vi "Lab Panel V3.2.vi"() -> ()   [LabVIEW 2013]
uses:
  <vilib>/Platform/TimedLoop/XDataNode/timing_clust.ctl
  <vilib>/Platform/TimedLoop/XDataNode/nitl_modes.ctl
  <vilib>/Platform/TimedLoop/XDataNode/wakeup.ctl
  Global 1.vi
  <vilib>/platform/TimedLoop/XDataNode/XDataNode.xnode
  <vilib>/Platform/TimedLoop/XDataNode/XDNodeRunTimeDep.lvlib
panel:
  out "TEMP update":bool
  out "AI update":bool
  in  "stop":bool
  in  "Tab Control 2":T1(tab)
  out "SIG LAB05-2":T2 {"PF" format="%.2f"; "AMPS" format="%.1f"}
  out "SIG LAB05-1":T2 {"PF" format="%.2f"; "AMPS" format="%.1f"}
  out "SIG LAB04-2":T2 {"PF" format="%.2f"; "AMPS" format="%.1f"}
  out "SIG LAB04-1":T2 {"PF" format="%.2f"; "AMPS" format="%.1f"}
  out "SIG LAB03-2":T2 {"PF" format="%.2f"; "AMPS" format="%.1f"}
  out "SIG LAB03-1":T2 {"PF" format="%.2f"; "AMPS" format="%.1f"}
  out "SIG LAB02-2":T2 {"PF" format="%.2f"; "AMPS" format="%.1f"}
  in  "RUN LAB01-1":bool
  in  "O/I  LAB05-1":bool
  in  "O/I  LAB05-2":bool
  in  "O/I  LAB04-1":bool
  in  "O/I  LAB04-2":bool
  in  "O/I  LAB02-1":bool
  in  "O/1  LAB02-2":bool
  in  "O/I  LAB01-2":bool
  in  "O/I  LAB01-1":bool
  in  "O/I  LAB03-1":bool
  in  "RUN LAB05-2":bool
  in  "RUN LAB05-1":bool
  in  "RUN LAB04-2":bool
  in  "RUN LAB04-1":bool
  in  "RUN LAB03-2":bool
  in  "RUN LAB03-1":bool
  in  "RUN LAB02-2":bool
  in  "RUN LAB02-1":bool
  in  "RUN LAB01-2":bool
  in  "SELECT LAB05-2":T3(radio)
  in  "SELECT LAB05-1":T3(radio)
  in  "SELECT LAB04-2":T3(radio)
  in  "SELECT LAB04-1":T3(radio)
  in  "SELECT LAB03-2":T3(radio)
  in  "SELECT LAB03-1":T3(radio)
  in  "SELECT LAB02-2":T3(radio)
  in  "SELECT LAB02-1":T3(radio)
  in  "SELECT LAB01-2":T3(radio)
  in  "SELECT LAB01-1":T3(radio)
  in  "O/I  LAB03-2":bool
  out "SIG LAB01-1":T2 {"PF" format="%.2f"; "AMPS" format="%.1f"}
  out "SIG LAB01-2":T2 {"PF" format="%.2f"; "AMPS" format="%.1f"}
  out "SIG LAB02-1":T2 {"PF" format="%.2f"; "AMPS" format="%.1f"}
  out "DISP LAB05-2":T4 {"MINS" format="%.2g"}
  out "DISP LAB05-1":T4 {"MINS" format="%.2g"}
  out "DISP LAB04-2":T4 {"MINS" format="%.2g"}
  out "DISP LAB04-1":T4 {"MINS" format="%.2g"}
  out "DISP LAB03-2":T4 {"MINS" format="%.2g"}
  out "DISP LAB03-1":T4 {"MINS" format="%.2g"}
  in  "SET LAB05-2":T5={"NAME"="", "DESCRIPTION"="", "CYCLES"=5.0, "T-RISE mins"=0.0, "T-RISE deg C"=0.0} {"CYCLES" min=5.0 step=1.0}
  in  "SET LAB05-1":T5={"NAME"="", "DESCRIPTION"="", "CYCLES"=5.0, "T-RISE mins"=0.0, "T-RISE deg C"=0.0} {"CYCLES" min=5.0 step=1.0}
  in  "SET LAB04-2":T5={"NAME"="", "DESCRIPTION"="", "CYCLES"=5.0, "T-RISE mins"=0.0, "T-RISE deg C"=0.0} {"CYCLES" min=5.0 step=1.0}
  in  "SET LAB04-1":T5={"NAME"="", "DESCRIPTION"="", "CYCLES"=5.0, "T-RISE mins"=0.0, "T-RISE deg C"=0.0} {"CYCLES" min=5.0 step=1.0}
  in  "SET LAB03-2":T5={"NAME"="", "DESCRIPTION"="", "CYCLES"=5.0, "T-RISE mins"=0.0, "T-RISE deg C"=0.0} {"CYCLES" min=5.0 step=1.0}
  in  "SET LAB03-1":T5={"NAME"="", "DESCRIPTION"="", "CYCLES"=5.0, "T-RISE mins"=0.0, "T-RISE deg C"=0.0} {"CYCLES" min=5.0 step=1.0}
  out "DISP LAB02-2":T4 {"MINS" format="%.2g"}
  out "DISP LAB02-1":T4 {"MINS" format="%.2g"}
  in  "SET LAB02-2":T5={"NAME"="", "DESCRIPTION"="", "CYCLES"=5.0, "T-RISE mins"=0.0, "T-RISE deg C"=0.0} {"CYCLES" min=5.0 step=1.0}
  in  "SET LAB02-1":T5={"NAME"="", "DESCRIPTION"="", "CYCLES"=5.0, "T-RISE mins"=0.0, "T-RISE deg C"=0.0} {"CYCLES" min=5.0 step=1.0}
  out "RESULT LAB05-2":bool
  out "RESULT LAB05-1":bool
  out "RESULT LAB04-2":bool
  out "RESULT LAB04-1":bool
  out "RESULT LAB03-2":bool
  out "RESULT LAB03-1":bool
  out "RESULT LAB02-2":bool
  out "RESULT LAB02-1":bool
  out "RESULT LAB01-2":bool
  out "RESULT LAB01-1":bool
  in  "SET LAB01-1":T5={"NAME"="", "DESCRIPTION"="", "CYCLES"=5.0, "T-RISE mins"=0.0, "T-RISE deg C"=0.0} {"CYCLES" min=5.0 step=1.0}
  in  "SET LAB01-2":T5={"NAME"="", "DESCRIPTION"="", "CYCLES"=5.0, "T-RISE mins"=0.0, "T-RISE deg C"=0.0} {"CYCLES" min=5.0 step=1.0}
  out "DISP LAB01-1":T4 {"MINS" format="%.2g"}
  out "DISP LAB01-2":T4 {"MINS" format="%.2f"}
  in  "Mail Report Error":errorcluster
  in  "MAIL SELECT":cluster{"Mail Notification":bool, "TO:":string}
  in  "Network Directory":path
  in  "JIG OFF TIME (S)":dbl=2.0 min=2.0 max=10.0 step=0.5 format="%.1g"
  in  "JIG ON TIME (S)":dbl=1.0 min=1.0 max=10.0 step=0.5 format="%.1g"
  out "FAIL LAB05-2":cluster{"LO":dbl, "HI":dbl}
  out "FAIL LAB05-1":cluster{"LO":dbl, "HI":dbl}
  out "FAIL LAB04-2":cluster{"LO":dbl, "HI":dbl}
  out "FAIL LAB04-1":cluster{"LO":dbl, "HI":dbl}
  out "FAIL LAB03-2":cluster{"LO":dbl, "HI":dbl}
  out "FAIL LAB03-1":cluster{"LO":dbl, "HI":dbl}
  out "FAIL LAB02-2":cluster{"LO":dbl, "HI":dbl}
  out "FAIL LAB02-1":cluster{"LO":dbl, "HI":dbl}
  out "FAIL LAB01-2":cluster{"LO":dbl, "HI":dbl}
  out "FAIL LAB01-1":cluster{"LO":dbl, "HI":dbl}
  out "TEMP START LAB05-2":cluster{"TL":dbl, "TN":dbl}
  out "TEMP START LAB04-2":cluster{"TL":dbl, "TN":dbl}
  out "TEMP START LAB03-2":cluster{"TL":dbl, "TN":dbl}
  out "TEMP START LAB02-2":cluster{"TL":dbl, "TN":dbl}
  out "TEMP START LAB01-2":cluster{"TL":dbl, "TN":dbl}
  out "TEMP START LAB05-1":cluster{"TL":dbl, "TN":dbl}
  out "TEMP START LAB04-1":cluster{"TL":dbl, "TN":dbl}
  out "TEMP START LAB03-1":cluster{"TL":dbl, "TN":dbl}
  out "TEMP START LAB02-1":cluster{"TL":dbl, "TN":dbl}
  out "TEMP START LAB01-1":cluster{"TL":dbl, "TN":dbl}
  out "JIG LAB01-1":bool
  out "JIG LAB01-2":bool
  out "JIG LAB02-1":bool
  out "JIG LAB02-2":bool
  out "JIG LAB03-1":bool
  out "JIG LAB03-2":bool
  out "JIG LAB04-1":bool
  out "JIG LAB04-2":bool
  out "JIG LAB05-1":bool
  out "JIG LAB05-2":bool
  out "CAL LAB01":T6 {"2 (TN) cal" min=0.0 step=0.01 format="%.2f"; "2 (TL) cal" min=0.0 step=0.01 format="%.2f"; "2 (PF) cal" min=0.0 step=0.01 format="%.2f"; "2 (V) cal" min=0.0 step=0.01 format="%.2f"; "2 (A) cal" min=0.0 step=0.01 format="%.2f"; "1 (TN) cal" min=0.0 step=0.01 format="%.2f"; "1 (TL) cal" min=0.0 step=0.01 format="%.2f"; "1 (PF) cal" min=0.0 step=0.01 format="%.2f"; "1 (V) cal" min=0.0 step=0.01 format="%.2f"; "1  (A) cal" min=0.0 step=0.01 format="%.2f"}
  out "CAL LAB03":T6 {"2 (TN) cal" min=0.0 step=0.01 format="%.2f"; "2 (TL) cal" min=0.0 step=0.01 format="%.2f"; "2 (PF) cal" min=0.0 step=0.01 format="%.2f"; "2 (V) cal" min=0.0 step=0.01 format="%.2f"; "2 (A) cal" min=0.0 step=0.01 format="%.2f"; "1 (TN) cal" min=0.0 step=0.01 format="%.2f"; "1 (TL) cal" min=0.0 step=0.01 format="%.2f"; "1 (PF) cal" min=0.0 step=0.01 format="%.2f"; "1 (V) cal" min=0.0 step=0.01 format="%.2f"; "1  (A) cal" min=0.0 step=0.01 format="%.2f"}
  out "CAL LAB02":T7 {"2 (TN) cal" min=0.0 step=0.01 format="%.2f"; "2 (TL) cal" min=0.0 step=0.01 format="%.2f"; "2 (PF) cal" min=0.0 step=0.01 format="%.2f"; "2 (V) cal" min=0.0 step=0.01 format="%.2f"; "2 (A) cal" min=0.0 step=0.01 format="%.2f"; "1 (TN) cal" min=0.0 step=0.01 format="%.2f"; "1 (TL) cal" min=0.0 step=0.01 format="%.2f"; "1 (PF) cal" min=0.0 step=0.01 format="%.2f"; "1 (V) cal" min=0.0 step=0.01 format="%.2f"; "1 (A) cal" min=0.0 step=0.01 format="%.2f"}
  out "CAL LAB05":T6 {"2 (TN) cal" min=0.0 step=0.01 format="%.2f"; "2 (TL) cal" min=0.0 step=0.01 format="%.2f"; "2 (PF) cal" min=0.0 step=0.01 format="%.2f"; "2 (V) cal" min=0.0 step=0.01 format="%.2f"; "2 (A) cal" min=0.0 step=0.01 format="%.2f"; "1 (TN) cal" min=0.0 step=0.01 format="%.2f"; "1 (TL) cal" min=0.0 step=0.01 format="%.2f"; "1 (PF) cal" min=0.0 step=0.01 format="%.2f"; "1 (V) cal" min=0.0 step=0.01 format="%.2f"; "1  (A) cal" min=0.0 step=0.01 format="%.2f"}
  out "CAL LAB04":T6 {"2 (TN) cal" min=0.0 step=0.01 format="%.2f"; "2 (TL) cal" min=0.0 step=0.01 format="%.2f"; "2 (PF) cal" min=0.0 step=0.01 format="%.2f"; "2 (V) cal" min=0.0 step=0.01 format="%.2f"; "2 (A) cal" min=0.0 step=0.01 format="%.2f"; "1 (TN) cal" min=0.0 step=0.01 format="%.2f"; "1 (TL) cal" min=0.0 step=0.01 format="%.2f"; "1 (PF) cal" min=0.0 step=0.01 format="%.2f"; "1 (V) cal" min=0.0 step=0.01 format="%.2f"; "1  (A) cal" min=0.0 step=0.01 format="%.2f"}
  out "calibration file error out":errorcluster
  in  "CALIBRATE":bool
  in  "MAIL SETTINGS":T8
  out "mail control":string
  out "MAIL REPORT":string
  out "stop2":bool
  in  "Tab Control":T9(tab)
  out "LAB01-2 (GRAPH)":dynamicdata(graph)
  out "LAB01-1 (GRAPH)":dynamicdata(graph)
  out "LAB02-2 (GRAPH)":dynamicdata(graph)
  out "LAB02-1 (GRAPH)":dynamicdata(graph)
  out "LAB03-2 (GRAPH)":dynamicdata(graph)
  out "LAB03-1 (GRAPH)":dynamicdata(graph)
  out "LAB04-2 (GRAPH)":dynamicdata(graph)
  out "LAB04-1 (GRAPH)":dynamicdata(graph)
  out "LAB05-2 (GRAPH)":dynamicdata(graph)
  out "LAB05-1 (GRAPH)":dynamicdata(graph)
  out "LAB05 TEMP":T10
  out "LAB04 TEMP":T10
  out "LAB02 TEMP":T10
  out "LAB01 TEMP":T10
  out "LAB03 TEMP":T10
  out "Analog Error Array":errorcluster[](array[cluster])
  out "AI loop time":dbl format="%.6g"
  out "loops":dbl
  in  "loop  delay(mS)":dbl
  out "on loops":dbl
  out "off loops":dbl
  out "jig cycle":dbl
  out "TDMS LAB01-1":refnum<k34>
  out "data file error":errorcluster
  out "TDMS LAB02-1":refnum<k34>
  out "TDMS LAB01-2":refnum<k34>
  out "TDMS LAB02-2":refnum<k34>
  out "TDMS LAB03-1":refnum<k34>
  out "TDMS LAB03-2":refnum<k34>
  out "TDMS LAB04-1":refnum<k34>
  out "TDMS LAB04-2":refnum<k34>
  out "TDMS LAB05-1":refnum<k34>
  out "TDMS LAB05-2":refnum<k34>
  # "LAB01"
  # "LAB02"
  # "LAB05"
  # "LAB03"
  # "LAB04"
  # "LAB01"
  # "LAB02"
  # "LAB03"
  # "LAB04"
  # "LAB05"
  # "JIG SET"
  # "Enter receipients address seperated by comma."
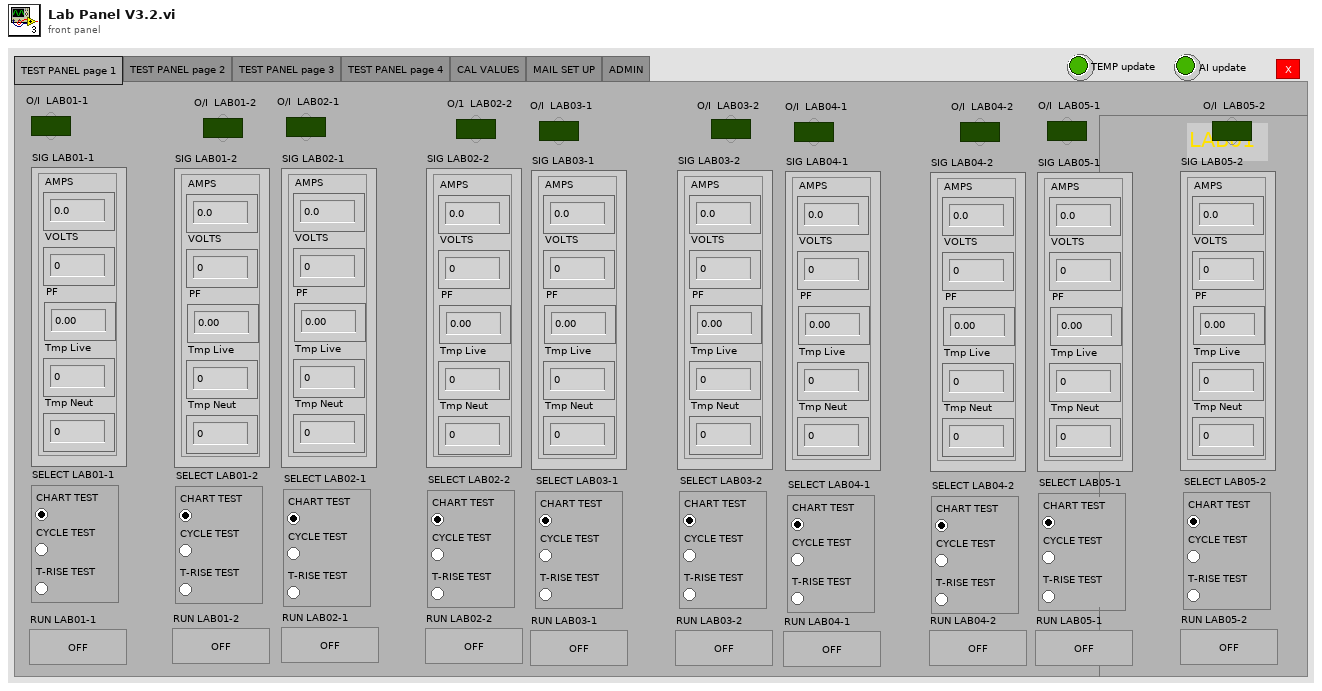
[diagram p1: front panel]
types:
  T1 = enum32{"TEST PANEL page 1", "TEST PANEL page 2", "TEST PANEL page 3", "TEST PANEL page 4", "CAL VALUES", "MAIL SET UP", "ADMIN"}
  T2 = cluster{"AMPS":dbl, "VOLTS":dbl, "PF":dbl, "Tmp Live":dbl, "Tmp Neut":dbl}
  T3 = enum32{"CHART TEST", "CYCLE TEST", "T-RISE TEST"}
  T4 = cluster{"CYCLE":dbl, "MINS":dbl, "STATUS":string}
  T5 = cluster{"NAME":string, "DESCRIPTION":string, "CYCLES":dbl, "T-RISE mins":dbl, "T-RISE deg C":dbl}
  T6 = cluster{"1  (A) cal":dbl, "1 (V) cal":dbl, "1 (PF) cal":dbl, "1 (TL) cal":dbl, "1 (TN) cal":dbl, "2 (A) cal":dbl, "2 (V) cal":dbl, "2 (PF) cal":dbl, "2 (TL) cal":dbl, "2 (TN) cal":dbl}
  T7 = cluster{"1 (A) cal":dbl, "1 (V) cal":dbl, "1 (PF) cal":dbl, "1 (TL) cal":dbl, "1 (TN) cal":dbl, "2 (A) cal":dbl, "2 (V) cal":dbl, "2 (PF) cal":dbl, "2 (TL) cal":dbl, "2 (TN) cal":dbl}
  T8 = cluster{"OUT SERVER ADDRESS":string, "FROM ACCOUNT":string, "USER NAME":string, "PASSWORD":string, "TEST MAIL":bool, "TEST MAIL STATUS":string, "mail error":errorcluster}
  T9 = enum32{"LAB01", "LAB02", "LAB03", "LAB04", "LAB05", "TEMPERATURE", "ERROR"}
  T10 = cluster{"T1 Live":dbl, "T1 Neut":dbl, "T2 Live":dbl, "T2 Neut":dbl, "ID":dbl, "ER":dbl}
  T11 = enum8{"Enabled", "Disabled", "Disabled and Grayed Out"}
  T12 = typedef "XDNodeRunTimeDep.lvlib/timing_clust.ctl" = cluster{"Expected End [f-1]":u64, "Actual End [f-1]":u64, "Finished Late? [f-1]":bool, "Expected End [i-1]":u64, "Actual End [i-1]":u64, "Finished Late? [i-1]":bool, "Expected Start [i]":u64, "Actual Start [i]":u64, "Expected Start [f]":u64, "Actual Start [f]":u64, "Source Name":string, "Structure Name":string, "Period":i64, "Deadline":i64, "Offset":i64, "Start":i64, "Priority":i32, "Timeout":i32, "Mode":T13, "Wakeup Reason":T14, "Error":errorcluster, "Source Type":string, "Secondary Source Type":string, "Global End Time":u64, "Global Start Time":u64, "Frame Duration":u64, "Iteration Duration":u64, "Assigned CPU":i32, "I/O Scan Engine Mode":u32}
  T13 = typedef "XDNodeRunTimeDep.lvlib/nitl_modes.ctl" = enum32{"No Change", "Process missed periods, maintain original phase", "Discard missed periods, maintain original phase", "Process missed periods, ignore original phase", "Discard missed periods, ignore original phase"}
  T14 = typedef "XDNodeRunTimeDep.lvlib/wakeup.ctl" = enum32{"Normal", "Aborted", "Asynchronous wakeup", "Timing source error", "Timed loop error", "Timeout"}
  T15 = enum16{"open", "open or create", "create or replace", "create", "open (read-only)"}
  T16 = enum16{"open", "replace", "create", "open or create", "replace or create", "replace or create with confirmation"}
  T17 = cluster{"SET LAB01-1":cluster{"NAME":string, "DESCRIPTION":string, "CYCLES":dbl, "T-RISE mins":dbl, "T-RISE deg C":dbl}, "SET LAB01-2":cluster{"NAME":string, "DESCRIPTION":string, "CYCLES":dbl, "T-RISE mins":dbl, "T-RISE deg C":dbl}, "SET LAB02-1":cluster{"NAME":string, "DESCRIPTION":string, "CYCLES":dbl, "T-RISE mins":dbl, "T-RISE deg C":dbl}, "SET LAB02-2":cluster{"NAME":string, "DESCRIPTION":string, "CYCLES":dbl, "T-RISE mins":dbl, "T-RISE deg C":dbl}, "SET LAB03-1":cluster{"NAME":string, "DESCRIPTION":string, "CYCLES":dbl, "T-RISE mins":dbl, "T-RISE deg C":dbl}, "SET LAB03-2":cluster{"NAME":string, "DESCRIPTION":string, "CYCLES":dbl, "T-RISE mins":dbl, "T-RISE deg C":dbl}, "SET LAB04-1":cluster{"NAME":string, "DESCRIPTION":string, "CYCLES":dbl, "T-RISE mins":dbl, "T-RISE deg C":dbl}, "SET LAB04-2":cluster{"NAME":string, "DESCRIPTION":string, "CYCLES":dbl, "T-RISE mins":dbl, "T-RISE deg C":dbl}, "SET LAB05-1":cluster{"NAME":string, "DESCRIPTION":string, "CYCLES":dbl, "T-RISE mins":dbl, "T-RISE deg C":dbl}, "SET LAB05-2":cluster{"NAME":string, "DESCRIPTION":string, "CYCLES":dbl, "T-RISE mins":dbl, "T-RISE deg C":dbl}, "Network Directory":path}
  T18 = cluster{"MAIL SETTINGS":cluster{"OUT SERVER ADDRESS":string, "FROM ACCOUNT":string, "USER NAME":string, "PASSWORD":string, "TEST MAIL":bool, "TEST MAIL STATUS":string, "mail error":errorcluster}, "MAIL SELECT":cluster{"Mail Notification":bool, "TO:":string}}
  T19 = cluster{"T1":dbl, "T2":dbl, "T3":dbl, "T4":dbl, "ID":dbl, "ER":dbl}
  T20 = cluster{"LAB01-1 (A)":dbl, "LAB01-1 (V)":dbl, "LAB01-1 (PF)":dbl, "LAB01-2 (A)":dbl, "LAB01-2 (V)":dbl, "LAB01-2 (PF)":dbl}
  T21 = cluster{"LAB02-1 (A)":dbl, "LAB02-1 (V)":dbl, "LAB02-1 (PF)":dbl, "LAB02-2 (A)":dbl, "LAB02-2 (V)":dbl, "LAB02-2 (PF)":dbl}
  T22 = cluster{"LAB03-1 (A)":dbl, "LAB03-1 (V)":dbl, "LAB03-1 (PF)":dbl, "LAB03-2 (A)":dbl, "LAB03-2 (V)":dbl, "LAB03-2 (PF)":dbl}
  T23 = cluster{"LAB04-1 (A)":dbl, "LAB04-1 (V)":dbl, "LAB04-1 (PF)":dbl, "LAB04-2 (A)":dbl, "LAB04-2 (V)":dbl, "LAB04-2 (PF)":dbl}
  T24 = cluster{"LAB05-1 (A)":dbl, "LAB05-1 (V)":dbl, "LAB05-1 (PF)":dbl, "LAB05-2 (A)":dbl, "LAB05-2 (V)":dbl, "LAB05-2 (PF)":dbl}
  T25 = cluster{"FAIL LAB01-1":cluster{"LO":dbl, "HI":dbl}, "SIG LAB01-1":cluster{"AMPS":dbl, "VOLTS":dbl, "PF":dbl, "Tmp Live":dbl, "Tmp Neut":dbl}, "TEMP START LAB01-1":cluster{"TL":dbl, "TN":dbl}, "DISP LAB01-1":cluster{"CYCLE":dbl, "MINS":dbl, "STATUS":string}, "SET LAB01-1":cluster{"NAME":string, "DESCRIPTION":string, "CYCLES":dbl, "T-RISE mins":dbl, "T-RISE deg C":dbl}, "TDMS LAB01-1":refnum<k34>}
  T26 = cluster{"FAIL LAB01-2":cluster{"LO":dbl, "HI":dbl}, "SIG LAB01-2":cluster{"AMPS":dbl, "VOLTS":dbl, "PF":dbl, "Tmp Live":dbl, "Tmp Neut":dbl}, "TEMP START LAB01-2":cluster{"TL":dbl, "TN":dbl}, "DISP LAB01-2":cluster{"CYCLE":dbl, "MINS":dbl, "STATUS":string}, "SET LAB01-2":cluster{"NAME":string, "DESCRIPTION":string, "CYCLES":dbl, "T-RISE mins":dbl, "T-RISE deg C":dbl}, "TDMS LAB01-2":refnum<k34>}
  T27 = cluster{"FAIL LAB02-1":cluster{"LO":dbl, "HI":dbl}, "SIG LAB02-1":cluster{"AMPS":dbl, "VOLTS":dbl, "PF":dbl, "Tmp Live":dbl, "Tmp Neut":dbl}, "TEMP START LAB02-1":cluster{"TL":dbl, "TN":dbl}, "DISP LAB02-1":cluster{"CYCLE":dbl, "MINS":dbl, "STATUS":string}, "SET LAB02-1":cluster{"NAME":string, "DESCRIPTION":string, "CYCLES":dbl, "T-RISE mins":dbl, "T-RISE deg C":dbl}, "TDMS LAB02-1":refnum<k34>}
  T28 = cluster{"FAIL LAB02-2":cluster{"LO":dbl, "HI":dbl}, "SIG LAB02-2":cluster{"AMPS":dbl, "VOLTS":dbl, "PF":dbl, "Tmp Live":dbl, "Tmp Neut":dbl}, "TEMP START LAB02-2":cluster{"TL":dbl, "TN":dbl}, "DISP LAB02-2":cluster{"CYCLE":dbl, "MINS":dbl, "STATUS":string}, "SET LAB02-2":cluster{"NAME":string, "DESCRIPTION":string, "CYCLES":dbl, "T-RISE mins":dbl, "T-RISE deg C":dbl}, "TDMS LAB02-2":refnum<k34>}
  T29 = cluster{"FAIL LAB03-1":cluster{"LO":dbl, "HI":dbl}, "SIG LAB03-1":cluster{"AMPS":dbl, "VOLTS":dbl, "PF":dbl, "Tmp Live":dbl, "Tmp Neut":dbl}, "TEMP START LAB03-1":cluster{"TL":dbl, "TN":dbl}, "DISP LAB03-1":cluster{"CYCLE":dbl, "MINS":dbl, "STATUS":string}, "SET LAB03-1":cluster{"NAME":string, "DESCRIPTION":string, "CYCLES":dbl, "T-RISE mins":dbl, "T-RISE deg C":dbl}, "TDMS LAB03-1":refnum<k34>}
  T30 = cluster{"FAIL LAB03-2":cluster{"LO":dbl, "HI":dbl}, "SIG LAB03-2":cluster{"AMPS":dbl, "VOLTS":dbl, "PF":dbl, "Tmp Live":dbl, "Tmp Neut":dbl}, "TEMP START LAB03-2":cluster{"TL":dbl, "TN":dbl}, "DISP LAB03-2":cluster{"CYCLE":dbl, "MINS":dbl, "STATUS":string}, "SET LAB03-2":cluster{"NAME":string, "DESCRIPTION":string, "CYCLES":dbl, "T-RISE mins":dbl, "T-RISE deg C":dbl}, "TDMS LAB03-2":refnum<k34>}
  T31 = cluster{"FAIL LAB04-1":cluster{"LO":dbl, "HI":dbl}, "SIG LAB04-1":cluster{"AMPS":dbl, "VOLTS":dbl, "PF":dbl, "Tmp Live":dbl, "Tmp Neut":dbl}, "TEMP START LAB04-1":cluster{"TL":dbl, "TN":dbl}, "DISP LAB04-1":cluster{"CYCLE":dbl, "MINS":dbl, "STATUS":string}, "SET LAB04-1":cluster{"NAME":string, "DESCRIPTION":string, "CYCLES":dbl, "T-RISE mins":dbl, "T-RISE deg C":dbl}, "TDMS LAB04-1":refnum<k34>}
  T32 = cluster{"FAIL LAB04-2":cluster{"LO":dbl, "HI":dbl}, "SIG LAB04-2":cluster{"AMPS":dbl, "VOLTS":dbl, "PF":dbl, "Tmp Live":dbl, "Tmp Neut":dbl}, "TEMP START LAB04-2":cluster{"TL":dbl, "TN":dbl}, "DISP LAB04-2":cluster{"CYCLE":dbl, "MINS":dbl, "STATUS":string}, "SET LAB04-2":cluster{"NAME":string, "DESCRIPTION":string, "CYCLES":dbl, "T-RISE mins":dbl, "T-RISE deg C":dbl}, "TDMS LAB04-2":refnum<k34>}
  T33 = cluster{"FAIL LAB05-1":cluster{"LO":dbl, "HI":dbl}, "SIG LAB05-1":cluster{"AMPS":dbl, "VOLTS":dbl, "PF":dbl, "Tmp Live":dbl, "Tmp Neut":dbl}, "TEMP START LAB05-1":cluster{"TL":dbl, "TN":dbl}, "DISP LAB05-1":cluster{"CYCLE":dbl, "MINS":dbl, "STATUS":string}, "SET LAB05-1":cluster{"NAME":string, "DESCRIPTION":string, "CYCLES":dbl, "T-RISE mins":dbl, "T-RISE deg C":dbl}, "TDMS LAB05-1":refnum<k34>}
  T34 = cluster{"FAIL LAB05-2":cluster{"LO":dbl, "HI":dbl}, "SIG LAB05-2":cluster{"AMPS":dbl, "VOLTS":dbl, "PF":dbl, "Tmp Live":dbl, "Tmp Neut":dbl}, "TEMP START LAB05-2":cluster{"TL":dbl, "TN":dbl}, "DISP LAB05-2":cluster{"CYCLE":dbl, "MINS":dbl, "STATUS":string}, "SET LAB05-2":cluster{"NAME":string, "DESCRIPTION":string, "CYCLES":dbl, "T-RISE mins":dbl, "T-RISE deg C":dbl}, "TDMS LAB05-2":refnum<k34>}
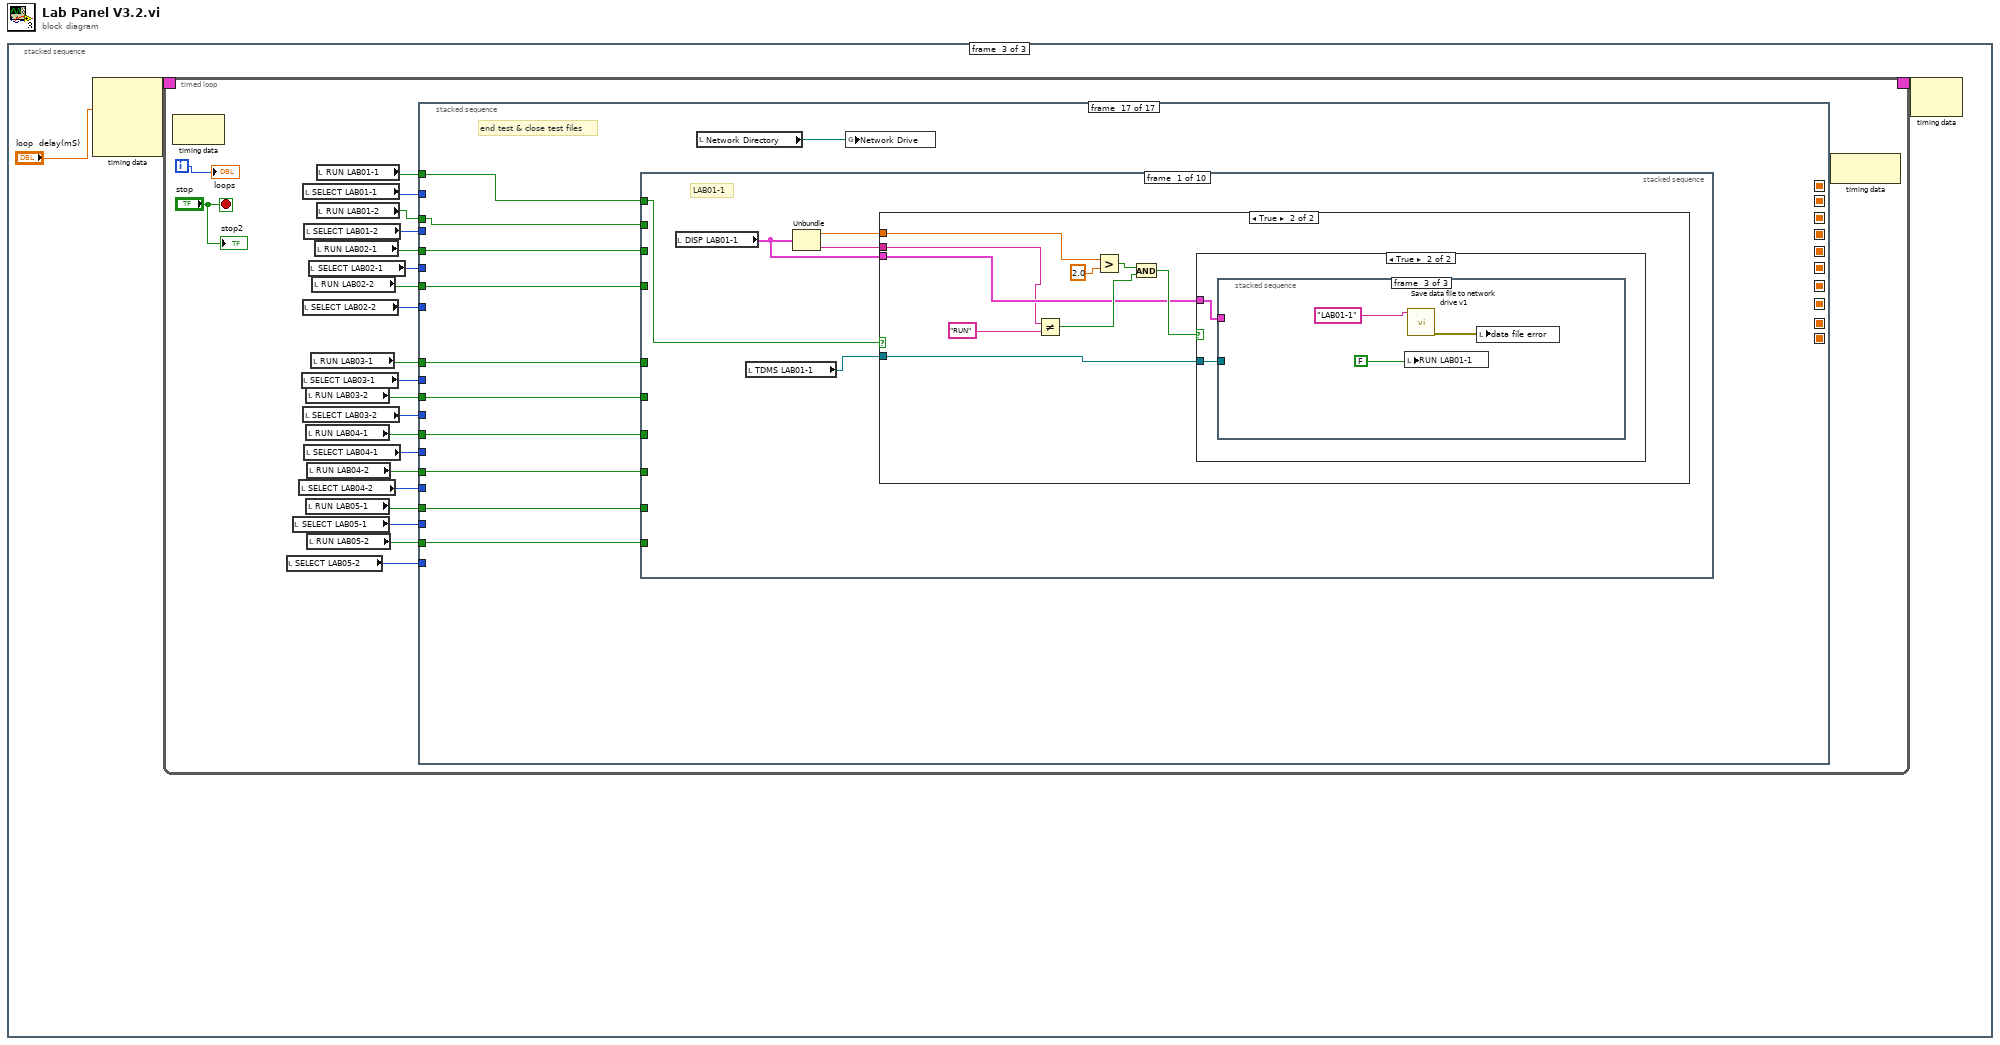
[diagram p0: block diagram]
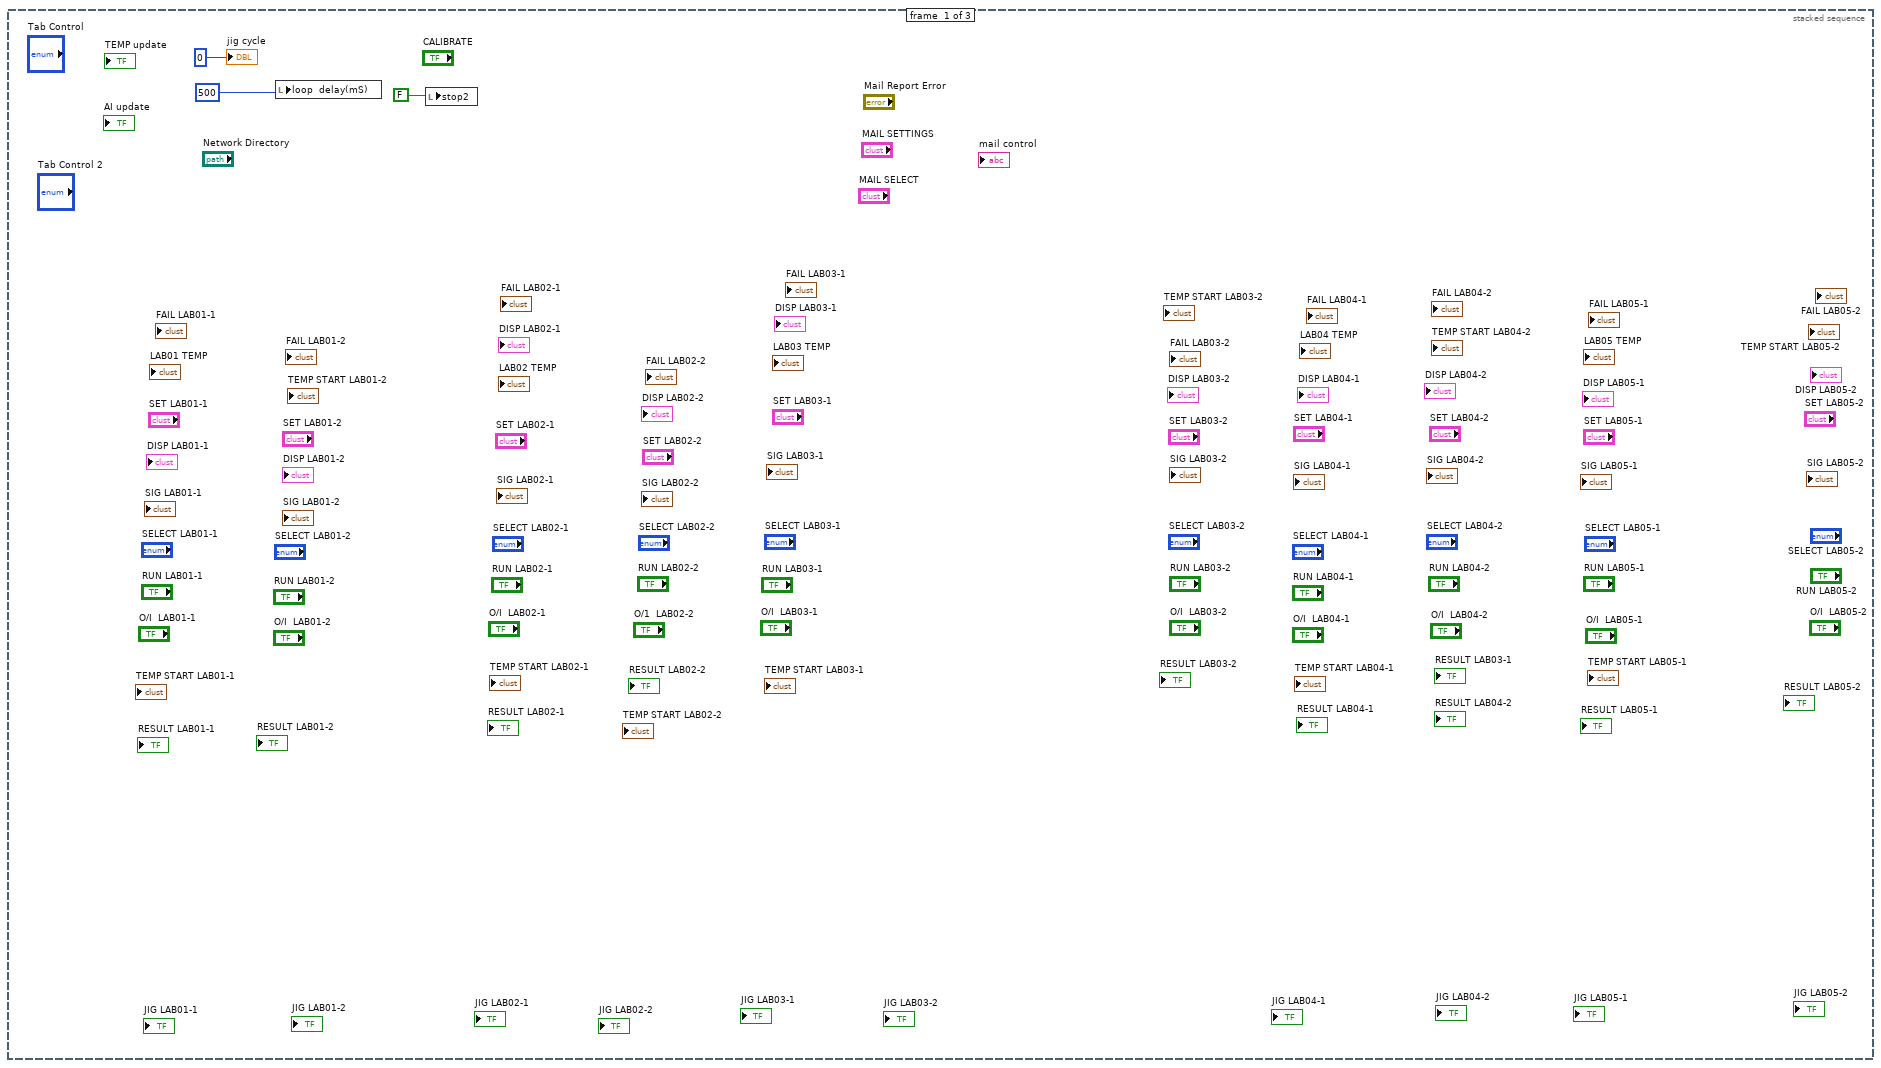
[diagram p2: hidden frame]
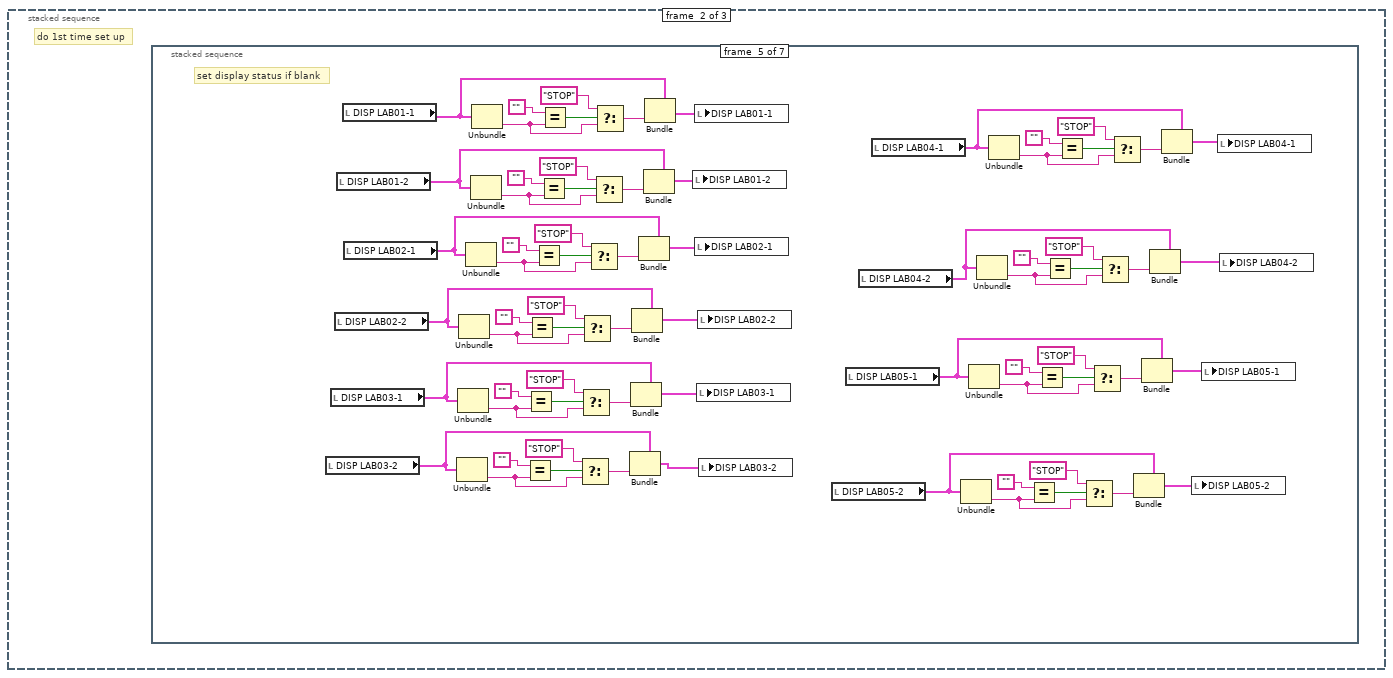
[diagram p3: hidden frame]
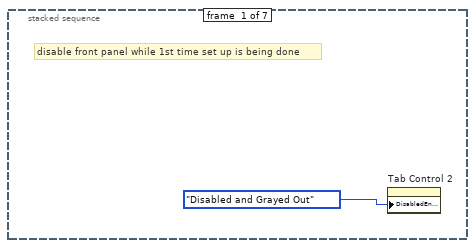
[diagram p4: hidden frame]
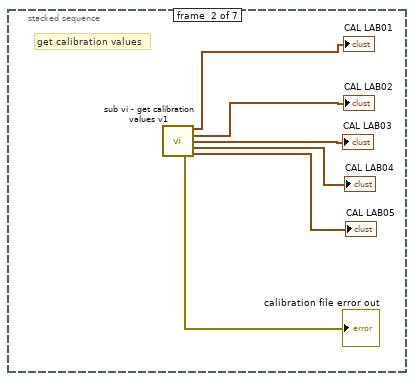
[diagram p5: hidden frame]
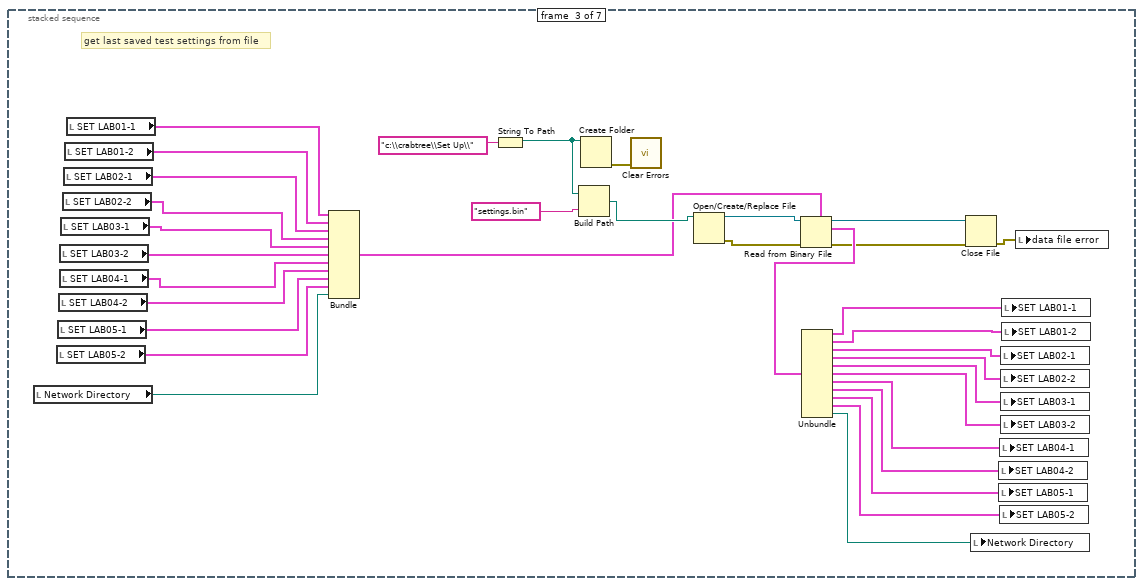
[diagram p6: hidden frame]
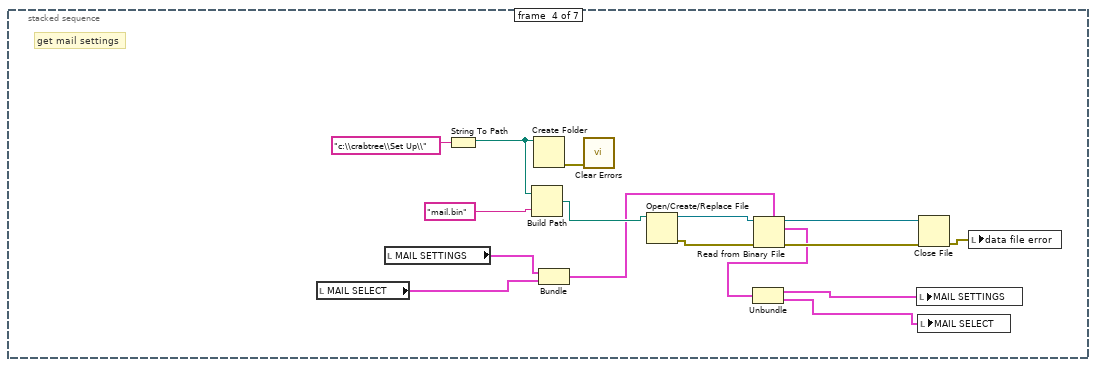
[diagram p7: hidden frame]
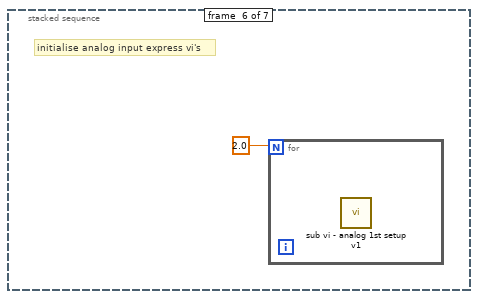
[diagram p8: hidden frame]
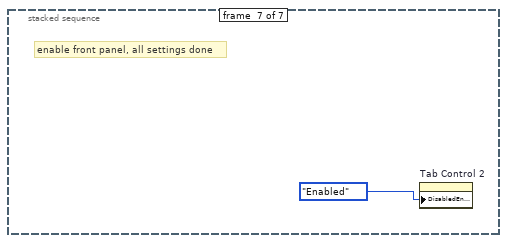
[diagram p9: hidden frame]
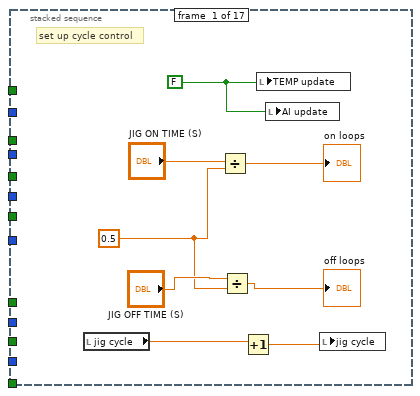
[diagram p10: hidden frame]
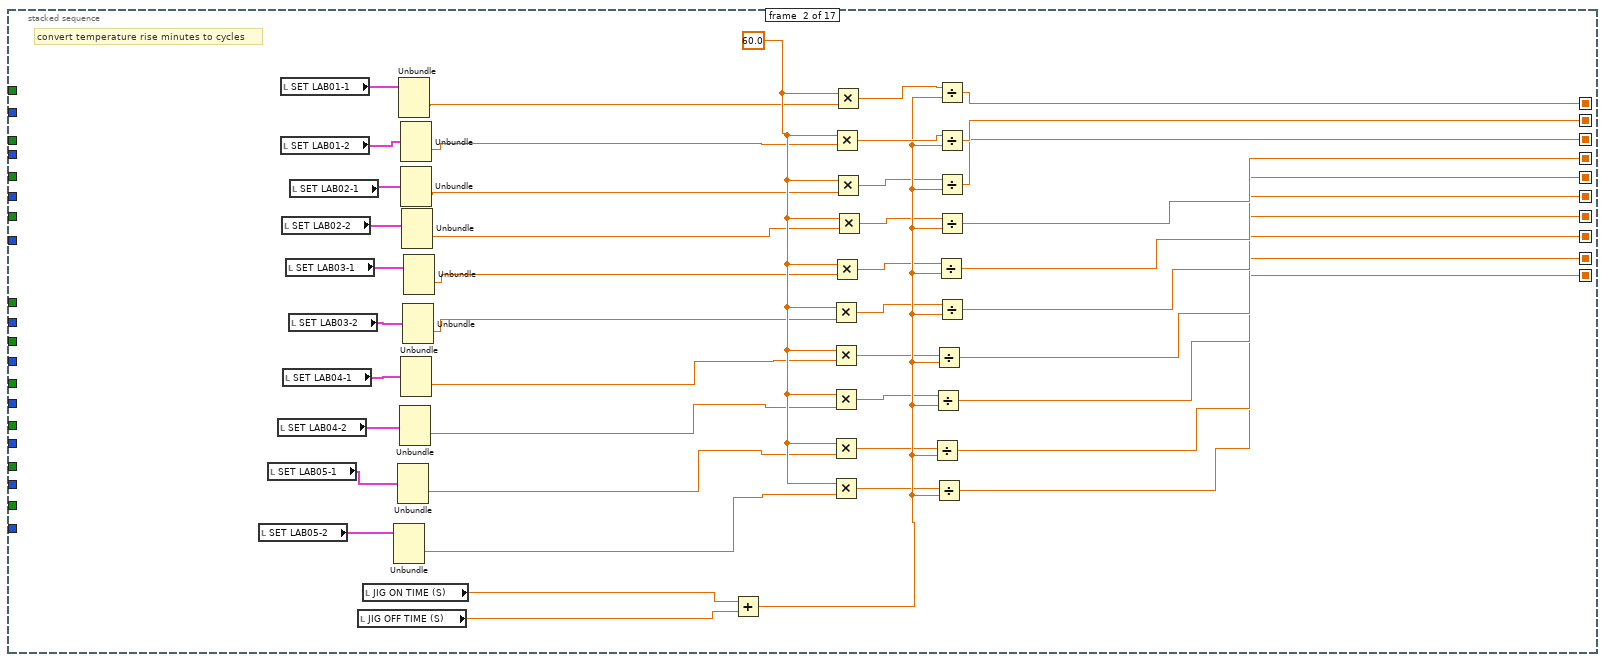
[diagram p11: hidden frame]
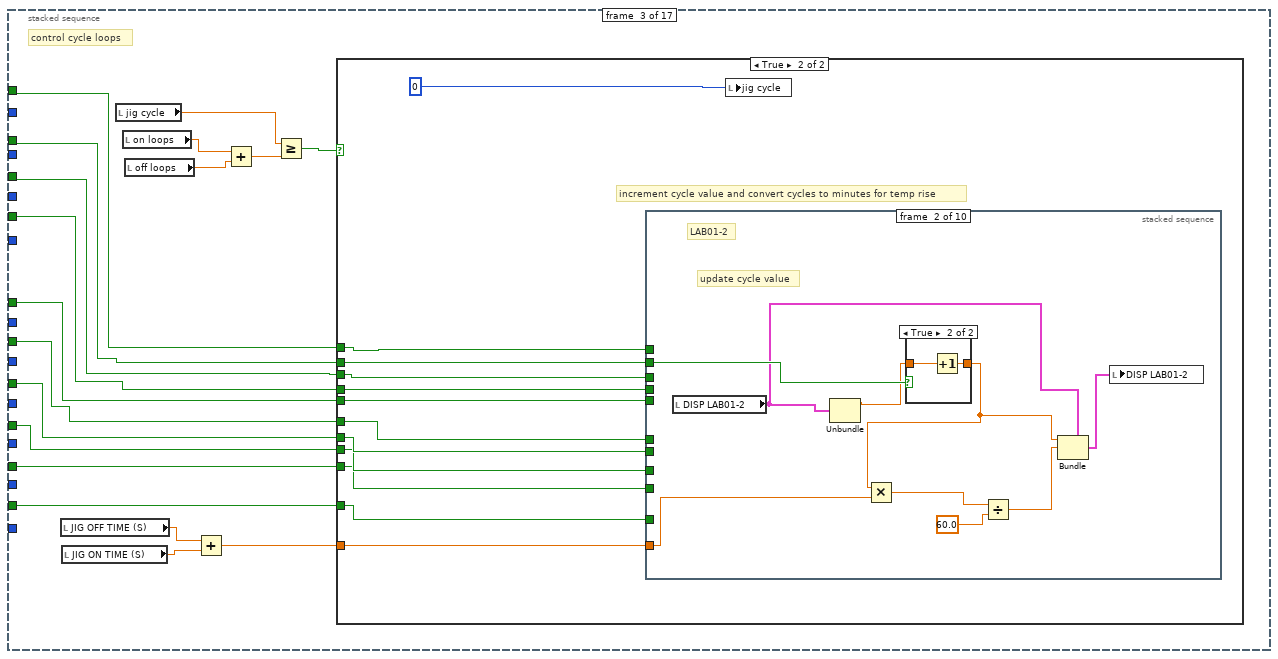
[diagram p12: hidden frame]
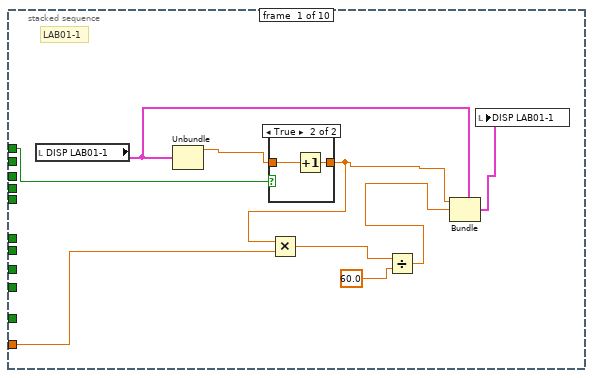
[diagram p14: hidden frame]
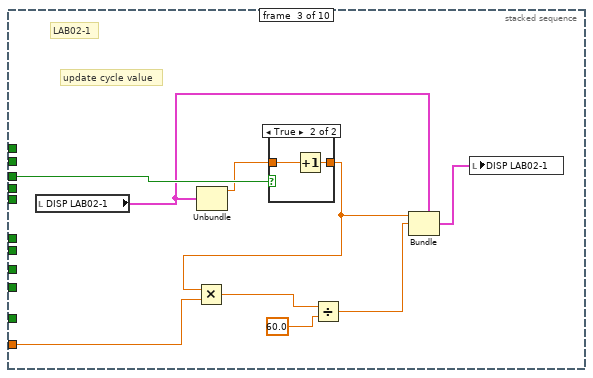
[diagram p17: hidden frame]
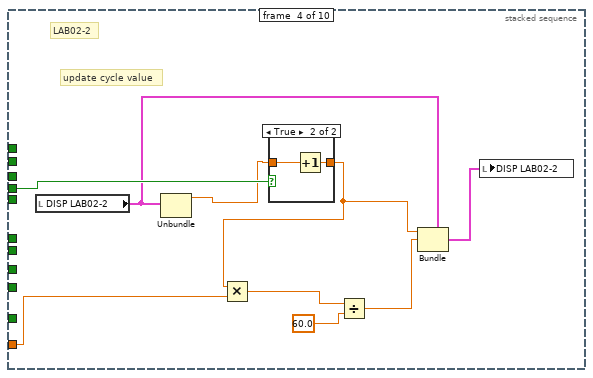
[diagram p19: hidden frame]
diagram:
  n1 = stacked-sequence {
    frame #0 {
      n2 = local write "loop  delay(mS)"(500) -> ()
      n3 = local write "stop2"(FALSE) -> ()
      "jig cycle" <- 0
    }
    frame #1 {
      # "do 1st time set up"
      n4 = stacked-sequence {
        frame #0 {
          # "disable front panel while 1st time set up is being done"
          n5 = property on="Tab Control 2" class="TabCtl (strict)"("DisabledEnum"=T11."Disabled and Grayed Out" ("Disabled")) -> ()  [unwired: 2 in, 2 out]
        }
        frame #1 {
          # "get calibration values"
          n6 = call "sub vi - get calibration values v1.vi"() -> ("LAB01 (CAL)"=→"CAL LAB01":T6, "LAB02 (CAL)"=→"CAL LAB02":T7, "LAB03 (CAL)"=→"CAL LAB03":T6, "LAB04 (CAL)"=→"CAL LAB04":T6, "calibration file error out"=→"calibration file error out":errorcluster, "LAB05 (CAL)"=→"CAL LAB05":T6)  [unwired: 10 in]
        }
        frame #2 {
          # "get last saved test settings from file"
          n7 = local read "Network Directory"() -> (w40:path)
          n8 = local read "SET LAB05-2"() -> (w41:T5)
          n9 = local read "SET LAB05-1"() -> (w42:T5)
          n10 = local read "SET LAB04-2"() -> (w43:T5)
          n11 = local read "SET LAB03-2"() -> (w39:T5)
          n12 = local read "SET LAB04-1"() -> (w44:T5)
          n13 = local read "SET LAB03-1"() -> (w38:T5)
          n14 = local read "SET LAB02-2"() -> (w37:T5)
          n15 = local read "SET LAB02-1"() -> (w36:T5)
          n16 = local read "SET LAB01-2"() -> (w35:T5)
          n17 = local read "SET LAB01-1"() -> (w34:T5)
          n18 = Bundle("SET LAB01-1"=w34, "SET LAB01-2"=w35, "SET LAB02-1"=w36, "SET LAB02-2"=w37, "SET LAB03-1"=w38, "SET LAB03-2"=w39, "SET LAB04-1"=w44, "SET LAB04-2"=w43, "SET LAB05-1"=w42, "SET LAB05-2"=w41, "Network Directory"=w40) -> (w27:T17)  [unwired: 1 in]
          n19 = String To Path(string="c:\\crabtree\\Set Up\\") -> (path=w31:path)
          n20 = Build Path(base path=w31, name or relative path="settings.bin") -> (appended path=w29:path)
          n21 = Create Folder(path (use dialog)=w31) -> (error out=w33:errorcluster)  [unwired: 2 in, 2 out]
          n22 = call <vilib>:"Clear Errors.vi"("error in (no error)"=w33) -> ()  [unwired: 6 in, 1 out]
          n23 = Open/Create/Replace File(file path (use dialog)=w29) -> (refnum out=w26:refnum<file>, error out=w28:errorcluster)  [unwired: 5 in, 1 out]
          n24 = Read from Binary File(5:w27, 8:w28, 11:w26) -> (0:w23:errorcluster, 2:w25:T17, 3:w24:refnum<file>)  [unwired: 3 in, 1 out]
          n25 = Unbundle(w25) -> ("SET LAB01-1"=w21:T5, "SET LAB01-2"=w20:T5, "SET LAB02-1"=w19:T5, "SET LAB02-2"=w18:T5, "SET LAB03-1"=w17:T5, "SET LAB03-2"=w16:T5, "SET LAB04-1"=w15:T5, "SET LAB04-2"=w14:T5, "SET LAB05-1"=w13:T5, "SET LAB05-2"=w12:T5, "Network Directory"=w11:path)
          n26 = Close File(refnum=w24, error in=w23) -> (error out=w22:errorcluster)  [unwired: 1 out]
          n27 = local write "Network Directory"(w11) -> ()
          n28 = local write "SET LAB04-2"(w14) -> ()
          n29 = local write "SET LAB05-1"(w13) -> ()
          n30 = local write "SET LAB04-1"(w15) -> ()
          n31 = local write "SET LAB05-2"(w12) -> ()
          n32 = local write "SET LAB02-1"(w19) -> ()
          n33 = local write "SET LAB02-2"(w18) -> ()
          n34 = local write "SET LAB03-1"(w17) -> ()
          n35 = local write "SET LAB03-2"(w16) -> ()
          n36 = local write "SET LAB01-1"(w21) -> ()
          n37 = local write "SET LAB01-2"(w20) -> ()
          n38 = local write "data file error"(w22) -> ()
        }
        frame #3 {
          # "get mail settings"
          n39 = local read "MAIL SELECT"() -> (w46:cluster{"Mail Notification":bool, "TO:":string})
          n40 = local read "MAIL SETTINGS"() -> (w50:T8)
          n41 = String To Path(string="c:\\crabtree\\Set Up\\") -> (path=w58:path)
          n42 = Build Path(base path=w58, name or relative path="mail.bin") -> (appended path=w56:path)
          n43 = Create Folder(path (use dialog)=w58) -> (error out=w60:errorcluster)  [unwired: 2 in, 2 out]
          n44 = Bundle("MAIL SETTINGS"=w50, "MAIL SELECT"=w46) -> (w49:T18)  [unwired: 1 in]
          n45 = call <vilib>:"Clear Errors.vi"("error in (no error)"=w60) -> ()  [unwired: 6 in, 1 out]
          n46 = Open/Create/Replace File(file path (use dialog)=w56) -> (refnum out=w54:refnum<file>, error out=w55:errorcluster)  [unwired: 5 in, 1 out]
          n47 = Read from Binary File(5:w49, 8:w55, 11:w54) -> (0:w52:errorcluster, 2:w48:T18, 3:w53:refnum<file>)  [unwired: 3 in, 1 out]
          n48 = Unbundle(w48) -> ("MAIL SETTINGS"=w47:T8, "MAIL SELECT"=w45:cluster{"Mail Notification":bool, "TO:":string})
          n49 = local write "MAIL SETTINGS"(w47) -> ()
          n50 = local write "MAIL SELECT"(w45) -> ()
          n51 = Close File(refnum=w53, error in=w52) -> (error out=w51:errorcluster)  [unwired: 1 out]
          n52 = local write "data file error"(w51) -> ()
        }
        frame #4 {
          # "set display status if blank"
          n53 = local read "DISP LAB03-2"() -> (w90:T4)
          n54 = local read "DISP LAB03-1"() -> (w97:T4)
          n55 = local read "DISP LAB02-2"() -> (w104:T4)
          n56 = local read "DISP LAB01-2"() -> (w117:T4)
          n57 = local read "DISP LAB01-1"() -> (w126:T4)
          n58 = local read "DISP LAB02-1"() -> (w111:T4)
          n59 = Unbundle(w90) -> ("STATUS"=w92:string)  [unwired: 2 out]
          n60 = Unbundle(w97) -> ("STATUS"=w99:string)  [unwired: 2 out]
          n61 = Unbundle(w104) -> ("STATUS"=w106:string)  [unwired: 2 out]
          n62 = Unbundle(w111) -> ("STATUS"=w113:string)  [unwired: 2 out]
          n63 = Unbundle(w117) -> ("STATUS"=w120:string)  [unwired: 2 out]
          n64 = Unbundle(w126) -> ("STATUS"=w127:string)  [unwired: 2 out]
          n65 = Equal?(x="", y=w92) -> (x = y?=w94:bool)
          n66 = Equal?(x="", y=w99) -> (x = y?=w101:bool)
          n67 = Equal?(x="", y=w106) -> (x = y?=w108:bool)
          n68 = Equal?(x="", y=w113) -> (x = y?=w115:bool)
          n69 = Equal?(x="", y=w120) -> (x = y?=w122:bool)
          n70 = Equal?(x="", y=w127) -> (x = y?=w129:bool)
          n71 = Select(t="STOP", s=w94, f=w92) -> (s? t:f=w91:string)
          n72 = Select(t="STOP", s=w101, f=w99) -> (s? t:f=w98:string)
          n73 = Select(t="STOP", s=w108, f=w106) -> (s? t:f=w105:string)
          n74 = Select(t="STOP", s=w115, f=w113) -> (s? t:f=w112:string)
          n75 = Select(t="STOP", s=w122, f=w120) -> (s? t:f=w119:string)
          n76 = Select(t="STOP", s=w129, f=w127) -> (s? t:f=w125:string)
          n77 = Bundle(cluster=w90, "STATUS"=w91) -> (w89:T4)  [unwired: 2 in]
          n78 = Bundle(cluster=w97, "STATUS"=w98) -> (w96:T4)  [unwired: 2 in]
          n79 = Bundle(cluster=w104, "STATUS"=w105) -> (w103:T4)  [unwired: 2 in]
          n80 = Bundle(cluster=w111, "STATUS"=w112) -> (w110:T4)  [unwired: 2 in]
          n81 = Bundle(cluster=w117, "STATUS"=w119) -> (w118:T4)  [unwired: 2 in]
          n82 = Bundle(cluster=w126, "STATUS"=w125) -> (w124:T4)  [unwired: 2 in]
          n83 = local write "DISP LAB01-2"(w118) -> ()
          n84 = local write "DISP LAB01-1"(w124) -> ()
          n85 = local write "DISP LAB02-1"(w110) -> ()
          n86 = local write "DISP LAB03-1"(w96) -> ()
          n87 = local write "DISP LAB02-2"(w103) -> ()
          n88 = local write "DISP LAB03-2"(w89) -> ()
          n89 = local read "DISP LAB05-2"() -> (w62:T4)
          n90 = local read "DISP LAB05-1"() -> (w69:T4)
          n91 = local read "DISP LAB04-2"() -> (w71:T4)
          n92 = local read "DISP LAB04-1"() -> (w73:T4)
          n93 = Unbundle(w62) -> ("STATUS"=w64:string)  [unwired: 2 out]
          n94 = Unbundle(w69) -> ("STATUS"=w75:string)  [unwired: 2 out]
          n95 = Unbundle(w71) -> ("STATUS"=w80:string)  [unwired: 2 out]
          n96 = Unbundle(w73) -> ("STATUS"=w85:string)  [unwired: 2 out]
          n97 = Equal?(x="", y=w64) -> (x = y?=w66:bool)
          n98 = Equal?(x="", y=w75) -> (x = y?=w77:bool)
          n99 = Equal?(x="", y=w80) -> (x = y?=w82:bool)
          n100 = Equal?(x="", y=w85) -> (x = y?=w87:bool)
          n101 = Select(t="STOP", s=w66, f=w64) -> (s? t:f=w63:string)
          n102 = Select(t="STOP", s=w77, f=w75) -> (s? t:f=w74:string)
          n103 = Select(t="STOP", s=w82, f=w80) -> (s? t:f=w79:string)
          n104 = Select(t="STOP", s=w87, f=w85) -> (s? t:f=w84:string)
          n105 = Bundle(cluster=w62, "STATUS"=w63) -> (w61:T4)  [unwired: 2 in]
          n106 = Bundle(cluster=w69, "STATUS"=w74) -> (w68:T4)  [unwired: 2 in]
          n107 = Bundle(cluster=w71, "STATUS"=w79) -> (w70:T4)  [unwired: 2 in]
          n108 = Bundle(cluster=w73, "STATUS"=w84) -> (w72:T4)  [unwired: 2 in]
          n109 = local write "DISP LAB05-2"(w61) -> ()
          n110 = local write "DISP LAB05-1"(w68) -> ()
          n111 = local write "DISP LAB04-1"(w72) -> ()
          n112 = local write "DISP LAB04-2"(w70) -> ()
        }
        frame #5 {
          # "initialise analog input express vi's"
          n113 = for {
            N: 2.0 -> [_]
            n114 = call "sub vi - analog 1st setup v1.vi"() -> ()  [unwired: 11 in, 5 out]
          }
        }
        frame #6 {
          # "enable front panel, all settings done"
          n115 = property on="Tab Control 2" class="TabCtl (strict)"("DisabledEnum"=T11."Enabled" ("Disabled")) -> ()  [unwired: 2 in, 2 out]
        }
      }
    }
    frame #2 {
      n116 = node-c288("loop  delay(mS)") -> (w135:T12)  [unwired: 3 in]
      n117 = timed-loop {
        timing: w135 -> [_]
        timing-out: [_] -> w134
        i -> [w157]
        stop <- "stop" stop-if-true
        n118 = node-c288() -> ()  [unwired: 1 in, 1 out]
        n119 = local read "SELECT LAB05-2"() -> (w137:T3)
        n120 = local read "SELECT LAB05-1"() -> (w138:T3)
        n121 = local read "SELECT LAB04-2"() -> (w139:T3)
        n122 = local read "SELECT LAB03-1"() -> (w142:T3)
        n123 = local read "SELECT LAB02-2"() -> (w143:T3)
        n124 = local read "SELECT LAB01-1"() -> (w146:T3)
        n125 = local read "SELECT LAB03-2"() -> (w141:T3)
        n126 = local read "SELECT LAB01-2"() -> (w145:T3)
        n127 = local read "SELECT LAB04-1"() -> (w140:T3)
        n128 = local read "RUN LAB03-2"() -> (w151:bool)
        n129 = local read "RUN LAB04-1"() -> (w150:bool)
        n130 = local read "RUN LAB05-1"() -> (w148:bool)
        n131 = local read "RUN LAB04-2"() -> (w149:bool)
        n132 = local read "RUN LAB05-2"() -> (w147:bool)
        n133 = local read "SELECT LAB02-1"() -> (w144:T3)
        n134 = local read "RUN LAB03-1"() -> (w152:bool)
        n135 = local read "RUN LAB02-2"() -> (w153:bool)
        n136 = local read "RUN LAB02-1"() -> (w154:bool)
        n137 = local read "RUN LAB01-1"() -> (w156:bool)
        n138 = local read "RUN LAB01-2"() -> (w155:bool)
        n139 = stacked-sequence {
          seq-local: [_ w209 _ _ _ _ _ _ _ _ _ _ _ _ _ _ _] -> [_ _ _ _ _ w1701 _ _ _ _ _ _ _ _ _ _ _]
          seq-local: [_ w208 _ _ _ _ _ _ _ _ _ _ _ _ _ _ _] -> [_ _ _ _ _ w1700 _ _ _ _ _ _ _ _ _ _ _]
          seq-local: [_ w195 _ _ _ _ _ _ _ _ _ _ _ _ _ _ _] -> [_ _ _ _ _ w1699 _ _ _ _ _ _ _ _ _ _ _]
          seq-local: [_ w194 _ _ _ _ _ _ _ _ _ _ _ _ _ _ _] -> [_ _ _ _ _ w1698 _ _ _ _ _ _ _ _ _ _ _]
          seq-local: [_ w193 _ _ _ _ _ _ _ _ _ _ _ _ _ _ _] -> [_ _ _ _ _ w1697 _ _ _ _ _ _ _ _ _ _ _]
          seq-local: [_ w192 _ _ _ _ _ _ _ _ _ _ _ _ _ _ _] -> [_ _ _ _ _ w1696 _ _ _ _ _ _ _ _ _ _ _]
          seq-local: [_ w191 _ _ _ _ _ _ _ _ _ _ _ _ _ _ _] -> [_ _ _ _ _ w1695 _ _ _ _ _ _ _ _ _ _ _]
          seq-local: [_ w190 _ _ _ _ _ _ _ _ _ _ _ _ _ _ _] -> [_ _ _ _ _ w1694 _ _ _ _ _ _ _ _ _ _ _]
          seq-local: [_ w189 _ _ _ _ _ _ _ _ _ _ _ _ _ _ _] -> [_ _ _ _ _ w1693 _ _ _ _ _ _ _ _ _ _ _]
          seq-local: [_ w188 _ _ _ _ _ _ _ _ _ _ _ _ _ _ _] -> [_ _ _ _ _ w1692 _ _ _ _ _ _ _ _ _ _ _]
          tunnel: w156 -> [_ _ w225 w386 w1301 w1721 w2031 _ _ _ _ w2476 w2964 _ _ w3225 w3486]
          tunnel: w155 -> [_ _ w224 w384 w1300 w1720 w2030 _ _ _ _ w2475 w2962 _ _ w3224 w3487]
          tunnel: w154 -> [_ _ w223 w382 w1299 w1719 w2029 _ _ _ _ w2474 w2960 _ _ w3223 w3485]
          tunnel: w153 -> [_ _ w222 w380 w1298 w1718 w2028 _ _ _ _ w2473 w2958 _ _ w3222 w3484]
          tunnel: w152 -> [_ _ w221 w378 w1297 w1717 w2027 _ _ _ _ w2472 w2956 _ _ w3221 w3483]
          tunnel: w151 -> [_ _ w220 w376 w1296 w1716 w2026 _ _ _ _ w2471 w2954 _ _ w3220 w3482]
          tunnel: w150 -> [_ _ w219 w374 w1295 w1715 w2025 _ _ _ _ w2470 w2952 _ _ w3219 w3481]
          tunnel: w149 -> [_ _ w218 w372 w1294 w1714 w2024 _ _ _ _ w2469 w2950 _ _ w3218 w3480]
          tunnel: w148 -> [_ _ w217 w370 w1293 w1713 w2023 _ _ _ _ w2468 w2948 _ _ w3217 w3479]
          tunnel: w147 -> [_ _ w216 w368 w1292 w1712 w2022 _ _ _ _ w2467 w2946 _ _ w3216 w3478]
          tunnel: w146 -> [_ _ _ w385 w1291 w1711 _ _ _ _ _ _ w2966 _ _ _ _]
          tunnel: w145 -> [_ _ _ w383 w1290 w1710 _ _ _ _ _ _ w2961 _ _ _ _]
          tunnel: w144 -> [_ _ _ w381 w1289 w1709 _ _ _ _ _ _ w2959 _ _ _ _]
          tunnel: w143 -> [_ _ _ w379 w1288 w1708 _ _ _ _ _ _ w2957 _ _ _ _]
          tunnel: w142 -> [_ _ _ w377 w1287 w1707 _ _ _ _ _ _ w2955 _ _ _ _]
          tunnel: w141 -> [_ _ _ w375 w1286 w1706 _ _ _ _ _ _ w2953 _ _ _ _]
          tunnel: w140 -> [_ _ _ w373 w1285 w1705 _ _ _ _ _ _ w2951 _ _ _ _]
          tunnel: w139 -> [_ _ _ w371 w1284 w1704 _ _ _ _ _ _ w2949 _ _ _ _]
          tunnel: w138 -> [_ _ _ w369 w1283 w1703 _ _ _ _ _ _ w2947 _ _ _ _]
          tunnel: w137 -> [_ _ _ w367 w1282 w1702 _ _ _ _ _ _ w2945 _ _ _ _]
          frame #0 {
            w160 = FALSE
            w165 = 0.5
            # "set up cycle control"
            n140 = local read "jig cycle"() -> (w164:dbl)
            n141 = Divide(x="JIG ON TIME (S)", y=w165) -> (x/y=→"on loops":dbl)
            n142 = Divide(x="JIG OFF TIME (S)", y=w165) -> (x/y=→"off loops":dbl)
            n143 = Increment(x=w164) -> (x+1=w163:dbl)
            n144 = local write "TEMP update"(w160) -> ()
            n145 = local write "AI update"(w160) -> ()
            n146 = local write "jig cycle"(w163) -> ()
          }
          frame #1 {
            w205 = 60.0
            # "convert temperature rise minutes to cycles"
            n147 = local read "SET LAB05-2"() -> (w169:T5)
            n148 = local read "SET LAB05-1"() -> (w171:T5)
            n149 = local read "SET LAB04-2"() -> (w173:T5)
            n150 = local read "SET LAB01-1"() -> (w187:T5)
            n151 = local read "SET LAB01-2"() -> (w185:T5)
            n152 = local read "SET LAB02-2"() -> (w181:T5)
            n153 = local read "SET LAB04-1"() -> (w175:T5)
            n154 = local read "SET LAB03-1"() -> (w179:T5)
            n155 = local read "SET LAB03-2"() -> (w177:T5)
            n156 = local read "SET LAB02-1"() -> (w183:T5)
            n157 = local read "JIG OFF TIME (S)"() -> (w210:dbl)
            n158 = local read "JIG ON TIME (S)"() -> (w211:dbl)
            n159 = Unbundle(w169) -> ("T-RISE mins"=w168:dbl)  [unwired: 4 out]
            n160 = Unbundle(w171) -> ("T-RISE mins"=w170:dbl)  [unwired: 4 out]
            n161 = Unbundle(w187) -> ("T-RISE mins"=w186:dbl)  [unwired: 4 out]
            n162 = Unbundle(w173) -> ("T-RISE mins"=w172:dbl)  [unwired: 4 out]
            n163 = Unbundle(w185) -> ("T-RISE mins"=w184:dbl)  [unwired: 4 out]
            n164 = Unbundle(w183) -> ("T-RISE mins"=w182:dbl)  [unwired: 4 out]
            n165 = Unbundle(w175) -> ("T-RISE mins"=w174:dbl)  [unwired: 4 out]
            n166 = Unbundle(w181) -> ("T-RISE mins"=w180:dbl)  [unwired: 4 out]
            n167 = Unbundle(w177) -> ("T-RISE mins"=w176:dbl)  [unwired: 4 out]
            n168 = Unbundle(w179) -> ("T-RISE mins"=w178:dbl)  [unwired: 4 out]
            n169 = Add(x=w211, y=w210) -> (x+y=w204:dbl)
            n170 = Multiply(x=w205, y=w176) -> (x*y=w200:dbl)
            n171 = Multiply(x=w205, y=w174) -> (x*y=w199:dbl)
            n172 = Multiply(x=w205, y=w172) -> (x*y=w198:dbl)
            n173 = Multiply(x=w205, y=w170) -> (x*y=w197:dbl)
            n174 = Multiply(x=w205, y=w168) -> (x*y=w196:dbl)
            n175 = Multiply(x=w205, y=w184) -> (x*y=w206:dbl)
            n176 = Multiply(x=w205, y=w178) -> (x*y=w201:dbl)
            n177 = Multiply(x=w205, y=w186) -> (x*y=w207:dbl)
            n178 = Multiply(x=w205, y=w182) -> (x*y=w203:dbl)
            n179 = Multiply(x=w205, y=w180) -> (x*y=w202:dbl)
            n180 = Divide(x=w197, y=w204) -> (x/y=w189:dbl)
            n181 = Divide(x=w198, y=w204) -> (x/y=w190:dbl)
            n182 = Divide(x=w199, y=w204) -> (x/y=w191:dbl)
            n183 = Divide(x=w196, y=w204) -> (x/y=w188:dbl)
            n184 = Divide(x=w201, y=w204) -> (x/y=w193:dbl)
            n185 = Divide(x=w207, y=w204) -> (x/y=w209:dbl)
            n186 = Divide(x=w206, y=w204) -> (x/y=w208:dbl)
            n187 = Divide(x=w203, y=w204) -> (x/y=w195:dbl)
            n188 = Divide(x=w202, y=w204) -> (x/y=w194:dbl)
            n189 = Divide(x=w200, y=w204) -> (x/y=w192:dbl)
          }
          frame #2 {
            # "control cycle loops"
            n190 = local read "JIG OFF TIME (S)"() -> (w214:dbl)
            n191 = local read "JIG ON TIME (S)"() -> (w213:dbl)
            n192 = local read "jig cycle"() -> (w227:dbl)
            n193 = local read "on loops"() -> (w229:dbl)
            n194 = local read "off loops"() -> (w228:dbl)
            n195 = Add(x=w214, y=w213) -> (x+y=w212:dbl)
            n196 = Add(x=w229, y=w228) -> (x+y=w215:dbl)
            n197 = Greater Or Equal?(x=w227, y=w215) -> (x >= y?=w226:bool)
            n198 = case shown="True" w226 {
              tunnel: w225 -> [_ w240]
              tunnel: w224 -> [_ w239]
              tunnel: w223 -> [_ w238]
              tunnel: w222 -> [_ w237]
              tunnel: w221 -> [_ w236]
              tunnel: w220 -> [_ w235]
              tunnel: w219 -> [_ w234]
              tunnel: w218 -> [_ w233]
              tunnel: w217 -> [_ w232]
              tunnel: w216 -> [_ w231]
              tunnel: w212 -> [_ w230]
              frame False {
              }
              frame True {
                # "increment cycle value and convert cycles to minutes for temp rise"
                n199 = stacked-sequence {
                  tunnel: w240 -> [w250 _ _ _ _ _ _ _ _ _]
                  tunnel: w239 -> [_ w262 _ _ _ _ _ _ _ _]
                  tunnel: w238 -> [_ _ w274 _ _ _ _ _ _ _]
                  tunnel: w237 -> [_ _ _ w286 _ _ _ _ _ _]
                  tunnel: w236 -> [_ _ _ _ w298 _ _ _ _ _]
                  tunnel: w235 -> [_ _ _ _ _ w310 _ _ _ _]
                  tunnel: w234 -> [_ _ _ _ _ _ w322 _ _ _]
                  tunnel: w233 -> [_ _ _ _ _ _ _ w334 _ _]
                  tunnel: w232 -> [_ _ _ _ _ _ _ _ w346 _]
                  tunnel: w231 -> [_ _ _ _ _ _ _ _ _ w358]
                  tunnel: w230 -> [w247 w259 w271 w283 w295 w307 w319 w331 w343 w355]
                  frame #0 {
                    # "LAB01-1"
                    n200 = local read "DISP LAB01-1"() -> (w245:T4)
                    n201 = Unbundle(w245) -> ("CYCLE"=w246:dbl)  [unwired: 2 out]
                    n202 = case shown="True" w250 {
                      tunnel: w246 -> [w251 w253]
                      tunnel: [w251 w252] -> w244
                      frame False {
                      }
                      frame True {
                        n203 = Increment(x=w253) -> (x+1=w252:dbl)
                      }
                    }
                    n204 = Multiply(x=w244, y=w247) -> (x*y=w248:dbl)
                    n205 = Divide(x=w248, y=60.0) -> (x/y=w243:dbl)
                    n206 = Bundle(cluster=w245, "CYCLE"=w244, "MINS"=w243) -> (w242:T4)  [unwired: 1 in]
                    n207 = local write "DISP LAB01-1"(w242) -> ()
                  }
                  frame #1 {
                    # "update cycle value"
                    # "LAB01-2"
                    n208 = local read "DISP LAB01-2"() -> (w257:T4)
                    n209 = Unbundle(w257) -> ("CYCLE"=w258:dbl)  [unwired: 2 out]
                    n210 = case shown="True" w262 {
                      tunnel: w258 -> [w263 w265]
                      tunnel: [w263 w264] -> w255
                      frame False {
                      }
                      frame True {
                        n211 = Increment(x=w265) -> (x+1=w264:dbl)
                      }
                    }
                    n212 = Multiply(x=w255, y=w259) -> (x*y=w260:dbl)
                    n213 = Divide(x=w260, y=60.0) -> (x/y=w254:dbl)
                    n214 = Bundle(cluster=w257, "CYCLE"=w255, "MINS"=w254) -> (w256:T4)  [unwired: 1 in]
                    n215 = local write "DISP LAB01-2"(w256) -> ()
                  }
                  frame #2 {
                    # "update cycle value"
                    # "LAB02-1"
                    n216 = local read "DISP LAB02-1"() -> (w269:T4)
                    n217 = Unbundle(w269) -> ("CYCLE"=w270:dbl)  [unwired: 2 out]
                    n218 = case shown="True" w274 {
                      tunnel: [w275 w277] -> w267
                      tunnel: w270 -> [w275 w276]
                      frame False {
                      }
                      frame True {
                        n219 = Increment(x=w276) -> (x+1=w277:dbl)
                      }
                    }
                    n220 = Multiply(x=w267, y=w271) -> (x*y=w272:dbl)
                    n221 = Divide(x=w272, y=60.0) -> (x/y=w266:dbl)
                    n222 = Bundle(cluster=w269, "CYCLE"=w267, "MINS"=w266) -> (w268:T4)  [unwired: 1 in]
                    n223 = local write "DISP LAB02-1"(w268) -> ()
                  }
                  frame #3 {
                    # "update cycle value"
                    # "LAB02-2"
                    n224 = local read "DISP LAB02-2"() -> (w281:T4)
                    n225 = Unbundle(w281) -> ("CYCLE"=w282:dbl)  [unwired: 2 out]
                    n226 = case shown="True" w286 {
                      tunnel: [w287 w289] -> w280
                      tunnel: w282 -> [w287 w288]
                      frame False {
                      }
                      frame True {
                        n227 = Increment(x=w288) -> (x+1=w289:dbl)
                      }
                    }
                    n228 = Multiply(x=w280, y=w283) -> (x*y=w284:dbl)
                    n229 = Divide(x=w284, y=60.0) -> (x/y=w279:dbl)
                    n230 = Bundle(cluster=w281, "CYCLE"=w280, "MINS"=w279) -> (w278:T4)  [unwired: 1 in]
                    n231 = local write "DISP LAB02-2"(w278) -> ()
                  }
                  frame #4 {
                    # "update cycle value"
                    # "LAB03-1"
                    n232 = local read "DISP LAB03-1"() -> (w293:T4)
                    n233 = Unbundle(w293) -> ("CYCLE"=w294:dbl)  [unwired: 2 out]
                    n234 = case shown="True" w298 {
                      tunnel: [w299 w301] -> w290
                      tunnel: w294 -> [w299 w300]
                      frame False {
                      }
                      frame True {
                        n235 = Increment(x=w300) -> (x+1=w301:dbl)
                      }
                    }
                    n236 = Multiply(x=w290, y=w295) -> (x*y=w296:dbl)
                    n237 = Divide(x=w296, y=60.0) -> (x/y=w291:dbl)
                    n238 = Bundle(cluster=w293, "CYCLE"=w290, "MINS"=w291) -> (w292:T4)  [unwired: 1 in]
                    n239 = local write "DISP LAB03-1"(w292) -> ()
                  }
                  frame #5 {
                    # "update cycle value"
                    # "LAB03-2"
                    n240 = local read "DISP LAB03-2"() -> (w305:T4)
                    n241 = Unbundle(w305) -> ("CYCLE"=w306:dbl)  [unwired: 2 out]
                    n242 = case shown="False" w310 {
                      tunnel: [w311 w313] -> w304
                      tunnel: w306 -> [w311 w312]
                      frame False {
                      }
                      frame True {
                        n243 = Increment(x=w312) -> (x+1=w313:dbl)
                      }
                    }
                    n244 = Multiply(x=w304, y=w307) -> (x*y=w308:dbl)
                    n245 = Divide(x=w308, y=60.0) -> (x/y=w303:dbl)
                    n246 = Bundle(cluster=w305, "CYCLE"=w304, "MINS"=w303) -> (w302:T4)  [unwired: 1 in]
                    n247 = local write "DISP LAB03-2"(w302) -> ()
                  }
                  frame #6 {
                    # "update cycle value"
                    # "LAB04-1"
                    n248 = local read "DISP LAB04-1"() -> (w317:T4)
                    n249 = Unbundle(w317) -> ("CYCLE"=w318:dbl)  [unwired: 2 out]
                    n250 = case shown="True" w322 {
                      tunnel: [w323 w325] -> w315
                      tunnel: w318 -> [w323 w324]
                      frame False {
                      }
                      frame True {
                        n251 = Increment(x=w324) -> (x+1=w325:dbl)
                      }
                    }
                    n252 = Multiply(x=w315, y=w319) -> (x*y=w320:dbl)
                    n253 = Divide(x=w320, y=60.0) -> (x/y=w314:dbl)
                    n254 = Bundle(cluster=w317, "CYCLE"=w315, "MINS"=w314) -> (w316:T4)  [unwired: 1 in]
                    n255 = local write "DISP LAB04-1"(w316) -> ()
                  }
                  frame #7 {
                    # "update cycle value"
                    # "LAB04-2"
                    n256 = local read "DISP LAB04-2"() -> (w329:T4)
                    n257 = Unbundle(w329) -> ("CYCLE"=w330:dbl)  [unwired: 2 out]
                    n258 = case shown="True" w334 {
                      tunnel: [w335 w337] -> w327
                      tunnel: w330 -> [w335 w336]
                      frame False {
                      }
                      frame True {
                        n259 = Increment(x=w336) -> (x+1=w337:dbl)
                      }
                    }
                    n260 = Multiply(x=w327, y=w331) -> (x*y=w333:dbl)
                    n261 = Divide(x=w333, y=60.0) -> (x/y=w326:dbl)
                    n262 = Bundle(cluster=w329, "CYCLE"=w327, "MINS"=w326) -> (w328:T4)  [unwired: 1 in]
                    n263 = local write "DISP LAB04-2"(w328) -> ()
                  }
                  frame #8 {
                    # "update cycle value"
                    # "LAB05-1"
                    n264 = local read "DISP LAB05-1"() -> (w341:T4)
                    n265 = Unbundle(w341) -> ("CYCLE"=w342:dbl)  [unwired: 2 out]
                    n266 = case shown="True" w346 {
                      tunnel: [w347 w349] -> w339
                      tunnel: w342 -> [w347 w348]
                      frame False {
                      }
                      frame True {
                        n267 = Increment(x=w348) -> (x+1=w349:dbl)
                      }
                    }
                    n268 = Multiply(x=w339, y=w343) -> (x*y=w344:dbl)
                    n269 = Divide(x=w344, y=60.0) -> (x/y=w338:dbl)
                    n270 = Bundle(cluster=w341, "CYCLE"=w339, "MINS"=w338) -> (w340:T4)  [unwired: 1 in]
                    n271 = local write "DISP LAB05-1"(w340) -> ()
                  }
                  frame #9 {
                    # "update cycle value"
                    # "LAB05-2"
                    n272 = local read "DISP LAB05-2"() -> (w354:T4)
                    n273 = Unbundle(w354) -> ("CYCLE"=w353:dbl)  [unwired: 2 out]
                    n274 = case shown="True" w358 {
                      tunnel: [w359 w361] -> w352
                      tunnel: w353 -> [w359 w360]
                      frame False {
                      }
                      frame True {
                        n275 = Increment(x=w360) -> (x+1=w361:dbl)
                      }
                    }
                    n276 = Multiply(x=w352, y=w355) -> (x*y=w356:dbl)
                    n277 = Divide(x=w356, y=60.0) -> (x/y=w351:dbl)
                    n278 = Bundle(cluster=w354, "CYCLE"=w352, "MINS"=w351) -> (w350:T4)  [unwired: 1 in]
                    n279 = local write "DISP LAB05-2"(w350) -> ()
                  }
                }
                n280 = local write "jig cycle"(0) -> ()
              }
            }
          }
          frame #3 {
            # "START & STOP test RUN switch change, start test if true and stop test if false"
            n281 = Get Date/Time In Seconds() -> (seconds since 1Jan1904=w365:timestamp)
            n282 = Format Date/Time String(time format string (%c)="%b%d", seconds (now)=w365) -> (date/time string=w389:string)  [unwired: 1 in]
            n283 = Format Date/Time String(time format string (%c)="%H%M", seconds (now)=w365) -> (date/time string=w387:string)  [unwired: 1 in]
            n284 = Format Date/Time String(time format string (%c)="%Y", seconds (now)=w365) -> (date/time string=w364:string)  [unwired: 1 in]
            n285 = event shown="[1] \"RUN LAB01-1\": Value Change" {
              selector: _ -> [_ _ _ _ _ _ _ _ _ _ _]
              dyn-events: _ -> [_ _ _ _ _ _ _ _ _ _ _]
              timeout: 10 -> [_ _ _ _ _ _ _ _ _ _ _]
              tunnel: "c:\\crabtree\\Test Data\\" -> [_ w398 w487 w576 w665 w754 w843 w932 w1021 w1110 w1199]
              tunnel: w389 -> [_ w397 w486 w575 w664 w753 w842 w931 w1020 w1109 w1198]
              tunnel: w387 -> [_ w395 w485 w574 w663 w752 w841 w930 w1019 w1108 w1197]
              tunnel: w385 -> [_ w396 _ _ _ _ _ _ _ _ _]
              tunnel: w386 -> [_ _ _ _ _ _ _ _ _ _ _]
              tunnel: w384 -> [_ _ _ _ _ _ _ _ _ _ _]
              tunnel: w383 -> [_ _ w484 _ _ _ _ _ _ _ _]
              tunnel: w382 -> [_ _ _ _ _ _ _ _ _ _ _]
              tunnel: w381 -> [_ _ _ w573 _ _ _ _ _ _ _]
              tunnel: w380 -> [_ _ _ _ _ _ _ _ _ _ _]
              tunnel: w379 -> [_ _ _ _ w662 _ _ _ _ _ _]
              tunnel: w378 -> [_ _ _ _ _ _ _ _ _ _ _]
              tunnel: w377 -> [_ _ _ _ _ w751 _ _ _ _ _]
              tunnel: w376 -> [_ _ _ _ _ _ _ _ _ _ _]
              tunnel: w375 -> [_ _ _ _ _ _ w840 _ _ _ _]
              tunnel: w374 -> [_ _ _ _ _ _ _ _ _ _ _]
              tunnel: w373 -> [_ _ _ _ _ _ _ w929 _ _ _]
              tunnel: w372 -> [_ _ _ _ _ _ _ _ _ _ _]
              tunnel: w371 -> [_ _ _ _ _ _ _ _ w1018 _ _]
              tunnel: w370 -> [_ _ _ _ _ _ _ _ _ _ _]
              tunnel: w369 -> [_ _ _ _ _ _ _ _ _ w1107 _]
              tunnel: w368 -> [_ _ _ _ _ _ _ _ _ _ _]
              tunnel: w367 -> [_ _ _ _ _ _ _ _ _ _ w1196]
              tunnel: w364 -> [_ w393 w482 w571 w660 w749 w838 w927 w1016 w1105 w1194]
              tunnel: [_ w392 w481 w570 w659 w748 w837 w926 w1015 w1104 w1193] -> w362
              event Timeout {
                n286 = event-data() -> ()  [unwired: 1 in, 3 out]
              }
              event "RUN LAB01-1": Value Change {
                n287 = event-data() -> ("NewVal"=w394:bool)  [unwired: 1 in, 5 out]
                n288 = case shown="True" w394 {
                  tunnel: w398 -> [_ w428]
                  tunnel: w397 -> [_ w427]
                  tunnel: w396 -> [w400 w426]
                  tunnel: w395 -> [_ w425]
                  tunnel: w393 -> [_ w424]
                  tunnel: [w399 w423] -> w392
                  frame False {
                    # "stop test"
                    n289 = stacked-sequence {
                      tunnel: w400 -> [w409 _]
                      tunnel: [w401 _] -> w399
                      frame #0 {
                        n290 = local read "DISP LAB01-1"() -> (w408:T4)
                        n291 = Unbundle(w408) -> ("CYCLE"=w406:dbl, "MINS"=w407:dbl)  [unwired: 1 out]
                        n292 = case shown="\"CYCLE TEST\"" w409 {
                          tunnel: w407 -> [_ _ w416]
                          tunnel: w406 -> [w414 w415 _]
                          tunnel: [w414 w415 w416] -> w405
                          frame "CHART TEST", Default {
                          }
                          frame "CYCLE TEST" {
                          }
                          frame "T-RISE TEST" {
                          }
                        }
                        n293 = local read "TDMS LAB01-1"() -> (w413:refnum<k34>)
                        n294 = Build Array("STOPPED") -> (w410:string[])
                        n295 = Build Array(w405) -> (w404:dbl[])
                        n296 = TDMS Write(0:w413, 5:"TEST RESULT", 7:w410, 9:w404) -> (4:w402:refnum<k34>, 15:w403:errorcluster)  [unwired: 2 in, 2 out]
                        n297 = TDMS Close(8:w403, 11:w402) -> (0:w401:errorcluster)  [unwired: 1 out]
                      }
                      frame #1 {
                        n298 = local read "DISP LAB01-1"() -> (w422:T4)
                        n299 = Bundle(cluster=w422, "STATUS"="STOP") -> (w420:T4)  [unwired: 2 in]
                        n300 = call "Save data file to network drive v1.vi"("panel id"="LAB01-1") -> ("network file save error"=w417:errorcluster)  [unwired: 9 in, 1 out]
                        n301 = local write "RESULT LAB01-1"(FALSE) -> ()
                        n302 = local write "DISP LAB01-1"(w420) -> ()
                        n303 = local write "data file error"(w417) -> ()
                      }
                    }
                  }
                  frame True {
                    # "start new test and create test file"
                    n304 = stacked-sequence {
                      seq-local: [w429 _ _ _ _] -> [_ w454 _ _ _]
                      tunnel: w428 -> [w434 _ _ _ _]
                      tunnel: w427 -> [w430 _ _ _ _]
                      tunnel: w426 -> [w444 _ _ _ _]
                      tunnel: w425 -> [w437 _ _ _ _]
                      tunnel: w424 -> [w432 _ _ _ _]
                      tunnel: [_ w448 _ _ _] -> w423
                      frame #0 {
                        w431 = "\\"
                        n305 = local read "SET LAB01-1"() -> (w439:T5)
                        n306 = case shown="\"CHART TEST\", Default" w444 {
                          tunnel: ["CHART TEST-" "CYCLE TEST-" "T-RISE TEST-"] -> w440
                          frame "CHART TEST", Default {
                          }
                          frame "CYCLE TEST" {
                          }
                          frame "T-RISE TEST" {
                          }
                        }
                        n307 = Unbundle(w439) -> ("DESCRIPTION"=w438:string)  [unwired: 4 out]
                        n308 = Concatenate Strings(w434, "LAB01-1\\", w432, w431, w430, w431) -> (w441:string)
                        n309 = String To Path(string=w441) -> (path=w443:path)
                        n310 = Concatenate Strings(w441, w440, w438, "-", w437, ".tdms") -> (w429:string)
                        n311 = Create Folder(path (use dialog)=w443) -> (error out=w442:errorcluster)  [unwired: 2 in, 2 out]
                        n312 = call <vilib>:"Clear Errors.vi"("error in (no error)"=w442) -> ()  [unwired: 6 in, 1 out]
                        n313 = global write "Global 1.vi" "LAB01-1 FILE"(w429) -> ()
                      }
                      frame #1 {
                        n314 = String To Path(string=w454) -> (path=w449:path)
                        n315 = TDMS Open(5:FALSE, 6:FALSE, 10:T15."create or replace" ("operation (0:open)"), 11:w449) -> (0:w448:errorcluster, 3:→"TDMS LAB01-1":refnum<k34>)  [unwired: 3 in]
                      }
                      frame #2 {
                        n316 = local read "SET LAB01-1"() -> (w460:T5)
                        n317 = local read "TDMS LAB01-1"() -> (w471:refnum<k34>)
                        n318 = Build Array("Testers Name", "Description", "Set Test Cycles", "T-Rise minutes", "T-Rise Deg C") -> (w461:string[])
                        n319 = Unbundle(w460) -> ("NAME"=w459:string, "DESCRIPTION"=w458:string, "CYCLES"=w457:dbl, "T-RISE mins"=w456:dbl, "T-RISE deg C"=w455:dbl)
                        n320 = Number To Decimal String(number=w457) -> (decimal integer string=w470:string)  [unwired: 1 in]
                        n321 = Number To Decimal String(number=w456) -> (decimal integer string=w469:string)  [unwired: 1 in]
                        n322 = Number To Decimal String(number=w455) -> (decimal integer string=w468:string)  [unwired: 1 in]
                        n323 = Build Array(w459, w458, w470, w469, w468) -> (w467:string[])
                        n324 = TDMS Set Properties(5:w467, 7:w461, 11:w471) -> ()  [unwired: 3 in, 4 out]
                      }
                      frame #3 {
                        w472 = 0.0
                        n325 = local read "DISP LAB01-1"() -> (w475:T4)
                        n326 = Bundle(cluster=w475, "CYCLE"=w472, "MINS"=w472, "STATUS"="RUN") -> (w474:T4)
                        n327 = local write "DISP LAB01-1"(w474) -> ()
                      }
                      frame #4 {
                        n328 = local read "SIG LAB01-1"() -> (w478:T2)
                        n329 = local read "TEMP START LAB01-1"() -> (w480:cluster{"TL":dbl, "TN":dbl})
                        n330 = Unbundle(w478) -> ("Tmp Live"=w477:dbl, "Tmp Neut"=w476:dbl)  [unwired: 3 out]
                        n331 = Bundle(cluster=w480, "TL"=w477, "TN"=w476) -> (w479:cluster{"TL":dbl, "TN":dbl})
                        n332 = local write "TEMP START LAB01-1"(w479) -> ()
                      }
                    }
                  }
                }
              }
              event "RUN LAB01-2": Value Change {
                n333 = event-data() -> ("NewVal"=w483:bool)  [unwired: 1 in, 5 out]
                n334 = case shown="False" w483 {
                  tunnel: w487 -> [_ w517]
                  tunnel: w486 -> [_ w516]
                  tunnel: w484 -> [w489 w515]
                  tunnel: w485 -> [_ w514]
                  tunnel: w482 -> [_ w513]
                  tunnel: [w488 w512] -> w481
                  frame False {
                    # "stop test"
                    n335 = stacked-sequence {
                      tunnel: w489 -> [w498 _]
                      tunnel: [w490 _] -> w488
                      frame #0 {
                        n336 = local read "DISP LAB01-2"() -> (w497:T4)
                        n337 = Unbundle(w497) -> ("CYCLE"=w495:dbl, "MINS"=w496:dbl)  [unwired: 1 out]
                        n338 = case shown="\"CHART TEST\", Default" w498 {
                          tunnel: w496 -> [_ _ w505]
                          tunnel: w495 -> [w503 w504 _]
                          tunnel: [w503 w504 w505] -> w494
                          frame "CHART TEST", Default {
                          }
                          frame "CYCLE TEST" {
                          }
                          frame "T-RISE TEST" {
                          }
                        }
                        n339 = local read "TDMS LAB01-2"() -> (w502:refnum<k34>)
                        n340 = Build Array("STOPPED") -> (w499:string[])
                        n341 = Build Array(w494) -> (w493:dbl[])
                        n342 = TDMS Write(0:w502, 5:"TEST RESULT", 7:w499, 9:w493) -> (4:w491:refnum<k34>, 15:w492:errorcluster)  [unwired: 2 in, 2 out]
                        n343 = TDMS Close(8:w492, 11:w491) -> (0:w490:errorcluster)  [unwired: 1 out]
                      }
                      frame #1 {
                        n344 = local read "DISP LAB01-2"() -> (w511:T4)
                        n345 = Bundle(cluster=w511, "STATUS"="STOP") -> (w509:T4)  [unwired: 2 in]
                        n346 = call "Save data file to network drive v1.vi"("panel id"="LAB01-2") -> ("network file save error"=w506:errorcluster)  [unwired: 9 in, 1 out]
                        n347 = local write "RESULT LAB01-2"(FALSE) -> ()
                        n348 = local write "DISP LAB01-2"(w509) -> ()
                        n349 = local write "data file error"(w506) -> ()
                      }
                    }
                  }
                  frame True {
                    # "start new test and create test file"
                    n350 = stacked-sequence {
                      seq-local: [w518 _ _ _ _] -> [_ w543 _ _ _]
                      tunnel: w517 -> [w523 _ _ _ _]
                      tunnel: w516 -> [w520 _ _ _ _]
                      tunnel: w515 -> [w533 _ _ _ _]
                      tunnel: w514 -> [w526 _ _ _ _]
                      tunnel: w513 -> [w521 _ _ _ _]
                      tunnel: [_ w537 _ _ _] -> w512
                      frame #0 {
                        w519 = "\\"
                        n351 = local read "SET LAB01-2"() -> (w528:T5)
                        n352 = case shown="\"CHART TEST\", Default" w533 {
                          tunnel: ["CHART TEST-" "CYCLE TEST-" "T-RISE TEST-"] -> w529
                          frame "CHART TEST", Default {
                          }
                          frame "CYCLE TEST" {
                          }
                          frame "T-RISE TEST" {
                          }
                        }
                        n353 = Unbundle(w528) -> ("DESCRIPTION"=w527:string)  [unwired: 4 out]
                        n354 = Concatenate Strings(w523, "LAB01-2\\", w521, w519, w520, w519) -> (w530:string)
                        n355 = String To Path(string=w530) -> (path=w532:path)
                        n356 = Concatenate Strings(w530, w529, w527, "-", w526, ".tdms") -> (w518:string)
                        n357 = Create Folder(path (use dialog)=w532) -> (error out=w531:errorcluster)  [unwired: 2 in, 2 out]
                        n358 = global write "Global 1.vi" "LAB01-2 FILE"(w518) -> ()
                        n359 = call <vilib>:"Clear Errors.vi"("error in (no error)"=w531) -> ()  [unwired: 6 in, 1 out]
                      }
                      frame #1 {
                        n360 = String To Path(string=w543) -> (path=w538:path)
                        n361 = TDMS Open(5:FALSE, 6:FALSE, 10:T15."create or replace" ("operation (0:open)"), 11:w538) -> (0:w537:errorcluster, 3:→"TDMS LAB01-2":refnum<k34>)  [unwired: 3 in]
                      }
                      frame #2 {
                        n362 = local read "SET LAB01-2"() -> (w549:T5)
                        n363 = local read "TDMS LAB01-2"() -> (w560:refnum<k34>)
                        n364 = Build Array("Testers Name", "Description", "Set Test Cycles", "T-Rise minutes", "T-Rise Deg C") -> (w550:string[])
                        n365 = Unbundle(w549) -> ("NAME"=w548:string, "DESCRIPTION"=w547:string, "CYCLES"=w546:dbl, "T-RISE mins"=w545:dbl, "T-RISE deg C"=w544:dbl)
                        n366 = Number To Decimal String(number=w546) -> (decimal integer string=w559:string)  [unwired: 1 in]
                        n367 = Number To Decimal String(number=w545) -> (decimal integer string=w558:string)  [unwired: 1 in]
                        n368 = Number To Decimal String(number=w544) -> (decimal integer string=w557:string)  [unwired: 1 in]
                        n369 = Build Array(w548, w547, w559, w558, w557) -> (w556:string[])
                        n370 = TDMS Set Properties(5:w556, 7:w550, 11:w560) -> ()  [unwired: 3 in, 4 out]
                      }
                      frame #3 {
                        w562 = 0.0
                        n371 = local read "DISP LAB01-2"() -> (w564:T4)
                        n372 = Bundle(cluster=w564, "CYCLE"=w562, "MINS"=w562, "STATUS"="RUN") -> (w563:T4)
                        n373 = local write "DISP LAB01-2"(w563) -> ()
                      }
                      frame #4 {
                        n374 = local read "SIG LAB01-2"() -> (w567:T2)
                        n375 = local read "TEMP START LAB01-2"() -> (w569:cluster{"TL":dbl, "TN":dbl})
                        n376 = Unbundle(w567) -> ("Tmp Live"=w566:dbl, "Tmp Neut"=w565:dbl)  [unwired: 3 out]
                        n377 = Bundle(cluster=w569, "TL"=w566, "TN"=w565) -> (w568:cluster{"TL":dbl, "TN":dbl})
                        n378 = local write "TEMP START LAB01-2"(w568) -> ()
                      }
                    }
                  }
                }
              }
              event "RUN LAB02-1": Value Change {
                n379 = event-data() -> ("NewVal"=w572:bool)  [unwired: 1 in, 5 out]
                n380 = case shown="False" w572 {
                  tunnel: w576 -> [_ w606]
                  tunnel: w575 -> [_ w605]
                  tunnel: w573 -> [w578 w604]
                  tunnel: w574 -> [_ w603]
                  tunnel: w571 -> [_ w602]
                  tunnel: [w577 w601] -> w570
                  frame False {
                    # "stop test"
                    n381 = stacked-sequence {
                      tunnel: w578 -> [w587 _]
                      tunnel: [w579 _] -> w577
                      frame #0 {
                        n382 = local read "DISP LAB02-1"() -> (w586:T4)
                        n383 = Unbundle(w586) -> ("CYCLE"=w584:dbl, "MINS"=w585:dbl)  [unwired: 1 out]
                        n384 = case shown="\"CYCLE TEST\"" w587 {
                          tunnel: w585 -> [_ _ w594]
                          tunnel: w584 -> [w592 w593 _]
                          tunnel: [w592 w593 w594] -> w583
                          frame "CHART TEST", Default {
                          }
                          frame "CYCLE TEST" {
                          }
                          frame "T-RISE TEST" {
                          }
                        }
                        n385 = local read "TDMS LAB02-1"() -> (w591:refnum<k34>)
                        n386 = Build Array("STOPPED") -> (w588:string[])
                        n387 = Build Array(w583) -> (w582:dbl[])
                        n388 = TDMS Write(0:w591, 5:"TEST RESULT", 7:w588, 9:w582) -> (4:w580:refnum<k34>, 15:w581:errorcluster)  [unwired: 2 in, 2 out]
                        n389 = TDMS Close(8:w581, 11:w580) -> (0:w579:errorcluster)  [unwired: 1 out]
                      }
                      frame #1 {
                        n390 = local read "DISP LAB02-1"() -> (w600:T4)
                        n391 = Bundle(cluster=w600, "STATUS"="STOP") -> (w598:T4)  [unwired: 2 in]
                        n392 = local write "RESULT LAB02-1"(FALSE) -> ()
                        n393 = local write "DISP LAB02-1"(w598) -> ()
                        n394 = call "Save data file to network drive v1.vi"("panel id"="LAB02-1") -> ("network file save error"=w595:errorcluster)  [unwired: 9 in, 1 out]
                        n395 = local write "data file error"(w595) -> ()
                      }
                    }
                  }
                  frame True {
                    # "start new test and create test file"
                    n396 = stacked-sequence {
                      seq-local: [w607 _ _ _ _] -> [_ w632 _ _ _]
                      tunnel: w606 -> [w612 _ _ _ _]
                      tunnel: w605 -> [w609 _ _ _ _]
                      tunnel: w604 -> [w622 _ _ _ _]
                      tunnel: w603 -> [w615 _ _ _ _]
                      tunnel: w602 -> [w610 _ _ _ _]
                      tunnel: [_ w626 _ _ _] -> w601
                      frame #0 {
                        w608 = "\\"
                        n397 = local read "SET LAB02-1"() -> (w617:T5)
                        n398 = case shown="\"CHART TEST\", Default" w622 {
                          tunnel: ["CHART TEST-" "CYCLE TEST-" "T-RISE TEST-"] -> w618
                          frame "CHART TEST", Default {
                          }
                          frame "CYCLE TEST" {
                          }
                          frame "T-RISE TEST" {
                          }
                        }
                        n399 = Unbundle(w617) -> ("DESCRIPTION"=w616:string)  [unwired: 4 out]
                        n400 = Concatenate Strings(w612, "LAB02-1\\", w610, w608, w609, w608) -> (w619:string)
                        n401 = String To Path(string=w619) -> (path=w621:path)
                        n402 = Concatenate Strings(w619, w618, w616, "-", w615, ".tdms") -> (w607:string)
                        n403 = Create Folder(path (use dialog)=w621) -> (error out=w620:errorcluster)  [unwired: 2 in, 2 out]
                        n404 = global write "Global 1.vi" "LAB02-1 FILE"(w607) -> ()
                        n405 = call <vilib>:"Clear Errors.vi"("error in (no error)"=w620) -> ()  [unwired: 6 in, 1 out]
                      }
                      frame #1 {
                        n406 = String To Path(string=w632) -> (path=w627:path)
                        n407 = TDMS Open(5:FALSE, 6:FALSE, 10:T15."create or replace" ("operation (0:open)"), 11:w627) -> (0:w626:errorcluster, 3:→"TDMS LAB02-1":refnum<k34>)  [unwired: 3 in]
                      }
                      frame #2 {
                        n408 = local read "SET LAB02-1"() -> (w638:T5)
                        n409 = local read "TDMS LAB02-1"() -> (w649:refnum<k34>)
                        n410 = Build Array("Testers Name", "Description", "Set Test Cycles", "T-Rise minutes", "T-Rise Deg C") -> (w639:string[])
                        n411 = Unbundle(w638) -> ("NAME"=w637:string, "DESCRIPTION"=w636:string, "CYCLES"=w635:dbl, "T-RISE mins"=w634:dbl, "T-RISE deg C"=w633:dbl)
                        n412 = Number To Decimal String(number=w635) -> (decimal integer string=w648:string)  [unwired: 1 in]
                        n413 = Number To Decimal String(number=w634) -> (decimal integer string=w647:string)  [unwired: 1 in]
                        n414 = Number To Decimal String(number=w633) -> (decimal integer string=w646:string)  [unwired: 1 in]
                        n415 = Build Array(w637, w636, w648, w647, w646) -> (w645:string[])
                        n416 = TDMS Set Properties(5:w645, 7:w639, 11:w649) -> ()  [unwired: 3 in, 4 out]
                      }
                      frame #3 {
                        w651 = 0.0
                        n417 = local read "DISP LAB02-1"() -> (w653:T4)
                        n418 = Bundle(cluster=w653, "CYCLE"=w651, "MINS"=w651, "STATUS"="RUN") -> (w652:T4)
                        n419 = local write "DISP LAB02-1"(w652) -> ()
                      }
                      frame #4 {
                        n420 = local read "SIG LAB02-1"() -> (w656:T2)
                        n421 = local read "TEMP START LAB02-1"() -> (w658:cluster{"TL":dbl, "TN":dbl})
                        n422 = Unbundle(w656) -> ("Tmp Live"=w655:dbl, "Tmp Neut"=w654:dbl)  [unwired: 3 out]
                        n423 = Bundle(cluster=w658, "TL"=w655, "TN"=w654) -> (w657:cluster{"TL":dbl, "TN":dbl})
                        n424 = local write "TEMP START LAB02-1"(w657) -> ()
                      }
                    }
                  }
                }
              }
              event "RUN LAB02-2": Value Change {
                n425 = event-data() -> ("NewVal"=w661:bool)  [unwired: 1 in, 5 out]
                n426 = case shown="False" w661 {
                  tunnel: w665 -> [_ w695]
                  tunnel: w664 -> [_ w694]
                  tunnel: w662 -> [w667 w693]
                  tunnel: w663 -> [_ w692]
                  tunnel: w660 -> [_ w691]
                  tunnel: [w666 w690] -> w659
                  frame False {
                    # "stop test"
                    n427 = stacked-sequence {
                      tunnel: w667 -> [w676 _]
                      tunnel: [w668 _] -> w666
                      frame #0 {
                        n428 = local read "DISP LAB02-2"() -> (w675:T4)
                        n429 = Unbundle(w675) -> ("CYCLE"=w673:dbl, "MINS"=w674:dbl)  [unwired: 1 out]
                        n430 = case shown="\"CYCLE TEST\"" w676 {
                          tunnel: w674 -> [_ _ w683]
                          tunnel: w673 -> [w681 w682 _]
                          tunnel: [w681 w682 w683] -> w672
                          frame "CHART TEST", Default {
                          }
                          frame "CYCLE TEST" {
                          }
                          frame "T-RISE TEST" {
                          }
                        }
                        n431 = local read "TDMS LAB02-2"() -> (w680:refnum<k34>)
                        n432 = Build Array("STOPPED") -> (w677:string[])
                        n433 = Build Array(w672) -> (w671:dbl[])
                        n434 = TDMS Write(0:w680, 5:"TEST RESULT", 7:w677, 9:w671) -> (4:w669:refnum<k34>, 15:w670:errorcluster)  [unwired: 2 in, 2 out]
                        n435 = TDMS Close(8:w670, 11:w669) -> (0:w668:errorcluster)  [unwired: 1 out]
                      }
                      frame #1 {
                        n436 = local read "DISP LAB02-2"() -> (w689:T4)
                        n437 = Bundle(cluster=w689, "STATUS"="STOP") -> (w687:T4)  [unwired: 2 in]
                        n438 = call "Save data file to network drive v1.vi"("panel id"="LAB02-2") -> ("network file save error"=w684:errorcluster)  [unwired: 9 in, 1 out]
                        n439 = local write "RESULT LAB02-2"(FALSE) -> ()
                        n440 = local write "DISP LAB02-2"(w687) -> ()
                        n441 = local write "data file error"(w684) -> ()
                      }
                    }
                  }
                  frame True {
                    # "start new test and create test file"
                    n442 = stacked-sequence {
                      seq-local: [w696 _ _ _ _] -> [_ w721 _ _ _]
                      tunnel: w695 -> [w701 _ _ _ _]
                      tunnel: w694 -> [w698 _ _ _ _]
                      tunnel: w693 -> [w711 _ _ _ _]
                      tunnel: w692 -> [w704 _ _ _ _]
                      tunnel: w691 -> [w699 _ _ _ _]
                      tunnel: [_ w715 _ _ _] -> w690
                      frame #0 {
                        w697 = "\\"
                        n443 = local read "SET LAB02-2"() -> (w706:T5)
                        n444 = case shown="\"CHART TEST\", Default" w711 {
                          tunnel: ["CHART TEST-" "CYCLE TEST-" "T-RISE TEST-"] -> w707
                          frame "CHART TEST", Default {
                          }
                          frame "CYCLE TEST" {
                          }
                          frame "T-RISE TEST" {
                          }
                        }
                        n445 = Unbundle(w706) -> ("DESCRIPTION"=w705:string)  [unwired: 4 out]
                        n446 = Concatenate Strings(w701, "LAB02-2\\", w699, w697, w698, w697) -> (w708:string)
                        n447 = String To Path(string=w708) -> (path=w710:path)
                        n448 = Concatenate Strings(w708, w707, w705, "-", w704, ".tdms") -> (w696:string)
                        n449 = Create Folder(path (use dialog)=w710) -> (error out=w709:errorcluster)  [unwired: 2 in, 2 out]
                        n450 = global write "Global 1.vi" "LAB02-2 FILE"(w696) -> ()
                        n451 = call <vilib>:"Clear Errors.vi"("error in (no error)"=w709) -> ()  [unwired: 6 in, 1 out]
                      }
                      frame #1 {
                        n452 = String To Path(string=w721) -> (path=w716:path)
                        n453 = TDMS Open(5:FALSE, 6:FALSE, 10:T15."create or replace" ("operation (0:open)"), 11:w716) -> (0:w715:errorcluster, 3:→"TDMS LAB02-2":refnum<k34>)  [unwired: 3 in]
                      }
                      frame #2 {
                        n454 = local read "SET LAB02-2"() -> (w727:T5)
                        n455 = local read "TDMS LAB02-2"() -> (w738:refnum<k34>)
                        n456 = Build Array("Testers Name", "Description", "Set Test Cycles", "T-Rise minutes", "T-Rise Deg C") -> (w728:string[])
                        n457 = Unbundle(w727) -> ("NAME"=w726:string, "DESCRIPTION"=w725:string, "CYCLES"=w724:dbl, "T-RISE mins"=w723:dbl, "T-RISE deg C"=w722:dbl)
                        n458 = Number To Decimal String(number=w724) -> (decimal integer string=w737:string)  [unwired: 1 in]
                        n459 = Number To Decimal String(number=w723) -> (decimal integer string=w736:string)  [unwired: 1 in]
                        n460 = Number To Decimal String(number=w722) -> (decimal integer string=w735:string)  [unwired: 1 in]
                        n461 = Build Array(w726, w725, w737, w736, w735) -> (w734:string[])
                        n462 = TDMS Set Properties(5:w734, 7:w728, 11:w738) -> ()  [unwired: 3 in, 4 out]
                      }
                      frame #3 {
                        w740 = 0.0
                        n463 = local read "DISP LAB02-2"() -> (w742:T4)
                        n464 = Bundle(cluster=w742, "CYCLE"=w740, "MINS"=w740, "STATUS"="RUN") -> (w741:T4)
                        n465 = local write "DISP LAB02-2"(w741) -> ()
                      }
                      frame #4 {
                        n466 = local read "SIG LAB02-2"() -> (w745:T2)
                        n467 = local read "TEMP START LAB02-2"() -> (w747:cluster{"TL":dbl, "TN":dbl})
                        n468 = Unbundle(w745) -> ("Tmp Live"=w744:dbl, "Tmp Neut"=w743:dbl)  [unwired: 3 out]
                        n469 = Bundle(cluster=w747, "TL"=w744, "TN"=w743) -> (w746:cluster{"TL":dbl, "TN":dbl})
                        n470 = local write "TEMP START LAB02-2"(w746) -> ()
                      }
                    }
                  }
                }
              }
              event "RUN LAB03-1": Value Change {
                n471 = event-data() -> ("NewVal"=w750:bool)  [unwired: 1 in, 5 out]
                n472 = case shown="False" w750 {
                  tunnel: w754 -> [_ w784]
                  tunnel: w753 -> [_ w783]
                  tunnel: w751 -> [w756 w782]
                  tunnel: w752 -> [_ w781]
                  tunnel: w749 -> [_ w780]
                  tunnel: [w755 w779] -> w748
                  frame False {
                    # "stop test"
                    n473 = stacked-sequence {
                      tunnel: w756 -> [w765 _]
                      tunnel: [w757 _] -> w755
                      frame #0 {
                        n474 = local read "DISP LAB03-1"() -> (w764:T4)
                        n475 = Unbundle(w764) -> ("CYCLE"=w762:dbl, "MINS"=w763:dbl)  [unwired: 1 out]
                        n476 = case shown="\"CYCLE TEST\"" w765 {
                          tunnel: w763 -> [_ _ w772]
                          tunnel: w762 -> [w770 w771 _]
                          tunnel: [w770 w771 w772] -> w761
                          frame "CHART TEST", Default {
                          }
                          frame "CYCLE TEST" {
                          }
                          frame "T-RISE TEST" {
                          }
                        }
                        n477 = local read "TDMS LAB03-1"() -> (w769:refnum<k34>)
                        n478 = Build Array("STOPPED") -> (w766:string[])
                        n479 = Build Array(w761) -> (w760:dbl[])
                        n480 = TDMS Write(0:w769, 5:"TEST RESULT", 7:w766, 9:w760) -> (4:w758:refnum<k34>, 15:w759:errorcluster)  [unwired: 2 in, 2 out]
                        n481 = TDMS Close(8:w759, 11:w758) -> (0:w757:errorcluster)  [unwired: 1 out]
                      }
                      frame #1 {
                        n482 = local read "DISP LAB03-1"() -> (w778:T4)
                        n483 = Bundle(cluster=w778, "STATUS"="STOP") -> (w776:T4)  [unwired: 2 in]
                        n484 = call "Save data file to network drive v1.vi"("panel id"="LAB03-1") -> ("network file save error"=w773:errorcluster)  [unwired: 9 in, 1 out]
                        n485 = local write "RESULT LAB03-1"(FALSE) -> ()
                        n486 = local write "data file error"(w773) -> ()
                        n487 = local write "DISP LAB03-1"(w776) -> ()
                      }
                    }
                  }
                  frame True {
                    # "start new test and create test file"
                    n488 = stacked-sequence {
                      seq-local: [w785 _ _ _ _] -> [_ w810 _ _ _]
                      tunnel: w784 -> [w790 _ _ _ _]
                      tunnel: w783 -> [w787 _ _ _ _]
                      tunnel: w782 -> [w800 _ _ _ _]
                      tunnel: w781 -> [w793 _ _ _ _]
                      tunnel: w780 -> [w788 _ _ _ _]
                      tunnel: [_ w804 _ _ _] -> w779
                      frame #0 {
                        w786 = "\\"
                        n489 = local read "SET LAB03-1"() -> (w795:T5)
                        n490 = case shown="\"CHART TEST\", Default" w800 {
                          tunnel: ["CHART TEST-" "CYCLE TEST-" "T-RISE TEST-"] -> w796
                          frame "CHART TEST", Default {
                          }
                          frame "CYCLE TEST" {
                          }
                          frame "T-RISE TEST" {
                          }
                        }
                        n491 = Unbundle(w795) -> ("DESCRIPTION"=w794:string)  [unwired: 4 out]
                        n492 = Concatenate Strings(w790, "LAB03-1\\", w788, w786, w787, w786) -> (w797:string)
                        n493 = String To Path(string=w797) -> (path=w799:path)
                        n494 = Concatenate Strings(w797, w796, w794, "-", w793, ".tdms") -> (w785:string)
                        n495 = Create Folder(path (use dialog)=w799) -> (error out=w798:errorcluster)  [unwired: 2 in, 2 out]
                        n496 = global write "Global 1.vi" "LAB03-1 FILE"(w785) -> ()
                        n497 = call <vilib>:"Clear Errors.vi"("error in (no error)"=w798) -> ()  [unwired: 6 in, 1 out]
                      }
                      frame #1 {
                        n498 = String To Path(string=w810) -> (path=w805:path)
                        n499 = TDMS Open(5:FALSE, 6:FALSE, 10:T15."create or replace" ("operation (0:open)"), 11:w805) -> (0:w804:errorcluster, 3:→"TDMS LAB03-1":refnum<k34>)  [unwired: 3 in]
                      }
                      frame #2 {
                        n500 = local read "SET LAB03-1"() -> (w816:T5)
                        n501 = local read "TDMS LAB03-1"() -> (w827:refnum<k34>)
                        n502 = Build Array("Testers Name", "Description", "Set Test Cycles", "T-Rise minutes", "T-Rise Deg C") -> (w817:string[])
                        n503 = Unbundle(w816) -> ("NAME"=w815:string, "DESCRIPTION"=w814:string, "CYCLES"=w813:dbl, "T-RISE mins"=w812:dbl, "T-RISE deg C"=w811:dbl)
                        n504 = Number To Decimal String(number=w813) -> (decimal integer string=w826:string)  [unwired: 1 in]
                        n505 = Number To Decimal String(number=w812) -> (decimal integer string=w825:string)  [unwired: 1 in]
                        n506 = Number To Decimal String(number=w811) -> (decimal integer string=w824:string)  [unwired: 1 in]
                        n507 = Build Array(w815, w814, w826, w825, w824) -> (w823:string[])
                        n508 = TDMS Set Properties(5:w823, 7:w817, 11:w827) -> ()  [unwired: 3 in, 4 out]
                      }
                      frame #3 {
                        w829 = 0.0
                        n509 = local read "DISP LAB03-1"() -> (w831:T4)
                        n510 = Bundle(cluster=w831, "CYCLE"=w829, "MINS"=w829, "STATUS"="RUN") -> (w830:T4)
                        n511 = local write "DISP LAB03-1"(w830) -> ()
                      }
                      frame #4 {
                        n512 = local read "SIG LAB03-1"() -> (w834:T2)
                        n513 = local read "TEMP START LAB03-1"() -> (w836:cluster{"TL":dbl, "TN":dbl})
                        n514 = Unbundle(w834) -> ("Tmp Live"=w833:dbl, "Tmp Neut"=w832:dbl)  [unwired: 3 out]
                        n515 = Bundle(cluster=w836, "TL"=w833, "TN"=w832) -> (w835:cluster{"TL":dbl, "TN":dbl})
                        n516 = local write "TEMP START LAB03-1"(w835) -> ()
                      }
                    }
                  }
                }
              }
              event "RUN LAB03-2": Value Change {
                n517 = event-data() -> ("NewVal"=w839:bool)  [unwired: 1 in, 5 out]
                n518 = case shown="False" w839 {
                  tunnel: w843 -> [_ w873]
                  tunnel: w842 -> [_ w872]
                  tunnel: w840 -> [w845 w871]
                  tunnel: w841 -> [_ w870]
                  tunnel: w838 -> [_ w869]
                  tunnel: [w844 w868] -> w837
                  frame False {
                    # "stop test"
                    n519 = stacked-sequence {
                      tunnel: w845 -> [w854 _]
                      tunnel: [w846 _] -> w844
                      frame #0 {
                        n520 = local read "DISP LAB03-2"() -> (w853:T4)
                        n521 = Unbundle(w853) -> ("CYCLE"=w851:dbl, "MINS"=w852:dbl)  [unwired: 1 out]
                        n522 = case shown="\"CYCLE TEST\"" w854 {
                          tunnel: w852 -> [_ _ w861]
                          tunnel: w851 -> [w859 w860 _]
                          tunnel: [w859 w860 w861] -> w850
                          frame "CHART TEST", Default {
                          }
                          frame "CYCLE TEST" {
                          }
                          frame "T-RISE TEST" {
                          }
                        }
                        n523 = local read "TDMS LAB03-2"() -> (w858:refnum<k34>)
                        n524 = Build Array("STOPPED") -> (w855:string[])
                        n525 = Build Array(w850) -> (w849:dbl[])
                        n526 = TDMS Write(0:w858, 5:"TEST RESULT", 7:w855, 9:w849) -> (4:w847:refnum<k34>, 15:w848:errorcluster)  [unwired: 2 in, 2 out]
                        n527 = TDMS Close(8:w848, 11:w847) -> (0:w846:errorcluster)  [unwired: 1 out]
                      }
                      frame #1 {
                        n528 = local read "DISP LAB03-2"() -> (w867:T4)
                        n529 = Bundle(cluster=w867, "STATUS"="STOP") -> (w865:T4)  [unwired: 2 in]
                        n530 = call "Save data file to network drive v1.vi"("panel id"="LAB03-2") -> ("network file save error"=w862:errorcluster)  [unwired: 9 in, 1 out]
                        n531 = local write "RESULT LAB03-2"(FALSE) -> ()
                        n532 = local write "DISP LAB03-2"(w865) -> ()
                        n533 = local write "data file error"(w862) -> ()
                      }
                    }
                  }
                  frame True {
                    # "start new test and create test file"
                    n534 = stacked-sequence {
                      seq-local: [w874 _ _ _ _] -> [_ w899 _ _ _]
                      tunnel: w873 -> [w879 _ _ _ _]
                      tunnel: w872 -> [w876 _ _ _ _]
                      tunnel: w871 -> [w889 _ _ _ _]
                      tunnel: w870 -> [w882 _ _ _ _]
                      tunnel: w869 -> [w877 _ _ _ _]
                      tunnel: [_ w893 _ _ _] -> w868
                      frame #0 {
                        w875 = "\\"
                        n535 = local read "SET LAB03-2"() -> (w884:T5)
                        n536 = case shown="\"CHART TEST\", Default" w889 {
                          tunnel: ["CHART TEST-" "CYCLE TEST-" "T-RISE TEST-"] -> w885
                          frame "CHART TEST", Default {
                          }
                          frame "CYCLE TEST" {
                          }
                          frame "T-RISE TEST" {
                          }
                        }
                        n537 = Unbundle(w884) -> ("DESCRIPTION"=w883:string)  [unwired: 4 out]
                        n538 = Concatenate Strings(w879, "LAB03-2\\", w877, w875, w876, w875) -> (w886:string)
                        n539 = String To Path(string=w886) -> (path=w888:path)
                        n540 = Concatenate Strings(w886, w885, w883, "-", w882, ".tdms") -> (w874:string)
                        n541 = Create Folder(path (use dialog)=w888) -> (error out=w887:errorcluster)  [unwired: 2 in, 2 out]
                        n542 = global write "Global 1.vi" "LAB03-2 FILE"(w874) -> ()
                        n543 = call <vilib>:"Clear Errors.vi"("error in (no error)"=w887) -> ()  [unwired: 6 in, 1 out]
                      }
                      frame #1 {
                        n544 = String To Path(string=w899) -> (path=w894:path)
                        n545 = TDMS Open(5:FALSE, 6:FALSE, 10:T15."create or replace" ("operation (0:open)"), 11:w894) -> (0:w893:errorcluster, 3:→"TDMS LAB03-2":refnum<k34>)  [unwired: 3 in]
                      }
                      frame #2 {
                        n546 = local read "SET LAB03-2"() -> (w905:T5)
                        n547 = local read "TDMS LAB03-2"() -> (w916:refnum<k34>)
                        n548 = Build Array("Testers Name", "Description", "Set Test Cycles", "T-Rise minutes", "T-Rise Deg C") -> (w906:string[])
                        n549 = Unbundle(w905) -> ("NAME"=w904:string, "DESCRIPTION"=w903:string, "CYCLES"=w902:dbl, "T-RISE mins"=w901:dbl, "T-RISE deg C"=w900:dbl)
                        n550 = Number To Decimal String(number=w902) -> (decimal integer string=w915:string)  [unwired: 1 in]
                        n551 = Number To Decimal String(number=w901) -> (decimal integer string=w914:string)  [unwired: 1 in]
                        n552 = Number To Decimal String(number=w900) -> (decimal integer string=w913:string)  [unwired: 1 in]
                        n553 = Build Array(w904, w903, w915, w914, w913) -> (w912:string[])
                        n554 = TDMS Set Properties(5:w912, 7:w906, 11:w916) -> ()  [unwired: 3 in, 4 out]
                      }
                      frame #3 {
                        w918 = 0.0
                        n555 = local read "DISP LAB03-2"() -> (w920:T4)
                        n556 = Bundle(cluster=w920, "CYCLE"=w918, "MINS"=w918, "STATUS"="RUN") -> (w919:T4)
                        n557 = local write "DISP LAB03-2"(w919) -> ()
                      }
                      frame #4 {
                        n558 = local read "SIG LAB03-2"() -> (w923:T2)
                        n559 = local read "TEMP START LAB03-2"() -> (w925:cluster{"TL":dbl, "TN":dbl})
                        n560 = Unbundle(w923) -> ("Tmp Live"=w922:dbl, "Tmp Neut"=w921:dbl)  [unwired: 3 out]
                        n561 = Bundle(cluster=w925, "TL"=w922, "TN"=w921) -> (w924:cluster{"TL":dbl, "TN":dbl})
                        n562 = local write "TEMP START LAB03-2"(w924) -> ()
                      }
                    }
                  }
                }
              }
              event "RUN LAB04-1": Value Change {
                n563 = event-data() -> ("NewVal"=w928:bool)  [unwired: 1 in, 5 out]
                n564 = case shown="False" w928 {
                  tunnel: w932 -> [_ w962]
                  tunnel: w931 -> [_ w961]
                  tunnel: w929 -> [w934 w960]
                  tunnel: w930 -> [_ w959]
                  tunnel: w927 -> [_ w958]
                  tunnel: [w933 w957] -> w926
                  frame False {
                    # "stop test"
                    n565 = stacked-sequence {
                      tunnel: w934 -> [w943 _]
                      tunnel: [w935 _] -> w933
                      frame #0 {
                        n566 = local read "DISP LAB04-1"() -> (w942:T4)
                        n567 = Unbundle(w942) -> ("CYCLE"=w940:dbl, "MINS"=w941:dbl)  [unwired: 1 out]
                        n568 = case shown="\"CYCLE TEST\"" w943 {
                          tunnel: w941 -> [_ _ w950]
                          tunnel: w940 -> [w948 w949 _]
                          tunnel: [w948 w949 w950] -> w939
                          frame "CHART TEST", Default {
                          }
                          frame "CYCLE TEST" {
                          }
                          frame "T-RISE TEST" {
                          }
                        }
                        n569 = local read "TDMS LAB04-1"() -> (w947:refnum<k34>)
                        n570 = Build Array("STOPPED") -> (w944:string[])
                        n571 = Build Array(w939) -> (w938:dbl[])
                        n572 = TDMS Write(0:w947, 5:"TEST RESULT", 7:w944, 9:w938) -> (4:w936:refnum<k34>, 15:w937:errorcluster)  [unwired: 2 in, 2 out]
                        n573 = TDMS Close(8:w937, 11:w936) -> (0:w935:errorcluster)  [unwired: 1 out]
                      }
                      frame #1 {
                        n574 = local read "DISP LAB04-1"() -> (w956:T4)
                        n575 = Bundle(cluster=w956, "STATUS"="STOP") -> (w954:T4)  [unwired: 2 in]
                        n576 = call "Save data file to network drive v1.vi"("panel id"="LAB04-1") -> ("network file save error"=w951:errorcluster)  [unwired: 9 in, 1 out]
                        n577 = local write "RESULT LAB04-1"(FALSE) -> ()
                        n578 = local write "DISP LAB04-1"(w954) -> ()
                        n579 = local write "data file error"(w951) -> ()
                      }
                    }
                  }
                  frame True {
                    # "start new test and create test file"
                    n580 = stacked-sequence {
                      seq-local: [w963 _ _ _ _] -> [_ w988 _ _ _]
                      tunnel: w962 -> [w968 _ _ _ _]
                      tunnel: w961 -> [w964 _ _ _ _]
                      tunnel: w960 -> [w978 _ _ _ _]
                      tunnel: w959 -> [w971 _ _ _ _]
                      tunnel: w958 -> [w966 _ _ _ _]
                      tunnel: [_ w982 _ _ _] -> w957
                      frame #0 {
                        w965 = "\\"
                        n581 = local read "SET LAB04-1"() -> (w973:T5)
                        n582 = case shown="\"CHART TEST\", Default" w978 {
                          tunnel: ["CHART TEST-" "CYCLE TEST-" "T-RISE TEST-"] -> w974
                          frame "CHART TEST", Default {
                          }
                          frame "CYCLE TEST" {
                          }
                          frame "T-RISE TEST" {
                          }
                        }
                        n583 = Unbundle(w973) -> ("DESCRIPTION"=w972:string)  [unwired: 4 out]
                        n584 = Concatenate Strings(w968, "LAB04-1\\", w966, w965, w964, w965) -> (w975:string)
                        n585 = String To Path(string=w975) -> (path=w977:path)
                        n586 = Concatenate Strings(w975, w974, w972, "-", w971, ".tdms") -> (w963:string)
                        n587 = Create Folder(path (use dialog)=w977) -> (error out=w976:errorcluster)  [unwired: 2 in, 2 out]
                        n588 = global write "Global 1.vi" "LAB04-1 FILE"(w963) -> ()
                        n589 = call <vilib>:"Clear Errors.vi"("error in (no error)"=w976) -> ()  [unwired: 6 in, 1 out]
                      }
                      frame #1 {
                        n590 = String To Path(string=w988) -> (path=w983:path)
                        n591 = TDMS Open(5:FALSE, 6:FALSE, 10:T15."create or replace" ("operation (0:open)"), 11:w983) -> (0:w982:errorcluster, 3:→"TDMS LAB04-1":refnum<k34>)  [unwired: 3 in]
                      }
                      frame #2 {
                        n592 = local read "SET LAB04-1"() -> (w994:T5)
                        n593 = local read "TDMS LAB04-1"() -> (w1005:refnum<k34>)
                        n594 = Build Array("Testers Name", "Description", "Set Test Cycles", "T-Rise minutes", "T-Rise Deg C") -> (w995:string[])
                        n595 = Unbundle(w994) -> ("NAME"=w993:string, "DESCRIPTION"=w992:string, "CYCLES"=w991:dbl, "T-RISE mins"=w990:dbl, "T-RISE deg C"=w989:dbl)
                        n596 = Number To Decimal String(number=w991) -> (decimal integer string=w1004:string)  [unwired: 1 in]
                        n597 = Number To Decimal String(number=w990) -> (decimal integer string=w1003:string)  [unwired: 1 in]
                        n598 = Number To Decimal String(number=w989) -> (decimal integer string=w1002:string)  [unwired: 1 in]
                        n599 = Build Array(w993, w992, w1004, w1003, w1002) -> (w1001:string[])
                        n600 = TDMS Set Properties(5:w1001, 7:w995, 11:w1005) -> ()  [unwired: 3 in, 4 out]
                      }
                      frame #3 {
                        w1007 = 0.0
                        n601 = local read "DISP LAB04-1"() -> (w1009:T4)
                        n602 = Bundle(cluster=w1009, "CYCLE"=w1007, "MINS"=w1007, "STATUS"="RUN") -> (w1008:T4)
                        n603 = local write "DISP LAB04-1"(w1008) -> ()
                      }
                      frame #4 {
                        n604 = local read "SIG LAB04-1"() -> (w1012:T2)
                        n605 = local read "TEMP START LAB04-1"() -> (w1014:cluster{"TL":dbl, "TN":dbl})
                        n606 = Unbundle(w1012) -> ("Tmp Live"=w1011:dbl, "Tmp Neut"=w1010:dbl)  [unwired: 3 out]
                        n607 = Bundle(cluster=w1014, "TL"=w1011, "TN"=w1010) -> (w1013:cluster{"TL":dbl, "TN":dbl})
                        n608 = local write "TEMP START LAB04-1"(w1013) -> ()
                      }
                    }
                  }
                }
              }
              event "RUN LAB04-2": Value Change {
                n609 = event-data() -> ("NewVal"=w1017:bool)  [unwired: 1 in, 5 out]
                n610 = case shown="False" w1017 {
                  tunnel: w1021 -> [_ w1051]
                  tunnel: w1020 -> [_ w1050]
                  tunnel: w1018 -> [w1023 w1049]
                  tunnel: w1019 -> [_ w1048]
                  tunnel: w1016 -> [_ w1047]
                  tunnel: [w1022 w1046] -> w1015
                  frame False {
                    # "stop test"
                    n611 = stacked-sequence {
                      tunnel: w1023 -> [w1032 _]
                      tunnel: [w1024 _] -> w1022
                      frame #0 {
                        n612 = local read "DISP LAB04-2"() -> (w1031:T4)
                        n613 = Unbundle(w1031) -> ("CYCLE"=w1029:dbl, "MINS"=w1030:dbl)  [unwired: 1 out]
                        n614 = case shown="\"CYCLE TEST\"" w1032 {
                          tunnel: w1030 -> [_ _ w1039]
                          tunnel: w1029 -> [w1037 w1038 _]
                          tunnel: [w1037 w1038 w1039] -> w1028
                          frame "CHART TEST", Default {
                          }
                          frame "CYCLE TEST" {
                          }
                          frame "T-RISE TEST" {
                          }
                        }
                        n615 = local read "TDMS LAB04-2"() -> (w1036:refnum<k34>)
                        n616 = Build Array("STOPPED") -> (w1033:string[])
                        n617 = Build Array(w1028) -> (w1027:dbl[])
                        n618 = TDMS Write(0:w1036, 5:"TEST RESULT", 7:w1033, 9:w1027) -> (4:w1025:refnum<k34>, 15:w1026:errorcluster)  [unwired: 2 in, 2 out]
                        n619 = TDMS Close(8:w1026, 11:w1025) -> (0:w1024:errorcluster)  [unwired: 1 out]
                      }
                      frame #1 {
                        n620 = local read "DISP LAB04-2"() -> (w1045:T4)
                        n621 = Bundle(cluster=w1045, "STATUS"="STOP") -> (w1043:T4)  [unwired: 2 in]
                        n622 = call "Save data file to network drive v1.vi"("panel id"="LAB04-2") -> ("network file save error"=w1040:errorcluster)  [unwired: 9 in, 1 out]
                        n623 = local write "RESULT LAB04-2"(FALSE) -> ()
                        n624 = local write "DISP LAB04-2"(w1043) -> ()
                        n625 = local write "data file error"(w1040) -> ()
                      }
                    }
                  }
                  frame True {
                    # "start new test and create test file"
                    n626 = stacked-sequence {
                      seq-local: [w1052 _ _ _ _] -> [_ w1077 _ _ _]
                      tunnel: w1051 -> [w1057 _ _ _ _]
                      tunnel: w1050 -> [w1053 _ _ _ _]
                      tunnel: w1049 -> [w1067 _ _ _ _]
                      tunnel: w1048 -> [w1060 _ _ _ _]
                      tunnel: w1047 -> [w1055 _ _ _ _]
                      tunnel: [_ w1071 _ _ _] -> w1046
                      frame #0 {
                        w1054 = "\\"
                        n627 = local read "SET LAB04-2"() -> (w1062:T5)
                        n628 = case shown="\"CHART TEST\", Default" w1067 {
                          tunnel: ["CHART TEST-" "CYCLE TEST-" "T-RISE TEST-"] -> w1063
                          frame "CHART TEST", Default {
                          }
                          frame "CYCLE TEST" {
                          }
                          frame "T-RISE TEST" {
                          }
                        }
                        n629 = Unbundle(w1062) -> ("DESCRIPTION"=w1061:string)  [unwired: 4 out]
                        n630 = Concatenate Strings(w1057, "LAB04-2\\", w1055, w1054, w1053, w1054) -> (w1064:string)
                        n631 = String To Path(string=w1064) -> (path=w1066:path)
                        n632 = Concatenate Strings(w1064, w1063, w1061, "-", w1060, ".tdms") -> (w1052:string)
                        n633 = Create Folder(path (use dialog)=w1066) -> (error out=w1065:errorcluster)  [unwired: 2 in, 2 out]
                        n634 = global write "Global 1.vi" "LAB04-2 FILE"(w1052) -> ()
                        n635 = call <vilib>:"Clear Errors.vi"("error in (no error)"=w1065) -> ()  [unwired: 6 in, 1 out]
                      }
                      frame #1 {
                        n636 = String To Path(string=w1077) -> (path=w1072:path)
                        n637 = TDMS Open(5:FALSE, 6:FALSE, 10:T15."create or replace" ("operation (0:open)"), 11:w1072) -> (0:w1071:errorcluster, 3:→"TDMS LAB04-2":refnum<k34>)  [unwired: 3 in]
                      }
                      frame #2 {
                        n638 = local read "SET LAB04-2"() -> (w1083:T5)
                        n639 = local read "TDMS LAB04-2"() -> (w1094:refnum<k34>)
                        n640 = Build Array("Testers Name", "Description", "Set Test Cycles", "T-Rise minutes", "T-Rise Deg C") -> (w1084:string[])
                        n641 = Unbundle(w1083) -> ("NAME"=w1082:string, "DESCRIPTION"=w1081:string, "CYCLES"=w1080:dbl, "T-RISE mins"=w1079:dbl, "T-RISE deg C"=w1078:dbl)
                        n642 = Number To Decimal String(number=w1080) -> (decimal integer string=w1093:string)  [unwired: 1 in]
                        n643 = Number To Decimal String(number=w1079) -> (decimal integer string=w1092:string)  [unwired: 1 in]
                        n644 = Number To Decimal String(number=w1078) -> (decimal integer string=w1091:string)  [unwired: 1 in]
                        n645 = Build Array(w1082, w1081, w1093, w1092, w1091) -> (w1090:string[])
                        n646 = TDMS Set Properties(5:w1090, 7:w1084, 11:w1094) -> ()  [unwired: 3 in, 4 out]
                      }
                      frame #3 {
                        w1096 = 0.0
                        n647 = local read "DISP LAB04-2"() -> (w1098:T4)
                        n648 = Bundle(cluster=w1098, "CYCLE"=w1096, "MINS"=w1096, "STATUS"="RUN") -> (w1097:T4)
                        n649 = local write "DISP LAB04-2"(w1097) -> ()
                      }
                      frame #4 {
                        n650 = local read "SIG LAB04-2"() -> (w1101:T2)
                        n651 = local read "TEMP START LAB04-2"() -> (w1103:cluster{"TL":dbl, "TN":dbl})
                        n652 = Unbundle(w1101) -> ("Tmp Live"=w1100:dbl, "Tmp Neut"=w1099:dbl)  [unwired: 3 out]
                        n653 = Bundle(cluster=w1103, "TL"=w1100, "TN"=w1099) -> (w1102:cluster{"TL":dbl, "TN":dbl})
                        n654 = local write "TEMP START LAB04-2"(w1102) -> ()
                      }
                    }
                  }
                }
              }
              event "RUN LAB05-1": Value Change {
                n655 = event-data() -> ("NewVal"=w1106:bool)  [unwired: 1 in, 5 out]
                n656 = case shown="False" w1106 {
                  tunnel: w1110 -> [_ w1140]
                  tunnel: w1109 -> [_ w1139]
                  tunnel: w1107 -> [w1112 w1138]
                  tunnel: w1108 -> [_ w1137]
                  tunnel: w1105 -> [_ w1136]
                  tunnel: [w1111 w1135] -> w1104
                  frame False {
                    # "stop test"
                    n657 = stacked-sequence {
                      tunnel: w1112 -> [w1121 _]
                      tunnel: [w1113 _] -> w1111
                      frame #0 {
                        n658 = local read "DISP LAB05-1"() -> (w1120:T4)
                        n659 = Unbundle(w1120) -> ("CYCLE"=w1118:dbl, "MINS"=w1119:dbl)  [unwired: 1 out]
                        n660 = case shown="\"CYCLE TEST\"" w1121 {
                          tunnel: w1119 -> [_ _ w1128]
                          tunnel: w1118 -> [w1126 w1127 _]
                          tunnel: [w1126 w1127 w1128] -> w1117
                          frame "CHART TEST", Default {
                          }
                          frame "CYCLE TEST" {
                          }
                          frame "T-RISE TEST" {
                          }
                        }
                        n661 = local read "TDMS LAB05-1"() -> (w1125:refnum<k34>)
                        n662 = Build Array("STOPPED") -> (w1122:string[])
                        n663 = Build Array(w1117) -> (w1116:dbl[])
                        n664 = TDMS Write(0:w1125, 5:"TEST RESULT", 7:w1122, 9:w1116) -> (4:w1114:refnum<k34>, 15:w1115:errorcluster)  [unwired: 2 in, 2 out]
                        n665 = TDMS Close(8:w1115, 11:w1114) -> (0:w1113:errorcluster)  [unwired: 1 out]
                      }
                      frame #1 {
                        n666 = local read "DISP LAB05-1"() -> (w1134:T4)
                        n667 = Bundle(cluster=w1134, "STATUS"="STOP") -> (w1132:T4)  [unwired: 2 in]
                        n668 = call "Save data file to network drive v1.vi"("panel id"="LAB05-1") -> ("network file save error"=w1129:errorcluster)  [unwired: 9 in, 1 out]
                        n669 = local write "RESULT LAB05-1"(FALSE) -> ()
                        n670 = local write "DISP LAB05-1"(w1132) -> ()
                        n671 = local write "data file error"(w1129) -> ()
                      }
                    }
                  }
                  frame True {
                    # "start new test and create test file"
                    n672 = stacked-sequence {
                      seq-local: [w1141 _ _ _ _] -> [_ w1166 _ _ _]
                      tunnel: w1140 -> [w1146 _ _ _ _]
                      tunnel: w1139 -> [w1142 _ _ _ _]
                      tunnel: w1138 -> [w1156 _ _ _ _]
                      tunnel: w1137 -> [w1149 _ _ _ _]
                      tunnel: w1136 -> [w1144 _ _ _ _]
                      tunnel: [_ w1160 _ _ _] -> w1135
                      frame #0 {
                        w1143 = "\\"
                        n673 = local read "SET LAB05-1"() -> (w1151:T5)
                        n674 = case shown="\"CHART TEST\", Default" w1156 {
                          tunnel: ["CHART TEST-" "CYCLE TEST-" "T-RISE TEST-"] -> w1152
                          frame "CHART TEST", Default {
                          }
                          frame "CYCLE TEST" {
                          }
                          frame "T-RISE TEST" {
                          }
                        }
                        n675 = Unbundle(w1151) -> ("DESCRIPTION"=w1150:string)  [unwired: 4 out]
                        n676 = Concatenate Strings(w1146, "LAB05-1\\", w1144, w1143, w1142, w1143) -> (w1153:string)
                        n677 = String To Path(string=w1153) -> (path=w1155:path)
                        n678 = Concatenate Strings(w1153, w1152, w1150, "-", w1149, ".tdms") -> (w1141:string)
                        n679 = Create Folder(path (use dialog)=w1155) -> (error out=w1154:errorcluster)  [unwired: 2 in, 2 out]
                        n680 = global write "Global 1.vi" "LAB05-1 FILE"(w1141) -> ()
                        n681 = call <vilib>:"Clear Errors.vi"("error in (no error)"=w1154) -> ()  [unwired: 6 in, 1 out]
                      }
                      frame #1 {
                        n682 = String To Path(string=w1166) -> (path=w1161:path)
                        n683 = TDMS Open(5:FALSE, 6:FALSE, 10:T15."create or replace" ("operation (0:open)"), 11:w1161) -> (0:w1160:errorcluster, 3:→"TDMS LAB05-1":refnum<k34>)  [unwired: 3 in]
                      }
                      frame #2 {
                        n684 = local read "SET LAB05-1"() -> (w1172:T5)
                        n685 = local read "TDMS LAB05-1"() -> (w1183:refnum<k34>)
                        n686 = Build Array("Testers Name", "Description", "Set Test Cycles", "T-Rise minutes", "T-Rise Deg C") -> (w1173:string[])
                        n687 = Unbundle(w1172) -> ("NAME"=w1171:string, "DESCRIPTION"=w1170:string, "CYCLES"=w1169:dbl, "T-RISE mins"=w1168:dbl, "T-RISE deg C"=w1167:dbl)
                        n688 = Number To Decimal String(number=w1169) -> (decimal integer string=w1182:string)  [unwired: 1 in]
                        n689 = Number To Decimal String(number=w1168) -> (decimal integer string=w1181:string)  [unwired: 1 in]
                        n690 = Number To Decimal String(number=w1167) -> (decimal integer string=w1180:string)  [unwired: 1 in]
                        n691 = Build Array(w1171, w1170, w1182, w1181, w1180) -> (w1179:string[])
                        n692 = TDMS Set Properties(5:w1179, 7:w1173, 11:w1183) -> ()  [unwired: 3 in, 4 out]
                      }
                      frame #3 {
                        w1185 = 0.0
                        n693 = local read "DISP LAB05-1"() -> (w1187:T4)
                        n694 = Bundle(cluster=w1187, "CYCLE"=w1185, "MINS"=w1185, "STATUS"="RUN") -> (w1186:T4)
                        n695 = local write "DISP LAB05-1"(w1186) -> ()
                      }
                      frame #4 {
                        n696 = local read "SIG LAB05-1"() -> (w1190:T2)
                        n697 = local read "TEMP START LAB05-1"() -> (w1192:cluster{"TL":dbl, "TN":dbl})
                        n698 = Unbundle(w1190) -> ("Tmp Live"=w1189:dbl, "Tmp Neut"=w1188:dbl)  [unwired: 3 out]
                        n699 = Bundle(cluster=w1192, "TL"=w1189, "TN"=w1188) -> (w1191:cluster{"TL":dbl, "TN":dbl})
                        n700 = local write "TEMP START LAB05-1"(w1191) -> ()
                      }
                    }
                  }
                }
              }
              event "RUN LAB05-2": Value Change {
                n701 = event-data() -> ("NewVal"=w1195:bool)  [unwired: 1 in, 5 out]
                n702 = case shown="False" w1195 {
                  tunnel: w1199 -> [_ w1229]
                  tunnel: w1198 -> [_ w1228]
                  tunnel: w1196 -> [w1201 w1227]
                  tunnel: w1197 -> [_ w1226]
                  tunnel: w1194 -> [_ w1225]
                  tunnel: [w1200 w1224] -> w1193
                  frame False {
                    # "stop test"
                    n703 = stacked-sequence {
                      tunnel: w1201 -> [w1210 _]
                      tunnel: [w1202 _] -> w1200
                      frame #0 {
                        n704 = local read "DISP LAB05-2"() -> (w1209:T4)
                        n705 = Unbundle(w1209) -> ("CYCLE"=w1207:dbl, "MINS"=w1208:dbl)  [unwired: 1 out]
                        n706 = case shown="\"CYCLE TEST\"" w1210 {
                          tunnel: w1208 -> [_ _ w1217]
                          tunnel: w1207 -> [w1215 w1216 _]
                          tunnel: [w1215 w1216 w1217] -> w1206
                          frame "CHART TEST", Default {
                          }
                          frame "CYCLE TEST" {
                          }
                          frame "T-RISE TEST" {
                          }
                        }
                        n707 = local read "TDMS LAB05-2"() -> (w1214:refnum<k34>)
                        n708 = Build Array("STOPPED") -> (w1211:string[])
                        n709 = Build Array(w1206) -> (w1205:dbl[])
                        n710 = TDMS Write(0:w1214, 5:"TEST RESULT", 7:w1211, 9:w1205) -> (4:w1203:refnum<k34>, 15:w1204:errorcluster)  [unwired: 2 in, 2 out]
                        n711 = TDMS Close(8:w1204, 11:w1203) -> (0:w1202:errorcluster)  [unwired: 1 out]
                      }
                      frame #1 {
                        n712 = local read "DISP LAB05-2"() -> (w1223:T4)
                        n713 = Bundle(cluster=w1223, "STATUS"="STOP") -> (w1221:T4)  [unwired: 2 in]
                        n714 = local write "RESULT LAB05-2"(FALSE) -> ()
                        n715 = local write "DISP LAB05-2"(w1221) -> ()
                        n716 = call "Save data file to network drive v1.vi"("panel id"="LAB05-2") -> ("network file save error"=w1218:errorcluster)  [unwired: 9 in, 1 out]
                        n717 = local write "data file error"(w1218) -> ()
                      }
                    }
                  }
                  frame True {
                    # "start new test and create test file"
                    n718 = stacked-sequence {
                      seq-local: [w1230 _ _ _ _] -> [_ w1255 _ _ _]
                      tunnel: w1229 -> [w1235 _ _ _ _]
                      tunnel: w1228 -> [w1231 _ _ _ _]
                      tunnel: w1227 -> [w1245 _ _ _ _]
                      tunnel: w1226 -> [w1238 _ _ _ _]
                      tunnel: w1225 -> [w1233 _ _ _ _]
                      tunnel: [_ w1249 _ _ _] -> w1224
                      frame #0 {
                        w1232 = "\\"
                        n719 = local read "SET LAB05-2"() -> (w1240:T5)
                        n720 = case shown="\"CHART TEST\", Default" w1245 {
                          tunnel: ["CHART TEST-" "CYCLE TEST-" "T-RISE TEST-"] -> w1241
                          frame "CHART TEST", Default {
                          }
                          frame "CYCLE TEST" {
                          }
                          frame "T-RISE TEST" {
                          }
                        }
                        n721 = Unbundle(w1240) -> ("DESCRIPTION"=w1239:string)  [unwired: 4 out]
                        n722 = Concatenate Strings(w1235, "LAB05-2\\", w1233, w1232, w1231, w1232) -> (w1242:string)
                        n723 = String To Path(string=w1242) -> (path=w1244:path)
                        n724 = Concatenate Strings(w1242, w1241, w1239, "-", w1238, ".tdms") -> (w1230:string)
                        n725 = Create Folder(path (use dialog)=w1244) -> (error out=w1243:errorcluster)  [unwired: 2 in, 2 out]
                        n726 = global write "Global 1.vi" "LAB05-2 FILE"(w1230) -> ()
                        n727 = call <vilib>:"Clear Errors.vi"("error in (no error)"=w1243) -> ()  [unwired: 6 in, 1 out]
                      }
                      frame #1 {
                        n728 = String To Path(string=w1255) -> (path=w1250:path)
                        n729 = TDMS Open(5:FALSE, 6:FALSE, 10:T15."create or replace" ("operation (0:open)"), 11:w1250) -> (0:w1249:errorcluster, 3:→"TDMS LAB05-2":refnum<k34>)  [unwired: 3 in]
                      }
                      frame #2 {
                        n730 = local read "SET LAB05-2"() -> (w1261:T5)
                        n731 = local read "TDMS LAB05-2"() -> (w1272:refnum<k34>)
                        n732 = Build Array("Testers Name", "Description", "Set Test Cycles", "T-Rise minutes", "T-Rise Deg C") -> (w1262:string[])
                        n733 = Unbundle(w1261) -> ("NAME"=w1260:string, "DESCRIPTION"=w1259:string, "CYCLES"=w1258:dbl, "T-RISE mins"=w1257:dbl, "T-RISE deg C"=w1256:dbl)
                        n734 = Number To Decimal String(number=w1258) -> (decimal integer string=w1271:string)  [unwired: 1 in]
                        n735 = Number To Decimal String(number=w1257) -> (decimal integer string=w1270:string)  [unwired: 1 in]
                        n736 = Number To Decimal String(number=w1256) -> (decimal integer string=w1269:string)  [unwired: 1 in]
                        n737 = Build Array(w1260, w1259, w1271, w1270, w1269) -> (w1268:string[])
                        n738 = TDMS Set Properties(5:w1268, 7:w1262, 11:w1272) -> ()  [unwired: 3 in, 4 out]
                      }
                      frame #3 {
                        w1274 = 0.0
                        n739 = local read "DISP LAB05-2"() -> (w1276:T4)
                        n740 = Bundle(cluster=w1276, "CYCLE"=w1274, "MINS"=w1274, "STATUS"="RUN") -> (w1275:T4)
                        n741 = local write "DISP LAB05-2"(w1275) -> ()
                      }
                      frame #4 {
                        n742 = local read "SIG LAB05-2"() -> (w1279:T2)
                        n743 = local read "TEMP START LAB05-2"() -> (w1281:cluster{"TL":dbl, "TN":dbl})
                        n744 = Unbundle(w1279) -> ("Tmp Live"=w1278:dbl, "Tmp Neut"=w1277:dbl)  [unwired: 3 out]
                        n745 = Bundle(cluster=w1281, "TL"=w1278, "TN"=w1277) -> (w1280:cluster{"TL":dbl, "TN":dbl})
                        n746 = local write "TEMP START LAB05-2"(w1280) -> ()
                      }
                    }
                  }
                }
              }
            }
            n747 = local write "data file error"(w362) -> ()
          }
          frame #4 {
            # "check if test cycles reached for cycle tests, if so then test pass"
            n748 = stacked-sequence {
              tunnel: w1301 -> [_ _ _ _ _ _ _ _ _ _]
              tunnel: w1300 -> [_ _ _ _ _ _ _ _ _ _]
              tunnel: w1299 -> [_ _ _ _ _ _ _ _ _ _]
              tunnel: w1298 -> [_ _ _ _ _ _ _ _ _ _]
              tunnel: w1297 -> [_ _ _ _ _ _ _ _ _ _]
              tunnel: w1296 -> [_ _ _ _ _ _ _ _ _ _]
              tunnel: w1295 -> [_ _ _ _ _ _ _ _ _ _]
              tunnel: w1294 -> [_ _ _ _ _ _ _ _ _ _]
              tunnel: w1293 -> [_ _ _ _ _ _ _ _ _ _]
              tunnel: w1292 -> [_ _ _ _ _ _ _ _ _ _]
              tunnel: w1291 -> [w1306 _ _ _ _ _ _ _ _ _]
              tunnel: w1290 -> [_ w1341 _ _ _ _ _ _ _ _]
              tunnel: w1289 -> [_ _ w1380 _ _ _ _ _ _ _]
              tunnel: w1288 -> [_ _ _ w1419 _ _ _ _ _ _]
              tunnel: w1287 -> [_ _ _ _ w1458 _ _ _ _ _]
              tunnel: w1286 -> [_ _ _ _ _ w1497 _ _ _ _]
              tunnel: w1285 -> [_ _ _ _ _ _ w1536 _ _ _]
              tunnel: w1284 -> [_ _ _ _ _ _ _ w1575 _ _]
              tunnel: w1283 -> [_ _ _ _ _ _ _ _ w1614 _]
              tunnel: w1282 -> [_ _ _ _ _ _ _ _ _ w1653]
              frame #0 {
                # "LAB01-1"
                n749 = Less?(x=w1306, y=2) -> (x < y?=w1304:bool)
                n750 = local read "DISP LAB01-1"() -> (w1307:T4)
                n751 = Unbundle(w1307) -> ("STATUS"=w1308:string)  [unwired: 2 out]
                n752 = Equal?(x=w1308, y="RUN") -> (x = y?=w1303:bool)
                n753 = And(x=w1303, y=w1304) -> (x .and. y?=w1302:bool)
                n754 = case shown="True" w1302 {
                  tunnel: w1307 -> [_ w1311]
                  tunnel: w1306 -> [_ w1316]
                  frame False {
                  }
                  frame True {
                    n755 = local read "SET LAB01-1"() -> (w1318:T5)
                    n756 = local read "TDMS LAB01-1"() -> (w1310:refnum<k34>)
                    n757 = Unbundle(w1311) -> ("CYCLE"=w1317:dbl)  [unwired: 2 out]
                    n758 = Unbundle(w1318) -> ("CYCLES"=w1313:dbl, "T-RISE mins"=w1315:dbl)  [unwired: 3 out]
                    n759 = case shown="\"CHART TEST\", Default" w1316 {
                      tunnel: w1315 -> [_ _ w1325]
                      tunnel: [w1320 w1322 w1325] -> w1314
                      tunnel: w1313 -> [w1320 w1322 _]
                      tunnel: ["CHART TEST" "CYCLES" "T-RISE TEST"] -> w1312
                      frame "CHART TEST", Default {
                      }
                      frame "CYCLE TEST" {
                      }
                      frame "T-RISE TEST" {
                      }
                    }
                    n760 = Greater Or Equal?(x=w1317, y=w1313) -> (x >= y?=w1319:bool)
                    n761 = case shown="True" w1319 {
                      tunnel: w1314 -> [w1329 _]
                      tunnel: w1312 -> [w1328 _]
                      tunnel: w1311 -> [w1327 _]
                      tunnel: w1310 -> [w1326 _]
                      frame True {
                        n762 = stacked-sequence {
                          tunnel: w1329 -> [w1333 _]
                          tunnel: w1328 -> [w1331 _]
                          tunnel: w1327 -> [_ w1339]
                          tunnel: w1326 -> [w1330 _]
                          frame #0 {
                            n763 = Build Array(w1331) -> (w1334:string[])
                            n764 = Build Array(w1333) -> (w1332:dbl[])
                            n765 = TDMS Write(0:w1330, 5:"TEST PASS", 7:w1334, 9:w1332) -> (15:w1336:errorcluster)  [unwired: 2 in, 3 out]
                            n766 = local write "data file error"(w1336) -> ()
                          }
                          frame #1 {
                            n767 = Bundle(cluster=w1339, "STATUS"="CYCLE PASS") -> (w1337:T4)  [unwired: 2 in]
                            n768 = local write "RESULT LAB01-1"(TRUE) -> ()
                            n769 = local write "DISP LAB01-1"(w1337) -> ()
                          }
                        }
                      }
                      frame False {
                      }
                    }
                  }
                }
              }
              frame #1 {
                # "LAB01-2"
                n770 = Less?(x=w1341, y=2) -> (x < y?=w1344:bool)
                n771 = local read "DISP LAB01-2"() -> (w1346:T4)
                n772 = Unbundle(w1346) -> ("STATUS"=w1347:string)  [unwired: 2 out]
                n773 = Equal?(x=w1347, y="RUN") -> (x = y?=w1343:bool)
                n774 = And(x=w1343, y=w1344) -> (x .and. y?=w1342:bool)
                n775 = case shown="True" w1342 {
                  tunnel: w1346 -> [_ w1350]
                  tunnel: w1341 -> [_ w1355]
                  frame False {
                  }
                  frame True {
                    n776 = local read "SET LAB01-2"() -> (w1357:T5)
                    n777 = local read "TDMS LAB01-2"() -> (w1349:refnum<k34>)
                    n778 = Unbundle(w1350) -> ("CYCLE"=w1356:dbl)  [unwired: 2 out]
                    n779 = Unbundle(w1357) -> ("CYCLES"=w1352:dbl, "T-RISE mins"=w1354:dbl)  [unwired: 3 out]
                    n780 = case shown="\"CHART TEST\", Default" w1355 {
                      tunnel: w1354 -> [_ _ w1364]
                      tunnel: [w1359 w1361 w1364] -> w1353
                      tunnel: w1352 -> [w1359 w1361 _]
                      tunnel: ["CHART TEST " "CYCLES" "T-RISE TEST"] -> w1351
                      frame "CHART TEST", Default {
                      }
                      frame "CYCLE TEST" {
                      }
                      frame "T-RISE TEST" {
                      }
                    }
                    n781 = Greater Or Equal?(x=w1356, y=w1352) -> (x >= y?=w1358:bool)
                    n782 = case shown="True" w1358 {
                      tunnel: w1353 -> [w1368 _]
                      tunnel: w1351 -> [w1367 _]
                      tunnel: w1350 -> [w1366 _]
                      tunnel: w1349 -> [w1365 _]
                      frame True {
                        n783 = stacked-sequence {
                          tunnel: w1368 -> [w1372 _]
                          tunnel: w1367 -> [w1370 _]
                          tunnel: w1366 -> [_ w1378]
                          tunnel: w1365 -> [w1369 _]
                          frame #0 {
                            n784 = Build Array(w1370) -> (w1373:string[])
                            n785 = Build Array(w1372) -> (w1371:dbl[])
                            n786 = TDMS Write(0:w1369, 5:"TEST PASS", 7:w1373, 9:w1371) -> (15:w1375:errorcluster)  [unwired: 2 in, 3 out]
                            n787 = local write "data file error"(w1375) -> ()
                          }
                          frame #1 {
                            n788 = Bundle(cluster=w1378, "STATUS"="CYCLE PASS") -> (w1376:T4)  [unwired: 2 in]
                            n789 = local write "RESULT LAB01-2"(TRUE) -> ()
                            n790 = local write "DISP LAB01-2"(w1376) -> ()
                          }
                        }
                      }
                      frame False {
                      }
                    }
                  }
                }
              }
              frame #2 {
                # "LAB02-1"
                n791 = Less?(x=w1380, y=2) -> (x < y?=w1383:bool)
                n792 = local read "DISP LAB02-1"() -> (w1385:T4)
                n793 = Unbundle(w1385) -> ("STATUS"=w1386:string)  [unwired: 2 out]
                n794 = Equal?(x=w1386, y="RUN") -> (x = y?=w1382:bool)
                n795 = And(x=w1382, y=w1383) -> (x .and. y?=w1381:bool)
                n796 = case shown="True" w1381 {
                  tunnel: w1385 -> [_ w1389]
                  tunnel: w1380 -> [_ w1394]
                  frame False {
                  }
                  frame True {
                    n797 = local read "SET LAB02-1"() -> (w1396:T5)
                    n798 = local read "TDMS LAB02-1"() -> (w1388:refnum<k34>)
                    n799 = Unbundle(w1389) -> ("CYCLE"=w1395:dbl)  [unwired: 2 out]
                    n800 = Unbundle(w1396) -> ("CYCLES"=w1391:dbl, "T-RISE mins"=w1393:dbl)  [unwired: 3 out]
                    n801 = case shown="\"CHART TEST\", Default" w1394 {
                      tunnel: w1393 -> [_ _ w1403]
                      tunnel: [w1398 w1400 w1403] -> w1392
                      tunnel: w1391 -> [w1398 w1400 _]
                      tunnel: ["CHART TEST" "CYCLES" "T-RISE TEST"] -> w1390
                      frame "CHART TEST", Default {
                      }
                      frame "CYCLE TEST" {
                      }
                      frame "T-RISE TEST" {
                      }
                    }
                    n802 = Greater Or Equal?(x=w1395, y=w1391) -> (x >= y?=w1397:bool)
                    n803 = case shown="True" w1397 {
                      tunnel: w1392 -> [w1407 _]
                      tunnel: w1390 -> [w1406 _]
                      tunnel: w1389 -> [w1405 _]
                      tunnel: w1388 -> [w1404 _]
                      frame True {
                        n804 = stacked-sequence {
                          tunnel: w1407 -> [w1411 _]
                          tunnel: w1406 -> [w1409 _]
                          tunnel: w1405 -> [_ w1417]
                          tunnel: w1404 -> [w1408 _]
                          frame #0 {
                            n805 = Build Array(w1409) -> (w1412:string[])
                            n806 = Build Array(w1411) -> (w1410:dbl[])
                            n807 = TDMS Write(0:w1408, 5:"TEST PASS", 7:w1412, 9:w1410) -> (15:w1414:errorcluster)  [unwired: 2 in, 3 out]
                            n808 = local write "data file error"(w1414) -> ()
                          }
                          frame #1 {
                            n809 = Bundle(cluster=w1417, "STATUS"="CYCLE PASS") -> (w1415:T4)  [unwired: 2 in]
                            n810 = local write "RESULT LAB02-1"(TRUE) -> ()
                            n811 = local write "DISP LAB02-1"(w1415) -> ()
                          }
                        }
                      }
                      frame False {
                      }
                    }
                  }
                }
              }
              frame #3 {
                # "LAB02-2"
                n812 = Less?(x=w1419, y=2) -> (x < y?=w1422:bool)
                n813 = local read "DISP LAB02-2"() -> (w1424:T4)
                n814 = Unbundle(w1424) -> ("STATUS"=w1425:string)  [unwired: 2 out]
                n815 = Equal?(x=w1425, y="RUN") -> (x = y?=w1421:bool)
                n816 = And(x=w1421, y=w1422) -> (x .and. y?=w1420:bool)
                n817 = case shown="True" w1420 {
                  tunnel: w1424 -> [_ w1428]
                  tunnel: w1419 -> [_ w1433]
                  frame False {
                  }
                  frame True {
                    n818 = local read "SET LAB02-2"() -> (w1435:T5)
                    n819 = local read "TDMS LAB02-2"() -> (w1427:refnum<k34>)
                    n820 = Unbundle(w1428) -> ("CYCLE"=w1434:dbl)  [unwired: 2 out]
                    n821 = Unbundle(w1435) -> ("CYCLES"=w1430:dbl, "T-RISE mins"=w1432:dbl)  [unwired: 3 out]
                    n822 = case shown="\"CHART TEST\", Default" w1433 {
                      tunnel: w1432 -> [_ _ w1442]
                      tunnel: [w1437 w1439 w1442] -> w1431
                      tunnel: w1430 -> [w1437 w1439 _]
                      tunnel: ["CHART TEST" "CYCLES" "T-RISE TEST"] -> w1429
                      frame "CHART TEST", Default {
                      }
                      frame "CYCLE TEST" {
                      }
                      frame "T-RISE TEST" {
                      }
                    }
                    n823 = Greater Or Equal?(x=w1434, y=w1430) -> (x >= y?=w1436:bool)
                    n824 = case shown="True" w1436 {
                      tunnel: w1431 -> [w1446 _]
                      tunnel: w1429 -> [w1445 _]
                      tunnel: w1428 -> [w1444 _]
                      tunnel: w1427 -> [w1443 _]
                      frame True {
                        n825 = stacked-sequence {
                          tunnel: w1446 -> [w1450 _]
                          tunnel: w1445 -> [w1448 _]
                          tunnel: w1444 -> [_ w1456]
                          tunnel: w1443 -> [w1447 _]
                          frame #0 {
                            n826 = Build Array(w1448) -> (w1451:string[])
                            n827 = Build Array(w1450) -> (w1449:dbl[])
                            n828 = TDMS Write(0:w1447, 5:"TEST PASS", 7:w1451, 9:w1449) -> (15:w1453:errorcluster)  [unwired: 2 in, 3 out]
                            n829 = local write "data file error"(w1453) -> ()
                          }
                          frame #1 {
                            n830 = Bundle(cluster=w1456, "STATUS"="CYCLE PASS") -> (w1454:T4)  [unwired: 2 in]
                            n831 = local write "RESULT LAB02-2"(TRUE) -> ()
                            n832 = local write "DISP LAB02-2"(w1454) -> ()
                          }
                        }
                      }
                      frame False {
                      }
                    }
                  }
                }
              }
              frame #4 {
                # "LAB03-1"
                n833 = Less?(x=w1458, y=2) -> (x < y?=w1461:bool)
                n834 = local read "DISP LAB03-1"() -> (w1463:T4)
                n835 = Unbundle(w1463) -> ("STATUS"=w1464:string)  [unwired: 2 out]
                n836 = Equal?(x=w1464, y="RUN") -> (x = y?=w1460:bool)
                n837 = And(x=w1460, y=w1461) -> (x .and. y?=w1459:bool)
                n838 = case shown="True" w1459 {
                  tunnel: w1463 -> [_ w1467]
                  tunnel: w1458 -> [_ w1472]
                  frame False {
                  }
                  frame True {
                    n839 = local read "SET LAB03-1"() -> (w1474:T5)
                    n840 = local read "TDMS LAB03-1"() -> (w1466:refnum<k34>)
                    n841 = Unbundle(w1467) -> ("CYCLE"=w1473:dbl)  [unwired: 2 out]
                    n842 = Unbundle(w1474) -> ("CYCLES"=w1469:dbl, "T-RISE mins"=w1471:dbl)  [unwired: 3 out]
                    n843 = case shown="\"CHART TEST\", Default" w1472 {
                      tunnel: w1471 -> [_ _ w1481]
                      tunnel: [w1476 w1478 w1481] -> w1470
                      tunnel: w1469 -> [w1476 w1478 _]
                      tunnel: ["CHART TEST" "CYCLES" "T-RISE TEST"] -> w1468
                      frame "CHART TEST", Default {
                      }
                      frame "CYCLE TEST" {
                      }
                      frame "T-RISE TEST" {
                      }
                    }
                    n844 = Greater Or Equal?(x=w1473, y=w1469) -> (x >= y?=w1475:bool)
                    n845 = case shown="True" w1475 {
                      tunnel: w1470 -> [w1485 _]
                      tunnel: w1468 -> [w1484 _]
                      tunnel: w1467 -> [w1483 _]
                      tunnel: w1466 -> [w1482 _]
                      frame True {
                        n846 = stacked-sequence {
                          tunnel: w1485 -> [w1489 _]
                          tunnel: w1484 -> [w1487 _]
                          tunnel: w1483 -> [_ w1495]
                          tunnel: w1482 -> [w1486 _]
                          frame #0 {
                            n847 = Build Array(w1487) -> (w1490:string[])
                            n848 = Build Array(w1489) -> (w1488:dbl[])
                            n849 = TDMS Write(0:w1486, 5:"TEST PASS", 7:w1490, 9:w1488) -> (15:w1492:errorcluster)  [unwired: 2 in, 3 out]
                            n850 = local write "data file error"(w1492) -> ()
                          }
                          frame #1 {
                            n851 = Bundle(cluster=w1495, "STATUS"="CYCLE PASS") -> (w1493:T4)  [unwired: 2 in]
                            n852 = local write "RESULT LAB03-1"(TRUE) -> ()
                            n853 = local write "DISP LAB03-1"(w1493) -> ()
                          }
                        }
                      }
                      frame False {
                      }
                    }
                  }
                }
              }
              frame #5 {
                # "LAB03-2"
                n854 = Less?(x=w1497, y=2) -> (x < y?=w1500:bool)
                n855 = local read "DISP LAB03-2"() -> (w1502:T4)
                n856 = Unbundle(w1502) -> ("STATUS"=w1503:string)  [unwired: 2 out]
                n857 = Equal?(x=w1503, y="RUN") -> (x = y?=w1499:bool)
                n858 = And(x=w1499, y=w1500) -> (x .and. y?=w1498:bool)
                n859 = case shown="True" w1498 {
                  tunnel: w1502 -> [_ w1506]
                  tunnel: w1497 -> [_ w1511]
                  frame False {
                  }
                  frame True {
                    n860 = local read "SET LAB03-2"() -> (w1513:T5)
                    n861 = local read "TDMS LAB03-2"() -> (w1505:refnum<k34>)
                    n862 = Unbundle(w1506) -> ("CYCLE"=w1512:dbl)  [unwired: 2 out]
                    n863 = Unbundle(w1513) -> ("CYCLES"=w1508:dbl, "T-RISE mins"=w1510:dbl)  [unwired: 3 out]
                    n864 = case shown="\"CHART TEST\", Default" w1511 {
                      tunnel: w1510 -> [_ _ w1520]
                      tunnel: [w1515 w1517 w1520] -> w1509
                      tunnel: w1508 -> [w1515 w1517 _]
                      tunnel: ["CHART TEST" "CYCLES" "T-RISE TEST"] -> w1507
                      frame "CHART TEST", Default {
                      }
                      frame "CYCLE TEST" {
                      }
                      frame "T-RISE TEST" {
                      }
                    }
                    n865 = Greater Or Equal?(x=w1512, y=w1508) -> (x >= y?=w1514:bool)
                    n866 = case shown="True" w1514 {
                      tunnel: w1509 -> [w1524 _]
                      tunnel: w1507 -> [w1523 _]
                      tunnel: w1506 -> [w1522 _]
                      tunnel: w1505 -> [w1521 _]
                      frame True {
                        n867 = stacked-sequence {
                          tunnel: w1524 -> [w1528 _]
                          tunnel: w1523 -> [w1526 _]
                          tunnel: w1522 -> [_ w1534]
                          tunnel: w1521 -> [w1525 _]
                          frame #0 {
                            n868 = Build Array(w1526) -> (w1529:string[])
                            n869 = Build Array(w1528) -> (w1527:dbl[])
                            n870 = TDMS Write(0:w1525, 5:"TEST PASS", 7:w1529, 9:w1527) -> (15:w1531:errorcluster)  [unwired: 2 in, 3 out]
                            n871 = local write "data file error"(w1531) -> ()
                          }
                          frame #1 {
                            n872 = Bundle(cluster=w1534, "STATUS"="CYCLE PASS") -> (w1532:T4)  [unwired: 2 in]
                            n873 = local write "RESULT LAB03-2"(TRUE) -> ()
                            n874 = local write "DISP LAB03-2"(w1532) -> ()
                          }
                        }
                      }
                      frame False {
                      }
                    }
                  }
                }
              }
              frame #6 {
                # "LAB04-1"
                n875 = Less?(x=w1536, y=2) -> (x < y?=w1539:bool)
                n876 = local read "DISP LAB04-1"() -> (w1541:T4)
                n877 = Unbundle(w1541) -> ("STATUS"=w1542:string)  [unwired: 2 out]
                n878 = Equal?(x=w1542, y="RUN") -> (x = y?=w1538:bool)
                n879 = And(x=w1538, y=w1539) -> (x .and. y?=w1537:bool)
                n880 = case shown="True" w1537 {
                  tunnel: w1541 -> [_ w1545]
                  tunnel: w1536 -> [_ w1550]
                  frame False {
                  }
                  frame True {
                    n881 = local read "SET LAB04-1"() -> (w1552:T5)
                    n882 = local read "TDMS LAB04-1"() -> (w1544:refnum<k34>)
                    n883 = Unbundle(w1545) -> ("CYCLE"=w1551:dbl)  [unwired: 2 out]
                    n884 = Unbundle(w1552) -> ("CYCLES"=w1547:dbl, "T-RISE mins"=w1549:dbl)  [unwired: 3 out]
                    n885 = case shown="\"CHART TEST\", Default" w1550 {
                      tunnel: w1549 -> [_ _ w1559]
                      tunnel: [w1554 w1556 w1559] -> w1548
                      tunnel: w1547 -> [w1554 w1556 _]
                      tunnel: ["CHART TEST" "CYCLES" "T-RISE TEST"] -> w1546
                      frame "CHART TEST", Default {
                      }
                      frame "CYCLE TEST" {
                      }
                      frame "T-RISE TEST" {
                      }
                    }
                    n886 = Greater Or Equal?(x=w1551, y=w1547) -> (x >= y?=w1553:bool)
                    n887 = case shown="True" w1553 {
                      tunnel: w1548 -> [w1563 _]
                      tunnel: w1546 -> [w1562 _]
                      tunnel: w1545 -> [w1561 _]
                      tunnel: w1544 -> [w1560 _]
                      frame True {
                        n888 = stacked-sequence {
                          tunnel: w1563 -> [w1567 _]
                          tunnel: w1562 -> [w1565 _]
                          tunnel: w1561 -> [_ w1573]
                          tunnel: w1560 -> [w1564 _]
                          frame #0 {
                            n889 = Build Array(w1565) -> (w1568:string[])
                            n890 = Build Array(w1567) -> (w1566:dbl[])
                            n891 = TDMS Write(0:w1564, 5:"TEST PASS", 7:w1568, 9:w1566) -> (15:w1570:errorcluster)  [unwired: 2 in, 3 out]
                            n892 = local write "data file error"(w1570) -> ()
                          }
                          frame #1 {
                            n893 = Bundle(cluster=w1573, "STATUS"="CYCLE PASS") -> (w1571:T4)  [unwired: 2 in]
                            n894 = local write "RESULT LAB04-1"(TRUE) -> ()
                            n895 = local write "DISP LAB04-1"(w1571) -> ()
                          }
                        }
                      }
                      frame False {
                      }
                    }
                  }
                }
              }
              frame #7 {
                # "LAB04-2"
                n896 = Less?(x=w1575, y=2) -> (x < y?=w1578:bool)
                n897 = local read "DISP LAB04-2"() -> (w1580:T4)
                n898 = Unbundle(w1580) -> ("STATUS"=w1581:string)  [unwired: 2 out]
                n899 = Equal?(x=w1581, y="RUN") -> (x = y?=w1577:bool)
                n900 = And(x=w1577, y=w1578) -> (x .and. y?=w1576:bool)
                n901 = case shown="True" w1576 {
                  tunnel: w1580 -> [_ w1584]
                  tunnel: w1575 -> [_ w1589]
                  frame False {
                  }
                  frame True {
                    n902 = local read "SET LAB04-2"() -> (w1591:T5)
                    n903 = local read "TDMS LAB04-2"() -> (w1583:refnum<k34>)
                    n904 = Unbundle(w1584) -> ("CYCLE"=w1590:dbl)  [unwired: 2 out]
                    n905 = Unbundle(w1591) -> ("CYCLES"=w1586:dbl, "T-RISE mins"=w1588:dbl)  [unwired: 3 out]
                    n906 = case shown="\"CHART TEST\", Default" w1589 {
                      tunnel: w1588 -> [_ _ w1598]
                      tunnel: [w1593 w1595 w1598] -> w1587
                      tunnel: w1586 -> [w1593 w1595 _]
                      tunnel: ["CHART TEST" "CYCLES" "T-RISE TEST"] -> w1585
                      frame "CHART TEST", Default {
                      }
                      frame "CYCLE TEST" {
                      }
                      frame "T-RISE TEST" {
                      }
                    }
                    n907 = Greater Or Equal?(x=w1590, y=w1586) -> (x >= y?=w1592:bool)
                    n908 = case shown="True" w1592 {
                      tunnel: w1587 -> [w1602 _]
                      tunnel: w1585 -> [w1601 _]
                      tunnel: w1584 -> [w1600 _]
                      tunnel: w1583 -> [w1599 _]
                      frame True {
                        n909 = stacked-sequence {
                          tunnel: w1602 -> [w1606 _]
                          tunnel: w1601 -> [w1604 _]
                          tunnel: w1600 -> [_ w1612]
                          tunnel: w1599 -> [w1603 _]
                          frame #0 {
                            n910 = Build Array(w1604) -> (w1607:string[])
                            n911 = Build Array(w1606) -> (w1605:dbl[])
                            n912 = TDMS Write(0:w1603, 5:"TEST PASS", 7:w1607, 9:w1605) -> (15:w1609:errorcluster)  [unwired: 2 in, 3 out]
                            n913 = local write "data file error"(w1609) -> ()
                          }
                          frame #1 {
                            n914 = Bundle(cluster=w1612, "STATUS"="CYCLE PASS") -> (w1610:T4)  [unwired: 2 in]
                            n915 = local write "RESULT LAB04-2"(TRUE) -> ()
                            n916 = local write "DISP LAB04-2"(w1610) -> ()
                          }
                        }
                      }
                      frame False {
                      }
                    }
                  }
                }
              }
              frame #8 {
                # "LAB05-1"
                n917 = Less?(x=w1614, y=2) -> (x < y?=w1617:bool)
                n918 = local read "DISP LAB05-1"() -> (w1619:T4)
                n919 = Unbundle(w1619) -> ("STATUS"=w1620:string)  [unwired: 2 out]
                n920 = Equal?(x=w1620, y="RUN") -> (x = y?=w1616:bool)
                n921 = And(x=w1616, y=w1617) -> (x .and. y?=w1615:bool)
                n922 = case shown="True" w1615 {
                  tunnel: w1619 -> [_ w1623]
                  tunnel: w1614 -> [_ w1628]
                  frame False {
                  }
                  frame True {
                    n923 = local read "SET LAB05-1"() -> (w1630:T5)
                    n924 = local read "TDMS LAB05-1"() -> (w1622:refnum<k34>)
                    n925 = Unbundle(w1623) -> ("CYCLE"=w1629:dbl)  [unwired: 2 out]
                    n926 = Unbundle(w1630) -> ("CYCLES"=w1625:dbl, "T-RISE mins"=w1627:dbl)  [unwired: 3 out]
                    n927 = case shown="\"CHART TEST\", Default" w1628 {
                      tunnel: w1627 -> [_ _ w1637]
                      tunnel: [w1632 w1634 w1637] -> w1626
                      tunnel: w1625 -> [w1632 w1634 _]
                      tunnel: ["CHART TEST" "CYCLES" "T-RISE TEST"] -> w1624
                      frame "CHART TEST", Default {
                      }
                      frame "CYCLE TEST" {
                      }
                      frame "T-RISE TEST" {
                      }
                    }
                    n928 = Greater Or Equal?(x=w1629, y=w1625) -> (x >= y?=w1631:bool)
                    n929 = case shown="True" w1631 {
                      tunnel: w1626 -> [w1641 _]
                      tunnel: w1624 -> [w1640 _]
                      tunnel: w1623 -> [w1639 _]
                      tunnel: w1622 -> [w1638 _]
                      frame True {
                        n930 = stacked-sequence {
                          tunnel: w1641 -> [w1645 _]
                          tunnel: w1640 -> [w1643 _]
                          tunnel: w1639 -> [_ w1651]
                          tunnel: w1638 -> [w1642 _]
                          frame #0 {
                            n931 = Build Array(w1643) -> (w1646:string[])
                            n932 = Build Array(w1645) -> (w1644:dbl[])
                            n933 = TDMS Write(0:w1642, 5:"TEST PASS", 7:w1646, 9:w1644) -> (15:w1648:errorcluster)  [unwired: 2 in, 3 out]
                            n934 = local write "data file error"(w1648) -> ()
                          }
                          frame #1 {
                            n935 = Bundle(cluster=w1651, "STATUS"="CYCLE PASS") -> (w1649:T4)  [unwired: 2 in]
                            n936 = local write "RESULT LAB05-1"(TRUE) -> ()
                            n937 = local write "DISP LAB05-1"(w1649) -> ()
                          }
                        }
                      }
                      frame False {
                      }
                    }
                  }
                }
              }
              frame #9 {
                # "LAB05-2"
                n938 = Less?(x=w1653, y=2) -> (x < y?=w1656:bool)
                n939 = local read "DISP LAB05-2"() -> (w1658:T4)
                n940 = Unbundle(w1658) -> ("STATUS"=w1659:string)  [unwired: 2 out]
                n941 = Equal?(x=w1659, y="RUN") -> (x = y?=w1655:bool)
                n942 = And(x=w1655, y=w1656) -> (x .and. y?=w1654:bool)
                n943 = case shown="True" w1654 {
                  tunnel: w1658 -> [_ w1662]
                  tunnel: w1653 -> [_ w1667]
                  frame False {
                  }
                  frame True {
                    n944 = local read "SET LAB05-2"() -> (w1669:T5)
                    n945 = local read "TDMS LAB05-2"() -> (w1661:refnum<k34>)
                    n946 = Unbundle(w1662) -> ("CYCLE"=w1668:dbl)  [unwired: 2 out]
                    n947 = Unbundle(w1669) -> ("CYCLES"=w1664:dbl, "T-RISE mins"=w1666:dbl)  [unwired: 3 out]
                    n948 = case shown="\"CHART TEST\", Default" w1667 {
                      tunnel: w1666 -> [_ _ w1676]
                      tunnel: [w1671 w1673 w1676] -> w1665
                      tunnel: w1664 -> [w1671 w1673 _]
                      tunnel: ["CHART TEST" "CYCLES" "T-RISE TEST"] -> w1663
                      frame "CHART TEST", Default {
                      }
                      frame "CYCLE TEST" {
                      }
                      frame "T-RISE TEST" {
                      }
                    }
                    n949 = Greater Or Equal?(x=w1668, y=w1664) -> (x >= y?=w1670:bool)
                    n950 = case shown="True" w1670 {
                      tunnel: w1665 -> [w1680 _]
                      tunnel: w1663 -> [w1679 _]
                      tunnel: w1662 -> [w1678 _]
                      tunnel: w1661 -> [w1677 _]
                      frame True {
                        n951 = stacked-sequence {
                          tunnel: w1680 -> [w1684 _]
                          tunnel: w1679 -> [w1682 _]
                          tunnel: w1678 -> [_ w1690]
                          tunnel: w1677 -> [w1681 _]
                          frame #0 {
                            n952 = Build Array(w1682) -> (w1685:string[])
                            n953 = Build Array(w1684) -> (w1683:dbl[])
                            n954 = TDMS Write(0:w1681, 5:"TEST PASS", 7:w1685, 9:w1683) -> (15:w1687:errorcluster)  [unwired: 2 in, 3 out]
                            n955 = local write "data file error"(w1687) -> ()
                          }
                          frame #1 {
                            n956 = Bundle(cluster=w1690, "STATUS"="CYCLE PASS") -> (w1688:T4)  [unwired: 2 in]
                            n957 = local write "RESULT LAB05-2"(TRUE) -> ()
                            n958 = local write "DISP LAB05-2"(w1688) -> ()
                          }
                        }
                      }
                      frame False {
                      }
                    }
                  }
                }
              }
            }
          }
          frame #5 {
            # "check if test cycles reached for temperature rise test"
            n959 = stacked-sequence {
              tunnel: w1721 -> [_ _ _ _ _ _ _ _ _ _]
              tunnel: w1720 -> [_ _ _ _ _ _ _ _ _ _]
              tunnel: w1719 -> [_ _ _ _ _ _ _ _ _ _]
              tunnel: w1718 -> [_ _ _ _ _ _ _ _ _ _]
              tunnel: w1717 -> [_ _ _ _ _ _ _ _ _ _]
              tunnel: w1716 -> [_ _ _ _ _ _ _ _ _ _]
              tunnel: w1715 -> [_ _ _ _ _ _ _ _ _ _]
              tunnel: w1714 -> [_ _ _ _ _ _ _ _ _ _]
              tunnel: w1713 -> [_ _ _ _ _ _ _ _ _ _]
              tunnel: w1712 -> [_ _ _ _ _ _ _ _ _ _]
              tunnel: w1711 -> [w1727 _ _ _ _ _ _ _ _ _]
              tunnel: w1701 -> [w1722 _ _ _ _ _ _ _ _ _]
              tunnel: w1710 -> [_ w1753 _ _ _ _ _ _ _ _]
              tunnel: w1709 -> [_ _ w1783 _ _ _ _ _ _ _]
              tunnel: w1708 -> [_ _ _ w1813 _ _ _ _ _ _]
              tunnel: w1707 -> [_ _ _ _ w1843 _ _ _ _ _]
              tunnel: w1706 -> [_ _ _ _ _ w1873 _ _ _ _]
              tunnel: w1705 -> [_ _ _ _ _ _ w1903 _ _ _]
              tunnel: w1704 -> [_ _ _ _ _ _ _ w1933 _ _]
              tunnel: w1703 -> [_ _ _ _ _ _ _ _ w1963 _]
              tunnel: w1702 -> [_ _ _ _ _ _ _ _ _ w1993]
              tunnel: w1700 -> [_ w1752 _ _ _ _ _ _ _ _]
              tunnel: w1699 -> [_ _ w1782 _ _ _ _ _ _ _]
              tunnel: w1698 -> [_ _ _ w1812 _ _ _ _ _ _]
              tunnel: w1697 -> [_ _ _ _ w1842 _ _ _ _ _]
              tunnel: w1696 -> [_ _ _ _ _ w1872 _ _ _ _]
              tunnel: w1695 -> [_ _ _ _ _ _ w1902 _ _ _]
              tunnel: w1694 -> [_ _ _ _ _ _ _ w1932 _ _]
              tunnel: w1693 -> [_ _ _ _ _ _ _ _ w1962 _]
              tunnel: w1692 -> [_ _ _ _ _ _ _ _ _ w1992]
              frame #0 {
                # "LAB01-1"
                n960 = Equal?(x=w1727, y=2) -> (x = y?=w1725:bool)
                n961 = local read "DISP LAB01-1"() -> (w1728:T4)
                n962 = Unbundle(w1728) -> ("STATUS"=w1729:string)  [unwired: 2 out]
                n963 = Equal?(x=w1729, y="RUN") -> (x = y?=w1724:bool)
                n964 = And(x=w1724, y=w1725) -> (x .and. y?=w1723:bool)
                n965 = case shown="True" w1723 {
                  tunnel: w1728 -> [_ w1732]
                  tunnel: w1722 -> [_ w1735]
                  frame False {
                  }
                  frame True {
                    n966 = local read "SET LAB01-1"() -> (w1734:T5)
                    n967 = local read "TDMS LAB01-1"() -> (w1731:refnum<k34>)
                    n968 = Unbundle(w1732) -> ("CYCLE"=w1736:dbl)  [unwired: 2 out]
                    n969 = Unbundle(w1734) -> ("T-RISE mins"=w1733:dbl)  [unwired: 4 out]
                    n970 = Greater Or Equal?(x=w1736, y=w1735) -> (x >= y?=w1737:bool)
                    n971 = case shown="True" w1737 {
                      tunnel: w1733 -> [w1740 _]
                      tunnel: w1732 -> [w1739 _]
                      tunnel: w1731 -> [w1738 _]
                      frame True {
                        n972 = stacked-sequence {
                          tunnel: w1740 -> [w1743 _]
                          tunnel: w1739 -> [_ w1748]
                          tunnel: w1738 -> [w1741 _]
                          frame #0 {
                            n973 = Build Array("T-RISE") -> (w1745:string[])
                            n974 = Build Array(w1743) -> (w1744:dbl[])
                            n975 = TDMS Write(0:w1741, 5:"TEST PASS", 7:w1745, 9:w1744) -> (15:w1747:errorcluster)  [unwired: 2 in, 3 out]
                            n976 = local write "data file error"(w1747) -> ()
                          }
                          frame #1 {
                            n977 = Bundle(cluster=w1748, "STATUS"="T-RISE PASS") -> (w1750:T4)  [unwired: 2 in]
                            n978 = local write "RESULT LAB01-1"(TRUE) -> ()
                            n979 = local write "DISP LAB01-1"(w1750) -> ()
                          }
                        }
                      }
                      frame False {
                      }
                    }
                  }
                }
              }
              frame #1 {
                # "LAB01-2"
                n980 = Equal?(x=w1753, y=2) -> (x = y?=w1756:bool)
                n981 = local read "DISP LAB01-2"() -> (w1758:T4)
                n982 = Unbundle(w1758) -> ("STATUS"=w1759:string)  [unwired: 2 out]
                n983 = Equal?(x=w1759, y="RUN") -> (x = y?=w1755:bool)
                n984 = And(x=w1755, y=w1756) -> (x .and. y?=w1754:bool)
                n985 = case shown="True" w1754 {
                  tunnel: w1758 -> [_ w1762]
                  tunnel: w1752 -> [_ w1765]
                  frame False {
                  }
                  frame True {
                    n986 = local read "SET LAB01-2"() -> (w1764:T5)
                    n987 = local read "TDMS LAB01-2"() -> (w1761:refnum<k34>)
                    n988 = Unbundle(w1762) -> ("CYCLE"=w1766:dbl)  [unwired: 2 out]
                    n989 = Unbundle(w1764) -> ("T-RISE mins"=w1763:dbl)  [unwired: 4 out]
                    n990 = Greater Or Equal?(x=w1766, y=w1765) -> (x >= y?=w1767:bool)
                    n991 = case shown="True" w1767 {
                      tunnel: w1763 -> [w1770 _]
                      tunnel: w1762 -> [w1769 _]
                      tunnel: w1761 -> [w1768 _]
                      frame True {
                        n992 = stacked-sequence {
                          tunnel: w1770 -> [w1773 _]
                          tunnel: w1769 -> [_ w1778]
                          tunnel: w1768 -> [w1771 _]
                          frame #0 {
                            n993 = Build Array("T-RISE") -> (w1775:string[])
                            n994 = Build Array(w1773) -> (w1774:dbl[])
                            n995 = TDMS Write(0:w1771, 5:"TEST PASS", 7:w1775, 9:w1774) -> (15:w1777:errorcluster)  [unwired: 2 in, 3 out]
                            n996 = local write "data file error"(w1777) -> ()
                          }
                          frame #1 {
                            n997 = Bundle(cluster=w1778, "STATUS"="T-RISE PASS") -> (w1780:T4)  [unwired: 2 in]
                            n998 = local write "RESULT LAB01-2"(TRUE) -> ()
                            n999 = local write "DISP LAB01-2"(w1780) -> ()
                          }
                        }
                      }
                      frame False {
                      }
                    }
                  }
                }
              }
              frame #2 {
                # "LAB02-1"
                n1000 = Equal?(x=w1783, y=2) -> (x = y?=w1786:bool)
                n1001 = local read "DISP LAB02-1"() -> (w1788:T4)
                n1002 = Unbundle(w1788) -> ("STATUS"=w1789:string)  [unwired: 2 out]
                n1003 = Equal?(x=w1789, y="RUN") -> (x = y?=w1785:bool)
                n1004 = And(x=w1785, y=w1786) -> (x .and. y?=w1784:bool)
                n1005 = case shown="True" w1784 {
                  tunnel: w1788 -> [_ w1792]
                  tunnel: w1782 -> [_ w1795]
                  frame False {
                  }
                  frame True {
                    n1006 = local read "SET LAB02-1"() -> (w1794:T5)
                    n1007 = local read "TDMS LAB02-1"() -> (w1791:refnum<k34>)
                    n1008 = Unbundle(w1792) -> ("CYCLE"=w1796:dbl)  [unwired: 2 out]
                    n1009 = Unbundle(w1794) -> ("T-RISE mins"=w1793:dbl)  [unwired: 4 out]
                    n1010 = Greater Or Equal?(x=w1796, y=w1795) -> (x >= y?=w1797:bool)
                    n1011 = case shown="True" w1797 {
                      tunnel: w1793 -> [w1800 _]
                      tunnel: w1792 -> [w1799 _]
                      tunnel: w1791 -> [w1798 _]
                      frame True {
                        n1012 = stacked-sequence {
                          tunnel: w1800 -> [w1803 _]
                          tunnel: w1799 -> [_ w1808]
                          tunnel: w1798 -> [w1801 _]
                          frame #0 {
                            n1013 = Build Array("T-RISE") -> (w1805:string[])
                            n1014 = Build Array(w1803) -> (w1804:dbl[])
                            n1015 = TDMS Write(0:w1801, 5:"TEST PASS", 7:w1805, 9:w1804) -> (15:w1807:errorcluster)  [unwired: 2 in, 3 out]
                            n1016 = local write "data file error"(w1807) -> ()
                          }
                          frame #1 {
                            n1017 = Bundle(cluster=w1808, "STATUS"="T-RISE PASS") -> (w1810:T4)  [unwired: 2 in]
                            n1018 = local write "RESULT LAB02-1"(TRUE) -> ()
                            n1019 = local write "DISP LAB02-1"(w1810) -> ()
                          }
                        }
                      }
                      frame False {
                      }
                    }
                  }
                }
              }
              frame #3 {
                # "LAB02-2"
                n1020 = Equal?(x=w1813, y=2) -> (x = y?=w1816:bool)
                n1021 = local read "DISP LAB02-2"() -> (w1818:T4)
                n1022 = Unbundle(w1818) -> ("STATUS"=w1819:string)  [unwired: 2 out]
                n1023 = Equal?(x=w1819, y="RUN") -> (x = y?=w1815:bool)
                n1024 = And(x=w1815, y=w1816) -> (x .and. y?=w1814:bool)
                n1025 = case shown="True" w1814 {
                  tunnel: w1818 -> [_ w1822]
                  tunnel: w1812 -> [_ w1825]
                  frame False {
                  }
                  frame True {
                    n1026 = local read "SET LAB02-2"() -> (w1824:T5)
                    n1027 = local read "TDMS LAB02-2"() -> (w1821:refnum<k34>)
                    n1028 = Unbundle(w1822) -> ("CYCLE"=w1826:dbl)  [unwired: 2 out]
                    n1029 = Unbundle(w1824) -> ("T-RISE mins"=w1823:dbl)  [unwired: 4 out]
                    n1030 = Greater Or Equal?(x=w1826, y=w1825) -> (x >= y?=w1827:bool)
                    n1031 = case shown="True" w1827 {
                      tunnel: w1823 -> [w1830 _]
                      tunnel: w1822 -> [w1829 _]
                      tunnel: w1821 -> [w1828 _]
                      frame True {
                        n1032 = stacked-sequence {
                          tunnel: w1830 -> [w1833 _]
                          tunnel: w1829 -> [_ w1838]
                          tunnel: w1828 -> [w1831 _]
                          frame #0 {
                            n1033 = Build Array("T-RISE") -> (w1835:string[])
                            n1034 = Build Array(w1833) -> (w1834:dbl[])
                            n1035 = TDMS Write(0:w1831, 5:"TEST PASS", 7:w1835, 9:w1834) -> (15:w1837:errorcluster)  [unwired: 2 in, 3 out]
                            n1036 = local write "data file error"(w1837) -> ()
                          }
                          frame #1 {
                            n1037 = Bundle(cluster=w1838, "STATUS"="T-RISE PASS") -> (w1840:T4)  [unwired: 2 in]
                            n1038 = local write "RESULT LAB02-2"(TRUE) -> ()
                            n1039 = local write "DISP LAB02-2"(w1840) -> ()
                          }
                        }
                      }
                      frame False {
                      }
                    }
                  }
                }
              }
              frame #4 {
                # "LAB03-1"
                n1040 = Equal?(x=w1843, y=2) -> (x = y?=w1846:bool)
                n1041 = local read "DISP LAB03-1"() -> (w1848:T4)
                n1042 = Unbundle(w1848) -> ("STATUS"=w1849:string)  [unwired: 2 out]
                n1043 = Equal?(x=w1849, y="RUN") -> (x = y?=w1845:bool)
                n1044 = And(x=w1845, y=w1846) -> (x .and. y?=w1844:bool)
                n1045 = case shown="True" w1844 {
                  tunnel: w1848 -> [_ w1852]
                  tunnel: w1842 -> [_ w1855]
                  frame False {
                  }
                  frame True {
                    n1046 = local read "SET LAB03-1"() -> (w1854:T5)
                    n1047 = local read "TDMS LAB03-1"() -> (w1851:refnum<k34>)
                    n1048 = Unbundle(w1852) -> ("CYCLE"=w1856:dbl)  [unwired: 2 out]
                    n1049 = Unbundle(w1854) -> ("T-RISE mins"=w1853:dbl)  [unwired: 4 out]
                    n1050 = Greater Or Equal?(x=w1856, y=w1855) -> (x >= y?=w1857:bool)
                    n1051 = case shown="True" w1857 {
                      tunnel: w1853 -> [w1860 _]
                      tunnel: w1852 -> [w1859 _]
                      tunnel: w1851 -> [w1858 _]
                      frame True {
                        n1052 = stacked-sequence {
                          tunnel: w1860 -> [w1863 _]
                          tunnel: w1859 -> [_ w1868]
                          tunnel: w1858 -> [w1861 _]
                          frame #0 {
                            n1053 = Build Array("T-RISE") -> (w1865:string[])
                            n1054 = Build Array(w1863) -> (w1864:dbl[])
                            n1055 = TDMS Write(0:w1861, 5:"TEST PASS", 7:w1865, 9:w1864) -> (15:w1867:errorcluster)  [unwired: 2 in, 3 out]
                            n1056 = local write "data file error"(w1867) -> ()
                          }
                          frame #1 {
                            n1057 = Bundle(cluster=w1868, "STATUS"="T-RISE PASS") -> (w1870:T4)  [unwired: 2 in]
                            n1058 = local write "RESULT LAB03-1"(TRUE) -> ()
                            n1059 = local write "DISP LAB03-1"(w1870) -> ()
                          }
                        }
                      }
                      frame False {
                      }
                    }
                  }
                }
              }
              frame #5 {
                # "LAB03-2"
                n1060 = Equal?(x=w1873, y=2) -> (x = y?=w1876:bool)
                n1061 = local read "DISP LAB03-2"() -> (w1878:T4)
                n1062 = Unbundle(w1878) -> ("STATUS"=w1879:string)  [unwired: 2 out]
                n1063 = Equal?(x=w1879, y="RUN") -> (x = y?=w1875:bool)
                n1064 = And(x=w1875, y=w1876) -> (x .and. y?=w1874:bool)
                n1065 = case shown="True" w1874 {
                  tunnel: w1878 -> [_ w1882]
                  tunnel: w1872 -> [_ w1885]
                  frame False {
                  }
                  frame True {
                    n1066 = local read "SET LAB03-2"() -> (w1884:T5)
                    n1067 = local read "TDMS LAB03-2"() -> (w1881:refnum<k34>)
                    n1068 = Unbundle(w1882) -> ("CYCLE"=w1886:dbl)  [unwired: 2 out]
                    n1069 = Unbundle(w1884) -> ("T-RISE mins"=w1883:dbl)  [unwired: 4 out]
                    n1070 = Greater Or Equal?(x=w1886, y=w1885) -> (x >= y?=w1887:bool)
                    n1071 = case shown="True" w1887 {
                      tunnel: w1883 -> [w1890 _]
                      tunnel: w1882 -> [w1889 _]
                      tunnel: w1881 -> [w1888 _]
                      frame True {
                        n1072 = stacked-sequence {
                          tunnel: w1890 -> [w1893 _]
                          tunnel: w1889 -> [_ w1898]
                          tunnel: w1888 -> [w1891 _]
                          frame #0 {
                            n1073 = Build Array("T-RISE") -> (w1895:string[])
                            n1074 = Build Array(w1893) -> (w1894:dbl[])
                            n1075 = TDMS Write(0:w1891, 5:"TEST PASS", 7:w1895, 9:w1894) -> (15:w1897:errorcluster)  [unwired: 2 in, 3 out]
                            n1076 = local write "data file error"(w1897) -> ()
                          }
                          frame #1 {
                            n1077 = Bundle(cluster=w1898, "STATUS"="T-RISE PASS") -> (w1900:T4)  [unwired: 2 in]
                            n1078 = local write "RESULT LAB03-2"(TRUE) -> ()
                            n1079 = local write "DISP LAB03-2"(w1900) -> ()
                          }
                        }
                      }
                      frame False {
                      }
                    }
                  }
                }
              }
              frame #6 {
                # "LAB04-1"
                n1080 = Equal?(x=w1903, y=2) -> (x = y?=w1906:bool)
                n1081 = local read "DISP LAB04-1"() -> (w1908:T4)
                n1082 = Unbundle(w1908) -> ("STATUS"=w1909:string)  [unwired: 2 out]
                n1083 = Equal?(x=w1909, y="RUN") -> (x = y?=w1905:bool)
                n1084 = And(x=w1905, y=w1906) -> (x .and. y?=w1904:bool)
                n1085 = case shown="True" w1904 {
                  tunnel: w1908 -> [_ w1912]
                  tunnel: w1902 -> [_ w1915]
                  frame False {
                  }
                  frame True {
                    n1086 = local read "SET LAB04-1"() -> (w1914:T5)
                    n1087 = local read "TDMS LAB04-1"() -> (w1911:refnum<k34>)
                    n1088 = Unbundle(w1912) -> ("CYCLE"=w1916:dbl)  [unwired: 2 out]
                    n1089 = Unbundle(w1914) -> ("T-RISE mins"=w1913:dbl)  [unwired: 4 out]
                    n1090 = Greater Or Equal?(x=w1916, y=w1915) -> (x >= y?=w1917:bool)
                    n1091 = case shown="True" w1917 {
                      tunnel: w1913 -> [w1920 _]
                      tunnel: w1912 -> [w1919 _]
                      tunnel: w1911 -> [w1918 _]
                      frame True {
                        n1092 = stacked-sequence {
                          tunnel: w1920 -> [w1923 _]
                          tunnel: w1919 -> [_ w1928]
                          tunnel: w1918 -> [w1921 _]
                          frame #0 {
                            n1093 = Build Array("T-RISE") -> (w1925:string[])
                            n1094 = Build Array(w1923) -> (w1924:dbl[])
                            n1095 = TDMS Write(0:w1921, 5:"TEST PASS", 7:w1925, 9:w1924) -> (15:w1927:errorcluster)  [unwired: 2 in, 3 out]
                            n1096 = local write "data file error"(w1927) -> ()
                          }
                          frame #1 {
                            n1097 = Bundle(cluster=w1928, "STATUS"="T-RISE PASS") -> (w1930:T4)  [unwired: 2 in]
                            n1098 = local write "RESULT LAB04-1"(TRUE) -> ()
                            n1099 = local write "DISP LAB04-1"(w1930) -> ()
                          }
                        }
                      }
                      frame False {
                      }
                    }
                  }
                }
              }
              frame #7 {
                # "LAB04-2"
                n1100 = Equal?(x=w1933, y=2) -> (x = y?=w1936:bool)
                n1101 = local read "DISP LAB04-2"() -> (w1938:T4)
                n1102 = Unbundle(w1938) -> ("STATUS"=w1939:string)  [unwired: 2 out]
                n1103 = Equal?(x=w1939, y="RUN") -> (x = y?=w1935:bool)
                n1104 = And(x=w1935, y=w1936) -> (x .and. y?=w1934:bool)
                n1105 = case shown="True" w1934 {
                  tunnel: w1938 -> [_ w1942]
                  tunnel: w1932 -> [_ w1945]
                  frame False {
                  }
                  frame True {
                    n1106 = local read "SET LAB04-2"() -> (w1944:T5)
                    n1107 = local read "TDMS LAB04-2"() -> (w1941:refnum<k34>)
                    n1108 = Unbundle(w1942) -> ("CYCLE"=w1946:dbl)  [unwired: 2 out]
                    n1109 = Unbundle(w1944) -> ("T-RISE mins"=w1943:dbl)  [unwired: 4 out]
                    n1110 = Greater Or Equal?(x=w1946, y=w1945) -> (x >= y?=w1947:bool)
                    n1111 = case shown="True" w1947 {
                      tunnel: w1943 -> [w1950 _]
                      tunnel: w1942 -> [w1949 _]
                      tunnel: w1941 -> [w1948 _]
                      frame True {
                        n1112 = stacked-sequence {
                          tunnel: w1950 -> [w1953 _]
                          tunnel: w1949 -> [_ w1958]
                          tunnel: w1948 -> [w1951 _]
                          frame #0 {
                            n1113 = Build Array("T-RISE") -> (w1955:string[])
                            n1114 = Build Array(w1953) -> (w1954:dbl[])
                            n1115 = TDMS Write(0:w1951, 5:"TEST PASS", 7:w1955, 9:w1954) -> (15:w1957:errorcluster)  [unwired: 2 in, 3 out]
                            n1116 = local write "data file error"(w1957) -> ()
                          }
                          frame #1 {
                            n1117 = Bundle(cluster=w1958, "STATUS"="T-RISE PASS") -> (w1960:T4)  [unwired: 2 in]
                            n1118 = local write "RESULT LAB04-2"(TRUE) -> ()
                            n1119 = local write "DISP LAB04-2"(w1960) -> ()
                          }
                        }
                      }
                      frame False {
                      }
                    }
                  }
                }
              }
              frame #8 {
                # "LAB05-1"
                n1120 = Equal?(x=w1963, y=2) -> (x = y?=w1966:bool)
                n1121 = local read "DISP LAB05-1"() -> (w1968:T4)
                n1122 = Unbundle(w1968) -> ("STATUS"=w1969:string)  [unwired: 2 out]
                n1123 = Equal?(x=w1969, y="RUN") -> (x = y?=w1965:bool)
                n1124 = And(x=w1965, y=w1966) -> (x .and. y?=w1964:bool)
                n1125 = case shown="True" w1964 {
                  tunnel: w1968 -> [_ w1972]
                  tunnel: w1962 -> [_ w1975]
                  frame False {
                  }
                  frame True {
                    n1126 = local read "SET LAB05-1"() -> (w1974:T5)
                    n1127 = local read "TDMS LAB05-1"() -> (w1971:refnum<k34>)
                    n1128 = Unbundle(w1972) -> ("CYCLE"=w1976:dbl)  [unwired: 2 out]
                    n1129 = Unbundle(w1974) -> ("T-RISE mins"=w1973:dbl)  [unwired: 4 out]
                    n1130 = Greater Or Equal?(x=w1976, y=w1975) -> (x >= y?=w1977:bool)
                    n1131 = case shown="True" w1977 {
                      tunnel: w1973 -> [w1980 _]
                      tunnel: w1972 -> [w1979 _]
                      tunnel: w1971 -> [w1978 _]
                      frame True {
                        n1132 = stacked-sequence {
                          tunnel: w1980 -> [w1983 _]
                          tunnel: w1979 -> [_ w1988]
                          tunnel: w1978 -> [w1981 _]
                          frame #0 {
                            n1133 = Build Array("T-RISE") -> (w1985:string[])
                            n1134 = Build Array(w1983) -> (w1984:dbl[])
                            n1135 = TDMS Write(0:w1981, 5:"TEST PASS", 7:w1985, 9:w1984) -> (15:w1987:errorcluster)  [unwired: 2 in, 3 out]
                            n1136 = local write "data file error"(w1987) -> ()
                          }
                          frame #1 {
                            n1137 = Bundle(cluster=w1988, "STATUS"="T-RISE PASS") -> (w1990:T4)  [unwired: 2 in]
                            n1138 = local write "RESULT LAB05-1"(TRUE) -> ()
                            n1139 = local write "DISP LAB05-1"(w1990) -> ()
                          }
                        }
                      }
                      frame False {
                      }
                    }
                  }
                }
              }
              frame #9 {
                # "LAB05-2"
                n1140 = Equal?(x=w1993, y=2) -> (x = y?=w1996:bool)
                n1141 = local read "DISP LAB05-2"() -> (w1998:T4)
                n1142 = Unbundle(w1998) -> ("STATUS"=w1999:string)  [unwired: 2 out]
                n1143 = Equal?(x=w1999, y="RUN") -> (x = y?=w1995:bool)
                n1144 = And(x=w1995, y=w1996) -> (x .and. y?=w1994:bool)
                n1145 = case shown="True" w1994 {
                  tunnel: w1998 -> [_ w2002]
                  tunnel: w1992 -> [_ w2005]
                  frame False {
                  }
                  frame True {
                    n1146 = local read "SET LAB05-2"() -> (w2004:T5)
                    n1147 = local read "TDMS LAB05-2"() -> (w2001:refnum<k34>)
                    n1148 = Unbundle(w2002) -> ("CYCLE"=w2006:dbl)  [unwired: 2 out]
                    n1149 = Unbundle(w2004) -> ("T-RISE mins"=w2003:dbl)  [unwired: 4 out]
                    n1150 = Greater Or Equal?(x=w2006, y=w2005) -> (x >= y?=w2007:bool)
                    n1151 = case shown="True" w2007 {
                      tunnel: w2003 -> [w2010 _]
                      tunnel: w2002 -> [w2009 _]
                      tunnel: w2001 -> [w2008 _]
                      frame True {
                        n1152 = stacked-sequence {
                          tunnel: w2010 -> [w2013 _]
                          tunnel: w2009 -> [_ w2018]
                          tunnel: w2008 -> [w2011 _]
                          frame #0 {
                            n1153 = Build Array("T-RISE") -> (w2015:string[])
                            n1154 = Build Array(w2013) -> (w2014:dbl[])
                            n1155 = TDMS Write(0:w2011, 5:"TEST PASS", 7:w2015, 9:w2014) -> (15:w2017:errorcluster)  [unwired: 2 in, 3 out]
                            n1156 = local write "data file error"(w2017) -> ()
                          }
                          frame #1 {
                            n1157 = Bundle(cluster=w2018, "STATUS"="T-RISE PASS") -> (w2020:T4)  [unwired: 2 in]
                            n1158 = local write "RESULT LAB05-2"(TRUE) -> ()
                            n1159 = local write "DISP LAB05-2"(w2020) -> ()
                          }
                        }
                      }
                      frame False {
                      }
                    }
                  }
                }
              }
            }
          }
          frame #6 {
            # "disable functions"
            n1160 = stacked-sequence {
              tunnel: w2031 -> [w2045 _ w2101]
              tunnel: w2030 -> [w2040 _ w2100]
              tunnel: w2029 -> [w2039 _ w2099]
              tunnel: w2028 -> [w2037 _ w2098]
              tunnel: w2027 -> [w2038 _ w2097]
              tunnel: w2026 -> [_ w2062 w2096]
              tunnel: w2025 -> [_ w2063 w2095]
              tunnel: w2024 -> [_ w2064 w2094]
              tunnel: w2023 -> [_ w2065 w2093]
              tunnel: w2022 -> [_ w2066 w2092]
              frame #0 {
                n1161 = Select(t=2, s=w2037, f=0) -> (s? t:f=w2033:i32)
                n1162 = Select(t=2, s=w2039, f=0) -> (s? t:f=w2034:i32)
                n1163 = Select(t=2, s=w2038, f=0) -> (s? t:f=w2032:i32)
                n1164 = Select(t=2, s=w2045, f=0) -> (s? t:f=w2036:i32)
                n1165 = Select(t=2, s=w2040, f=0) -> (s? t:f=w2035:i32)
                n1166 = property on="SELECT LAB02-2" class="RadioBtnsControl (strict)"("DisabledEnum"=w2033) -> ()  [unwired: 2 in, 2 out]
                n1167 = property on="SELECT LAB02-1" class="RadioBtnsControl (strict)"("DisabledEnum"=w2034) -> ()  [unwired: 2 in, 2 out]
                n1168 = property on="SELECT LAB03-1" class="RadioBtnsControl (strict)"("DisabledEnum"=w2032) -> ()  [unwired: 2 in, 2 out]
                n1169 = property on="SELECT LAB01-1" class="RadioBtnsControl (strict)"("DisabledEnum"=w2036) -> ()  [unwired: 2 in, 2 out]
                n1170 = property on="SELECT LAB01-2" class="RadioBtnsControl (strict)"("DisabledEnum"=w2035) -> ()  [unwired: 2 in, 2 out]
                n1171 = Not(x=w2045) -> (.not. x?=w2046:bool)
                n1172 = property on="RESULT LAB01-1" class="Bool (strict)"("Visible"=w2046) -> ()  [unwired: 2 in, 2 out]
                n1173 = Not(x=w2040) -> (.not. x?=w2044:bool)
                n1174 = Not(x=w2039) -> (.not. x?=w2043:bool)
                n1175 = Not(x=w2037) -> (.not. x?=w2042:bool)
                n1176 = property on="RESULT LAB01-2" class="Bool (strict)"("Visible"=w2044) -> ()  [unwired: 2 in, 2 out]
                n1177 = Not(x=w2038) -> (.not. x?=w2041:bool)
                n1178 = property on="RESULT LAB02-1" class="Bool (strict)"("Visible"=w2043) -> ()  [unwired: 2 in, 2 out]
                n1179 = property on="RESULT LAB02-2" class="Bool (strict)"("Visible"=w2042) -> ()  [unwired: 2 in, 2 out]
                n1180 = property on="RESULT LAB03-1" class="Bool (strict)"("Visible"=w2041) -> ()  [unwired: 2 in, 2 out]
                n1181 = property on="SET LAB01-1" class="Clust (strict)"("DisabledEnum"=w2036) -> ()  [unwired: 2 in, 2 out]
                n1182 = property on="SET LAB01-2" class="Clust (strict)"("DisabledEnum"=w2035) -> ()  [unwired: 2 in, 2 out]
                n1183 = property on="SET LAB02-1" class="Clust (strict)"("DisabledEnum"=w2034) -> ()  [unwired: 2 in, 2 out]
                n1184 = property on="SET LAB02-2" class="Clust (strict)"("DisabledEnum"=w2033) -> ()  [unwired: 2 in, 2 out]
                n1185 = property on="SET LAB03-1" class="Clust (strict)"("DisabledEnum"=w2032) -> ()  [unwired: 2 in, 2 out]
                n1186 = property on="O/I  LAB01-1" class="Bool (strict)"("DisabledEnum"=w2036) -> ()  [unwired: 2 in, 2 out]
                n1187 = property on="O/I  LAB01-2" class="Bool (strict)"("DisabledEnum"=w2035) -> ()  [unwired: 2 in, 2 out]
                n1188 = property on="O/I  LAB02-1" class="Bool (strict)"("DisabledEnum"=w2034) -> ()  [unwired: 2 in, 2 out]
                n1189 = property on="O/1  LAB02-2" class="Bool (strict)"("DisabledEnum"=w2033) -> ()  [unwired: 2 in, 2 out]
                n1190 = property on="O/I  LAB03-1" class="Bool (strict)"("DisabledEnum"=w2032) -> ()  [unwired: 2 in, 2 out]
              }
              frame #1 {
                n1191 = Select(t=2, s=w2066, f=0) -> (s? t:f=w2057:i32)
                n1192 = Select(t=2, s=w2065, f=0) -> (s? t:f=w2058:i32)
                n1193 = Select(t=2, s=w2062, f=0) -> (s? t:f=w2061:i32)
                n1194 = Select(t=2, s=w2063, f=0) -> (s? t:f=w2060:i32)
                n1195 = Select(t=2, s=w2064, f=0) -> (s? t:f=w2059:i32)
                n1196 = property on="SELECT LAB05-2" class="RadioBtnsControl (strict)"("DisabledEnum"=w2057) -> ()  [unwired: 2 in, 2 out]
                n1197 = property on="SELECT LAB05-1" class="RadioBtnsControl (strict)"("DisabledEnum"=w2058) -> ()  [unwired: 2 in, 2 out]
                n1198 = property on="SELECT LAB03-2" class="RadioBtnsControl (strict)"("DisabledEnum"=w2061) -> ()  [unwired: 2 in, 2 out]
                n1199 = property on="SELECT LAB04-1" class="RadioBtnsControl (strict)"("DisabledEnum"=w2060) -> ()  [unwired: 2 in, 2 out]
                n1200 = property on="SELECT LAB04-2" class="RadioBtnsControl (strict)"("DisabledEnum"=w2059) -> ()  [unwired: 2 in, 2 out]
                n1201 = property on="SET LAB05-2" class="Clust (strict)"("DisabledEnum"=w2057) -> ()  [unwired: 2 in, 2 out]
                n1202 = property on="SET LAB05-1" class="Clust (strict)"("DisabledEnum"=w2058) -> ()  [unwired: 2 in, 2 out]
                n1203 = property on="SET LAB03-2" class="Clust (strict)"("DisabledEnum"=w2061) -> ()  [unwired: 2 in, 2 out]
                n1204 = property on="SET LAB04-1" class="Clust (strict)"("DisabledEnum"=w2060) -> ()  [unwired: 2 in, 2 out]
                n1205 = property on="SET LAB04-2" class="Clust (strict)"("DisabledEnum"=w2059) -> ()  [unwired: 2 in, 2 out]
                n1206 = property on="O/I  LAB05-2" class="Bool (strict)"("DisabledEnum"=w2057) -> ()  [unwired: 2 in, 2 out]
                n1207 = property on="O/I  LAB05-1" class="Bool (strict)"("DisabledEnum"=w2058) -> ()  [unwired: 2 in, 2 out]
                n1208 = property on="O/I  LAB04-1" class="Bool (strict)"("DisabledEnum"=w2060) -> ()  [unwired: 2 in, 2 out]
                n1209 = property on="O/I  LAB04-2" class="Bool (strict)"("DisabledEnum"=w2059) -> ()  [unwired: 2 in, 2 out]
                n1210 = property on="O/I  LAB03-2" class="Bool (strict)"("DisabledEnum"=w2061) -> ()  [unwired: 2 in, 2 out]
                n1211 = Not(x=w2066) -> (.not. x?=w2067:bool)
                n1212 = Not(x=w2065) -> (.not. x?=w2068:bool)
                n1213 = Not(x=w2064) -> (.not. x?=w2069:bool)
                n1214 = property on="RESULT LAB05-2" class="Bool (strict)"("Visible"=w2067) -> ()  [unwired: 2 in, 2 out]
                n1215 = property on="RESULT LAB05-1" class="Bool (strict)"("Visible"=w2068) -> ()  [unwired: 2 in, 2 out]
                n1216 = Not(x=w2063) -> (.not. x?=w2070:bool)
                n1217 = property on="RESULT LAB04-2" class="Bool (strict)"("Visible"=w2069) -> ()  [unwired: 2 in, 2 out]
                n1218 = Not(x=w2062) -> (.not. x?=w2071:bool)
                n1219 = property on="RESULT LAB04-1" class="Bool (strict)"("Visible"=w2070) -> ()  [unwired: 2 in, 2 out]
                n1220 = property on="RESULT LAB03-2" class="Bool (strict)"("Visible"=w2071) -> ()  [unwired: 2 in, 2 out]
              }
              frame #2 {
                # "disable calibrate if any test running"
                n1221 = Or(x=w2093, y=w2092) -> (x .or. y?=w2086:bool)
                n1222 = Or(x=w2095, y=w2094) -> (x .or. y?=w2088:bool)
                n1223 = Or(x=w2099, y=w2098) -> (x .or. y?=w2090:bool)
                n1224 = Or(x=w2097, y=w2096) -> (x .or. y?=w2089:bool)
                n1225 = Or(x=w2101, y=w2100) -> (x .or. y?=w2091:bool)
                n1226 = Or(x=w2089, y=w2088) -> (x .or. y?=w2087:bool)
                n1227 = Or(x=w2091, y=w2090) -> (x .or. y?=w2085:bool)
                n1228 = Or(x=w2087, y=w2086) -> (x .or. y?=w2084:bool)
                n1229 = Or(x=w2085, y=w2084) -> (x .or. y?=w2083:bool)
                n1230 = case shown="False" w2083 {
                  tunnel: [0 2] -> w2082
                  frame False {
                  }
                  frame True {
                  }
                }
                n1231 = property on="MAIL SETTINGS" class="Clust (strict)"("DisabledEnum"=w2082) -> ()  [unwired: 2 in, 2 out]
                n1232 = property on="CALIBRATE" class="Bool (strict)"("DisabledEnum"=w2082) -> ()  [unwired: 2 in, 2 out]
              }
            }
          }
          frame #7 {
            # "drive jigs"
            n1233 = stacked-sequence {
              frame #0 {
                # "jig on"
                n1234 = local read "jig cycle"() -> (w2104:dbl)
                n1235 = Equal?(x=w2104, y=0) -> (x = y?=w2106:bool)
                n1236 = case shown="True" w2106 {
                  frame False {
                  }
                  frame True {
                    n1237 = local read "RUN LAB01-1"() -> (w2107:bool)
                    n1238 = local read "RUN LAB01-2"() -> (w2108:bool)
                    n1239 = local read "RUN LAB03-1"() -> (w2114:bool)
                    n1240 = local read "RUN LAB03-2"() -> (w2113:bool)
                    n1241 = local read "RUN LAB02-1"() -> (w2116:bool)
                    n1242 = local read "RUN LAB02-2"() -> (w2115:bool)
                    n1243 = local read "RUN LAB04-1"() -> (w2112:bool)
                    n1244 = local read "RUN LAB04-2"() -> (w2111:bool)
                    n1245 = local read "RUN LAB05-1"() -> (w2110:bool)
                    n1246 = local read "RUN LAB05-2"() -> (w2109:bool)
                    n1247 = local write "JIG LAB05-1"(w2110) -> ()
                    n1248 = local write "JIG LAB05-2"(w2109) -> ()
                    n1249 = local write "JIG LAB04-2"(w2111) -> ()
                    n1250 = local write "JIG LAB02-1"(w2116) -> ()
                    n1251 = local write "JIG LAB03-1"(w2114) -> ()
                    n1252 = local write "JIG LAB04-1"(w2112) -> ()
                    n1253 = local write "JIG LAB03-2"(w2113) -> ()
                    n1254 = local write "JIG LAB02-2"(w2115) -> ()
                    n1255 = local write "JIG LAB01-1"(w2107) -> ()
                    n1256 = local write "JIG LAB01-2"(w2108) -> ()
                  }
                }
              }
              frame #1 {
                # "jig off"
                n1257 = local read "jig cycle"() -> (w2119:dbl)
                n1258 = local read "on loops"() -> (w2118:dbl)
                n1259 = Equal?(x=w2119, y=w2118) -> (x = y?=w2117:bool)
                n1260 = case shown="True" w2117 {
                  frame False {
                  }
                  frame True {
                    w2170 = FALSE
                    w2171 = TRUE
                    w2169 = 2
                    n1261 = local read "SELECT LAB05-2"() -> (w2160:T3)
                    n1262 = local read "SELECT LAB04-2"() -> (w2162:T3)
                    n1263 = local read "SELECT LAB04-1"() -> (w2163:T3)
                    n1264 = local read "SELECT LAB05-1"() -> (w2161:T3)
                    n1265 = local read "SELECT LAB03-2"() -> (w2164:T3)
                    n1266 = local read "SELECT LAB02-1"() -> (w2167:T3)
                    n1267 = local read "SELECT LAB03-1"() -> (w2165:T3)
                    n1268 = local read "SELECT LAB02-2"() -> (w2166:T3)
                    n1269 = local read "SELECT LAB01-2"() -> (w2168:T3)
                    n1270 = local read "RUN LAB05-1"() -> (w2130:bool)
                    n1271 = local read "RUN LAB05-2"() -> (w2129:bool)
                    n1272 = local read "RUN LAB04-2"() -> (w2131:bool)
                    n1273 = local read "RUN LAB04-1"() -> (w2132:bool)
                    n1274 = local read "RUN LAB01-1"() -> (w2148:bool)
                    n1275 = local read "RUN LAB01-2"() -> (w2137:bool)
                    n1276 = local read "RUN LAB03-2"() -> (w2133:bool)
                    n1277 = local read "SELECT LAB01-1"() -> (w2172:T3)
                    n1278 = local read "RUN LAB03-1"() -> (w2134:bool)
                    n1279 = local read "RUN LAB02-1"() -> (w2136:bool)
                    n1280 = local read "RUN LAB02-2"() -> (w2135:bool)
                    n1281 = Equal?(x=w2169, y=w2165) -> (x = y?=w2143:bool)
                    n1282 = Equal?(x=w2169, y=w2164) -> (x = y?=w2142:bool)
                    n1283 = Equal?(x=w2169, y=w2163) -> (x = y?=w2141:bool)
                    n1284 = Equal?(x=w2169, y=w2162) -> (x = y?=w2140:bool)
                    n1285 = Equal?(x=w2169, y=w2161) -> (x = y?=w2139:bool)
                    n1286 = Equal?(x=w2169, y=w2160) -> (x = y?=w2138:bool)
                    n1287 = Equal?(x=w2169, y=w2172) -> (x = y?=w2149:bool)
                    n1288 = Equal?(x=w2169, y=w2167) -> (x = y?=w2145:bool)
                    n1289 = Equal?(x=w2169, y=w2166) -> (x = y?=w2144:bool)
                    n1290 = Equal?(x=w2169, y=w2168) -> (x = y?=w2146:bool)
                    n1291 = And(x=w2140, y=w2131) -> (x .and. y?=w2122:bool)
                    n1292 = And(x=w2143, y=w2134) -> (x .and. y?=w2125:bool)
                    n1293 = And(x=w2141, y=w2132) -> (x .and. y?=w2123:bool)
                    n1294 = And(x=w2138, y=w2129) -> (x .and. y?=w2120:bool)
                    n1295 = And(x=w2144, y=w2135) -> (x .and. y?=w2126:bool)
                    n1296 = And(x=w2142, y=w2133) -> (x .and. y?=w2124:bool)
                    n1297 = And(x=w2139, y=w2130) -> (x .and. y?=w2121:bool)
                    n1298 = And(x=w2146, y=w2137) -> (x .and. y?=w2128:bool)
                    n1299 = And(x=w2149, y=w2148) -> (x .and. y?=w2147:bool)
                    n1300 = And(x=w2145, y=w2136) -> (x .and. y?=w2127:bool)
                    n1301 = Select(t=w2171, s=w2147, f=w2170) -> (s? t:f=w2150:bool)
                    n1302 = Select(t=w2171, s=w2128, f=w2170) -> (s? t:f=w2151:bool)
                    n1303 = Select(t=w2171, s=w2127, f=w2170) -> (s? t:f=w2152:bool)
                    n1304 = Select(t=w2171, s=w2126, f=w2170) -> (s? t:f=w2153:bool)
                    n1305 = Select(t=w2171, s=w2125, f=w2170) -> (s? t:f=w2154:bool)
                    n1306 = Select(t=w2171, s=w2124, f=w2170) -> (s? t:f=w2155:bool)
                    n1307 = Select(t=w2171, s=w2123, f=w2170) -> (s? t:f=w2156:bool)
                    n1308 = Select(t=w2171, s=w2122, f=w2170) -> (s? t:f=w2157:bool)
                    n1309 = Select(t=w2171, s=w2121, f=w2170) -> (s? t:f=w2158:bool)
                    n1310 = Select(t=w2171, s=w2120, f=w2170) -> (s? t:f=w2159:bool)
                    n1311 = local write "JIG LAB03-2"(w2155) -> ()
                    n1312 = local write "JIG LAB02-1"(w2152) -> ()
                    n1313 = local write "JIG LAB02-2"(w2153) -> ()
                    n1314 = local write "JIG LAB01-2"(w2151) -> ()
                    n1315 = local write "JIG LAB03-1"(w2154) -> ()
                    n1316 = local write "JIG LAB01-1"(w2150) -> ()
                    n1317 = local write "JIG LAB05-2"(w2159) -> ()
                    n1318 = local write "JIG LAB04-1"(w2156) -> ()
                    n1319 = local write "JIG LAB05-1"(w2158) -> ()
                    n1320 = local write "JIG LAB04-2"(w2157) -> ()
                  }
                }
              }
            }
          }
          frame #8 {
            # "drive digital output"
            n1321 = local read "O/I  LAB05-2"() -> (w2178:bool)
            n1322 = local read "O/I  LAB05-1"() -> (w2180:bool)
            n1323 = local read "JIG LAB05-2"() -> (w2177:bool)
            n1324 = local read "O/I  LAB04-2"() -> (w2182:bool)
            n1325 = local read "JIG LAB05-1"() -> (w2179:bool)
            n1326 = local read "JIG LAB04-2"() -> (w2181:bool)
            n1327 = local read "O/1  LAB02-2"() -> (w2189:bool)
            n1328 = local read "O/I  LAB03-1"() -> (w2187:bool)
            n1329 = local read "O/I  LAB04-1"() -> (w2183:bool)
            n1330 = local read "O/I  LAB02-1"() -> (w2191:bool)
            n1331 = local read "O/I  LAB03-2"() -> (w2185:bool)
            n1332 = local read "JIG LAB04-1"() -> (w2176:bool)
            n1333 = local read "JIG LAB03-2"() -> (w2184:bool)
            n1334 = local read "O/I  LAB01-2"() -> (w2193:bool)
            n1335 = local read "JIG LAB02-1"() -> (w2190:bool)
            n1336 = local read "JIG LAB02-2"() -> (w2188:bool)
            n1337 = local read "JIG LAB03-1"() -> (w2186:bool)
            n1338 = local read "O/I  LAB01-1"() -> (w2195:bool)
            n1339 = local read "JIG LAB01-2"() -> (w2192:bool)
            n1340 = local read "JIG LAB01-1"() -> (w2194:bool)
            n1341 = Build Array(w2182, w2181, w2180, w2179, w2178, w2177) -> (w2173:bool[])
            n1342 = Build Array(w2188, w2187, w2186, w2185, w2184, w2183, w2176) -> (w2174:bool[])
            n1343 = Build Array(w2195, w2194, w2193, w2192, w2191, w2190, w2189) -> (w2175:bool[])
            n1344 = call "sub vi - Drive Relays All v6.vi"("Array #2"=w2173, "Array #1"=w2174, "Array #0"=w2175) -> ()  [unwired: 8 in, 1 out]
          }
          frame #9 {
            # "get temperature values"
            n1345 = stacked-sequence {
              frame #0 {
                n1346 = local read "jig cycle"() -> (w2196:dbl)
                n1347 = local read "on loops"() -> (w2199:dbl)
                n1348 = local read "jig cycle"() -> (w2201:dbl)
                n1349 = Add(x=w2199, y=2) -> (x+y=w2200:dbl)
                n1350 = Equal?(x=w2201, y=0) -> (x = y?=w2202:bool)
                n1351 = Equal?(x=w2196, y=w2200) -> (x = y?=w2197:bool)
                n1352 = case shown="True" w2202 {
                  frame False {
                  }
                  frame True {
                    w2214 = FALSE
                    w2215 = TRUE
                    n1353 = local write "TEMP update"(TRUE) -> ()
                    n1354 = call "sub vi - GET ALL TEMP v3.vi"("LA01-EN"=w2215, "LA02-EN"=w2215, "LA03-EN"=w2215, "LA04-EN"=w2214, "LA05-EN"=w2214, "Gen Cal Value"=1.0) -> ("LA01 TEMP"=w2213:T19, "LA02 TEMP"=w2211:T19, "LA03 TEMP"=w2210:T19)  [unwired: 4 in, 3 out]
                    n1355 = local write "LAB03 TEMP"(w2210) -> ()
                    n1356 = local write "LAB02 TEMP"(w2211) -> ()
                    n1357 = local write "LAB01 TEMP"(w2213) -> ()
                  }
                }
                n1358 = case shown="True" w2197 {
                  frame False {
                  }
                  frame True {
                    w2207 = TRUE
                    w2208 = FALSE
                    n1359 = local write "TEMP update"(TRUE) -> ()
                    n1360 = call "sub vi - GET ALL TEMP v3.vi"("LA01-EN"=w2208, "LA02-EN"=w2208, "LA03-EN"=w2208, "LA04-EN"=w2207, "LA05-EN"=w2207, "Gen Cal Value"=1.0) -> ("LA04 TEMP"=w2205:T19, "LA05 TEMP"=w2204:T19)  [unwired: 4 in, 4 out]
                    n1361 = local write "LAB04 TEMP"(w2205) -> ()
                    n1362 = local write "LAB05 TEMP"(w2204) -> ()
                  }
                }
              }
              frame #1 {
                n1363 = local read "CAL LAB01"() -> (w2233:T6)
                n1364 = local read "LAB01 TEMP"() -> (w2234:T10)
                n1365 = Unbundle By Name(w2234) -> ("T1 Live"=w2224:dbl, "T1 Neut"=w2223:dbl, "T2 Live"=w2222:dbl, "T2 Neut"=w2221:dbl)  [unwired: 2 out]
                n1366 = Unbundle By Name(w2233) -> ("1 (TL) cal"=w2220:dbl, "1 (TN) cal"=w2219:dbl, "2 (TL) cal"=w2218:dbl, "2 (TN) cal"=w2217:dbl)  [unwired: 6 out]
                n1367 = Multiply(x=w2224, y=w2220) -> (x*y=w2230:dbl)
                n1368 = Multiply(x=w2223, y=w2219) -> (x*y=w2229:dbl)
                n1369 = Multiply(x=w2222, y=w2218) -> (x*y=w2226:dbl)
                n1370 = Multiply(x=w2221, y=w2217) -> (x*y=w2225:dbl)
                n1371 = local read "SIG LAB01-2"() -> (w2228:T2)
                n1372 = local read "SIG LAB01-1"() -> (w2232:T2)
                n1373 = Bundle By Name(cluster=w2232, "Tmp Live"=w2230, "Tmp Neut"=w2229) -> (w2231:T2)
                n1374 = Bundle By Name(cluster=w2228, "Tmp Live"=w2226, "Tmp Neut"=w2225) -> (w2227:T2)
                n1375 = local write "SIG LAB01-1"(w2231) -> ()
                n1376 = local write "SIG LAB01-2"(w2227) -> ()
              }
              frame #2 {
                n1377 = local read "CAL LAB02"() -> (w2251:T7)
                n1378 = local read "LAB02 TEMP"() -> (w2252:T10)
                n1379 = Unbundle By Name(w2252) -> ("T1 Live"=w2242:dbl, "T1 Neut"=w2241:dbl, "T2 Live"=w2240:dbl, "T2 Neut"=w2239:dbl)  [unwired: 2 out]
                n1380 = Unbundle By Name(w2251) -> ("1 (TL) cal"=w2238:dbl, "1 (TN) cal"=w2237:dbl, "2 (TL) cal"=w2236:dbl, "2 (TN) cal"=w2235:dbl)  [unwired: 6 out]
                n1381 = Multiply(x=w2242, y=w2238) -> (x*y=w2248:dbl)
                n1382 = Multiply(x=w2241, y=w2237) -> (x*y=w2247:dbl)
                n1383 = Multiply(x=w2240, y=w2236) -> (x*y=w2244:dbl)
                n1384 = Multiply(x=w2239, y=w2235) -> (x*y=w2243:dbl)
                n1385 = local read "SIG LAB02-2"() -> (w2246:T2)
                n1386 = local read "SIG LAB02-1"() -> (w2250:T2)
                n1387 = Bundle By Name(cluster=w2250, "Tmp Live"=w2248, "Tmp Neut"=w2247) -> (w2249:T2)
                n1388 = Bundle By Name(cluster=w2246, "Tmp Live"=w2244, "Tmp Neut"=w2243) -> (w2245:T2)
                n1389 = local write "SIG LAB02-1"(w2249) -> ()
                n1390 = local write "SIG LAB02-2"(w2245) -> ()
              }
              frame #3 {
                n1391 = local read "CAL LAB03"() -> (w2269:T6)
                n1392 = local read "LAB03 TEMP"() -> (w2270:T10)
                n1393 = Unbundle By Name(w2270) -> ("T1 Live"=w2260:dbl, "T1 Neut"=w2259:dbl, "T2 Live"=w2258:dbl, "T2 Neut"=w2257:dbl)  [unwired: 2 out]
                n1394 = Unbundle By Name(w2269) -> ("1 (TL) cal"=w2256:dbl, "1 (TN) cal"=w2255:dbl, "2 (TL) cal"=w2254:dbl, "2 (TN) cal"=w2253:dbl)  [unwired: 6 out]
                n1395 = Multiply(x=w2260, y=w2256) -> (x*y=w2266:dbl)
                n1396 = Multiply(x=w2259, y=w2255) -> (x*y=w2265:dbl)
                n1397 = Multiply(x=w2258, y=w2254) -> (x*y=w2262:dbl)
                n1398 = Multiply(x=w2257, y=w2253) -> (x*y=w2261:dbl)
                n1399 = local read "SIG LAB03-2"() -> (w2264:T2)
                n1400 = local read "SIG LAB03-1"() -> (w2268:T2)
                n1401 = Bundle By Name(cluster=w2268, "Tmp Live"=w2266, "Tmp Neut"=w2265) -> (w2267:T2)
                n1402 = Bundle By Name(cluster=w2264, "Tmp Live"=w2262, "Tmp Neut"=w2261) -> (w2263:T2)
                n1403 = local write "SIG LAB03-1"(w2267) -> ()
                n1404 = local write "SIG LAB03-2"(w2263) -> ()
              }
              frame #4 {
                n1405 = local read "CAL LAB04"() -> (w2287:T6)
                n1406 = local read "LAB04 TEMP"() -> (w2288:T10)
                n1407 = Unbundle By Name(w2288) -> ("T1 Live"=w2278:dbl, "T1 Neut"=w2277:dbl, "T2 Live"=w2276:dbl, "T2 Neut"=w2275:dbl)  [unwired: 2 out]
                n1408 = Unbundle By Name(w2287) -> ("1 (TL) cal"=w2274:dbl, "1 (TN) cal"=w2273:dbl, "2 (TL) cal"=w2272:dbl, "2 (TN) cal"=w2271:dbl)  [unwired: 6 out]
                n1409 = Multiply(x=w2278, y=w2274) -> (x*y=w2284:dbl)
                n1410 = Multiply(x=w2277, y=w2273) -> (x*y=w2283:dbl)
                n1411 = Multiply(x=w2276, y=w2272) -> (x*y=w2280:dbl)
                n1412 = Multiply(x=w2275, y=w2271) -> (x*y=w2279:dbl)
                n1413 = local read "SIG LAB04-2"() -> (w2282:T2)
                n1414 = local read "SIG LAB04-1"() -> (w2286:T2)
                n1415 = Bundle By Name(cluster=w2286, "Tmp Live"=w2284, "Tmp Neut"=w2283) -> (w2285:T2)
                n1416 = Bundle By Name(cluster=w2282, "Tmp Live"=w2280, "Tmp Neut"=w2279) -> (w2281:T2)
                n1417 = local write "SIG LAB04-1"(w2285) -> ()
                n1418 = local write "SIG LAB04-2"(w2281) -> ()
              }
              frame #5 {
                n1419 = local read "CAL LAB05"() -> (w2305:T6)
                n1420 = local read "LAB05 TEMP"() -> (w2306:T10)
                n1421 = Unbundle By Name(w2306) -> ("T1 Live"=w2296:dbl, "T1 Neut"=w2295:dbl, "T2 Live"=w2294:dbl, "T2 Neut"=w2293:dbl)  [unwired: 2 out]
                n1422 = Unbundle By Name(w2305) -> ("1 (TL) cal"=w2292:dbl, "1 (TN) cal"=w2291:dbl, "2 (TL) cal"=w2290:dbl, "2 (TN) cal"=w2289:dbl)  [unwired: 6 out]
                n1423 = Multiply(x=w2296, y=w2292) -> (x*y=w2302:dbl)
                n1424 = Multiply(x=w2295, y=w2291) -> (x*y=w2301:dbl)
                n1425 = Multiply(x=w2294, y=w2290) -> (x*y=w2298:dbl)
                n1426 = Multiply(x=w2293, y=w2289) -> (x*y=w2297:dbl)
                n1427 = local read "SIG LAB05-2"() -> (w2300:T2)
                n1428 = local read "SIG LAB05-1"() -> (w2304:T2)
                n1429 = Bundle By Name(cluster=w2304, "Tmp Live"=w2302, "Tmp Neut"=w2301) -> (w2303:T2)
                n1430 = Bundle By Name(cluster=w2300, "Tmp Live"=w2298, "Tmp Neut"=w2297) -> (w2299:T2)
                n1431 = local write "SIG LAB05-1"(w2303) -> ()
                n1432 = local write "SIG LAB05-2"(w2299) -> ()
              }
            }
          }
          frame #10 {
            # "get analog values"
            n1433 = local read "on loops"() -> (w2313:dbl)
            n1434 = local read "jig cycle"() -> (w2310:dbl)
            n1435 = Add(x=w2313, y=1) -> (x+y=w2311:dbl)
            n1436 = Equal?(x=w2310, y=1) -> (x = y?=w2308:bool)
            n1437 = Equal?(x=w2310, y=w2311) -> (x = y?=w2309:bool)
            n1438 = Or(x=w2308, y=w2309) -> (x .or. y?=w2307:bool)
            n1439 = case shown="True" w2307 {
              frame False {
              }
              frame True {
                n1440 = call "sub vi - Read Analog All v8.vi"() -> ("Analog loop time"=w2321:dbl, "array GRAPH"=w2320:dynamicdata[], "LAB01"=w2319:T20, "LAB02"=w2318:T21, "LAB03"=w2317:T22, "LAB04"=w2316:T23, "array ERROR"=w2322:errorcluster[], "LAB05"=w2315:T24)  [unwired: 8 in]
                n1441 = stacked-sequence {
                  tunnel: w2322 -> [w2325 _ _ _ _ _]
                  tunnel: w2321 -> [w2324 _ _ _ _ _]
                  tunnel: w2320 -> [w2323 _ _ _ _ _]
                  tunnel: w2319 -> [_ w2370 _ _ _ _]
                  tunnel: w2318 -> [_ _ w2371 _ _ _]
                  tunnel: w2317 -> [_ _ _ w2396 _ _]
                  tunnel: w2316 -> [_ _ _ _ w2419 _]
                  tunnel: w2315 -> [_ _ _ _ _ w2444]
                  frame #0 {
                    n1442 = local write "AI update"(TRUE) -> ()
                    n1443 = Index Array(array=w2323, index=6) -> (element=→"LAB04-1 (GRAPH)":dynamicdata)
                    n1444 = Index Array(array=w2323, index=7) -> (element=→"LAB04-2 (GRAPH)":dynamicdata)
                    n1445 = Index Array(array=w2323, index=9) -> (element=→"LAB05-2 (GRAPH)":dynamicdata)
                    n1446 = Index Array(array=w2323, index=8) -> (element=→"LAB05-1 (GRAPH)":dynamicdata)
                    n1447 = Index Array(array=w2323, index=5) -> (element=→"LAB03-2 (GRAPH)":dynamicdata)
                    n1448 = Index Array(array=w2323, index=0) -> (element=→"LAB01-1 (GRAPH)":dynamicdata)
                    n1449 = Index Array(array=w2323, index=1) -> (element=→"LAB01-2 (GRAPH)":dynamicdata)
                    n1450 = Index Array(array=w2323, index=2) -> (element=→"LAB02-1 (GRAPH)":dynamicdata)
                    n1451 = Index Array(array=w2323, index=3) -> (element=→"LAB02-2 (GRAPH)":dynamicdata)
                    n1452 = Index Array(array=w2323, index=4) -> (element=→"LAB03-1 (GRAPH)":dynamicdata)
                    "AI loop time" <- w2324
                    "Analog Error Array" <- w2325
                  }
                  frame #1 {
                    n1453 = local read "CAL LAB01"() -> (w2369:T6)
                    n1454 = Unbundle By Name(w2370) -> ("LAB01-1 (A)"=w2368:dbl, "LAB01-1 (V)"=w2367:dbl, "LAB01-1 (PF)"=w2366:dbl, "LAB01-2 (A)"=w2365:dbl, "LAB01-2 (V)"=w2364:dbl, "LAB01-2 (PF)"=w2363:dbl)
                    n1455 = Unbundle By Name(w2369) -> ("1  (A) cal"=w2362:dbl, "1 (V) cal"=w2361:dbl, "1 (PF) cal"=w2360:dbl, "2 (A) cal"=w2359:dbl, "2 (V) cal"=w2358:dbl, "2 (PF) cal"=w2357:dbl)  [unwired: 4 out]
                    n1456 = Multiply(x=w2368, y=w2362) -> (x*y=w2355:dbl)
                    n1457 = Multiply(x=w2367, y=w2361) -> (x*y=w2354:dbl)
                    n1458 = Multiply(x=w2366, y=w2360) -> (x*y=w2353:dbl)
                    n1459 = Multiply(x=w2365, y=w2359) -> (x*y=w2349:dbl)
                    n1460 = Multiply(x=w2364, y=w2358) -> (x*y=w2348:dbl)
                    n1461 = Multiply(x=w2363, y=w2357) -> (x*y=w2347:dbl)
                    n1462 = local read "SIG LAB01-1"() -> (w2356:T2)
                    n1463 = local read "SIG LAB01-2"() -> (w2351:T2)
                    n1464 = Bundle By Name(cluster=w2356, "AMPS"=w2355, "VOLTS"=w2354, "PF"=w2353) -> (w2352:T2)
                    n1465 = Bundle By Name(cluster=w2351, "AMPS"=w2349, "VOLTS"=w2348, "PF"=w2347) -> (w2350:T2)
                    n1466 = local write "SIG LAB01-2"(w2350) -> ()
                    n1467 = local write "SIG LAB01-1"(w2352) -> ()
                  }
                  frame #2 {
                    n1468 = local read "CAL LAB02"() -> (w2394:T7)
                    n1469 = Unbundle By Name(w2371) -> ("LAB02-1 (A)"=w2393:dbl, "LAB02-1 (V)"=w2392:dbl, "LAB02-1 (PF)"=w2391:dbl, "LAB02-2 (A)"=w2390:dbl, "LAB02-2 (V)"=w2389:dbl, "LAB02-2 (PF)"=w2388:dbl)
                    n1470 = Unbundle By Name(w2394) -> ("1 (A) cal"=w2387:dbl, "1 (V) cal"=w2386:dbl, "1 (PF) cal"=w2385:dbl, "2 (A) cal"=w2384:dbl, "2 (V) cal"=w2383:dbl, "2 (PF) cal"=w2382:dbl)  [unwired: 4 out]
                    n1471 = Multiply(x=w2393, y=w2387) -> (x*y=w2380:dbl)
                    n1472 = Multiply(x=w2392, y=w2386) -> (x*y=w2379:dbl)
                    n1473 = Multiply(x=w2391, y=w2385) -> (x*y=w2378:dbl)
                    n1474 = Multiply(x=w2390, y=w2384) -> (x*y=w2374:dbl)
                    n1475 = Multiply(x=w2389, y=w2383) -> (x*y=w2373:dbl)
                    n1476 = Multiply(x=w2388, y=w2382) -> (x*y=w2372:dbl)
                    n1477 = local read "SIG LAB02-1"() -> (w2381:T2)
                    n1478 = local read "SIG LAB02-2"() -> (w2376:T2)
                    n1479 = Bundle By Name(cluster=w2381, "AMPS"=w2380, "VOLTS"=w2379, "PF"=w2378) -> (w2377:T2)
                    n1480 = Bundle By Name(cluster=w2376, "AMPS"=w2374, "VOLTS"=w2373, "PF"=w2372) -> (w2375:T2)
                    n1481 = local write "SIG LAB02-2"(w2375) -> ()
                    n1482 = local write "SIG LAB02-1"(w2377) -> ()
                  }
                  frame #3 {
                    n1483 = local read "CAL LAB03"() -> (w2418:T6)
                    n1484 = Unbundle By Name(w2396) -> ("LAB03-1 (A)"=w2417:dbl, "LAB03-1 (V)"=w2416:dbl, "LAB03-1 (PF)"=w2415:dbl, "LAB03-2 (A)"=w2414:dbl, "LAB03-2 (V)"=w2413:dbl, "LAB03-2 (PF)"=w2412:dbl)
                    n1485 = Unbundle By Name(w2418) -> ("1  (A) cal"=w2411:dbl, "1 (V) cal"=w2410:dbl, "1 (PF) cal"=w2409:dbl, "2 (A) cal"=w2408:dbl, "2 (V) cal"=w2407:dbl, "2 (PF) cal"=w2406:dbl)  [unwired: 4 out]
                    n1486 = Multiply(x=w2417, y=w2411) -> (x*y=w2404:dbl)
                    n1487 = Multiply(x=w2416, y=w2410) -> (x*y=w2395:dbl)
                    n1488 = Multiply(x=w2415, y=w2409) -> (x*y=w2403:dbl)
                    n1489 = Multiply(x=w2414, y=w2408) -> (x*y=w2399:dbl)
                    n1490 = Multiply(x=w2413, y=w2407) -> (x*y=w2398:dbl)
                    n1491 = Multiply(x=w2412, y=w2406) -> (x*y=w2397:dbl)
                    n1492 = local read "SIG LAB03-1"() -> (w2405:T2)
                    n1493 = local read "SIG LAB03-2"() -> (w2401:T2)
                    n1494 = Bundle By Name(cluster=w2405, "AMPS"=w2404, "VOLTS"=w2395, "PF"=w2403) -> (w2402:T2)
                    n1495 = Bundle By Name(cluster=w2401, "AMPS"=w2399, "VOLTS"=w2398, "PF"=w2397) -> (w2400:T2)
                    n1496 = local write "SIG LAB03-2"(w2400) -> ()
                    n1497 = local write "SIG LAB03-1"(w2402) -> ()
                  }
                  frame #4 {
                    n1498 = local read "CAL LAB04"() -> (w2442:T6)
                    n1499 = Unbundle By Name(w2419) -> ("LAB04-1 (A)"=w2441:dbl, "LAB04-1 (V)"=w2440:dbl, "LAB04-1 (PF)"=w2439:dbl, "LAB04-2 (A)"=w2438:dbl, "LAB04-2 (V)"=w2437:dbl, "LAB04-2 (PF)"=w2436:dbl)
                    n1500 = Unbundle By Name(w2442) -> ("1  (A) cal"=w2435:dbl, "1 (V) cal"=w2434:dbl, "1 (PF) cal"=w2433:dbl, "2 (A) cal"=w2432:dbl, "2 (V) cal"=w2431:dbl, "2 (PF) cal"=w2430:dbl)  [unwired: 4 out]
                    n1501 = Multiply(x=w2441, y=w2435) -> (x*y=w2428:dbl)
                    n1502 = Multiply(x=w2440, y=w2434) -> (x*y=w2427:dbl)
                    n1503 = Multiply(x=w2439, y=w2433) -> (x*y=w2426:dbl)
                    n1504 = Multiply(x=w2438, y=w2432) -> (x*y=w2422:dbl)
                    n1505 = Multiply(x=w2437, y=w2431) -> (x*y=w2421:dbl)
                    n1506 = Multiply(x=w2436, y=w2430) -> (x*y=w2420:dbl)
                    n1507 = local read "SIG LAB04-1"() -> (w2429:T2)
                    n1508 = local read "SIG LAB04-2"() -> (w2424:T2)
                    n1509 = Bundle By Name(cluster=w2429, "AMPS"=w2428, "VOLTS"=w2427, "PF"=w2426) -> (w2425:T2)
                    n1510 = Bundle By Name(cluster=w2424, "AMPS"=w2422, "VOLTS"=w2421, "PF"=w2420) -> (w2423:T2)
                    n1511 = local write "SIG LAB04-2"(w2423) -> ()
                    n1512 = local write "SIG LAB04-1"(w2425) -> ()
                  }
                  frame #5 {
                    n1513 = local read "CAL LAB05"() -> (w2466:T6)
                    n1514 = Unbundle By Name(w2444) -> ("LAB05-1 (A)"=w2465:dbl, "LAB05-1 (V)"=w2443:dbl, "LAB05-1 (PF)"=w2464:dbl, "LAB05-2 (A)"=w2463:dbl, "LAB05-2 (V)"=w2462:dbl, "LAB05-2 (PF)"=w2461:dbl)
                    n1515 = Unbundle By Name(w2466) -> ("1  (A) cal"=w2460:dbl, "1 (V) cal"=w2459:dbl, "1 (PF) cal"=w2458:dbl, "2 (A) cal"=w2457:dbl, "2 (V) cal"=w2456:dbl, "2 (PF) cal"=w2455:dbl)  [unwired: 4 out]
                    n1516 = Multiply(x=w2465, y=w2460) -> (x*y=w2453:dbl)
                    n1517 = Multiply(x=w2443, y=w2459) -> (x*y=w2452:dbl)
                    n1518 = Multiply(x=w2464, y=w2458) -> (x*y=w2451:dbl)
                    n1519 = Multiply(x=w2463, y=w2457) -> (x*y=w2447:dbl)
                    n1520 = Multiply(x=w2462, y=w2456) -> (x*y=w2446:dbl)
                    n1521 = Multiply(x=w2461, y=w2455) -> (x*y=w2445:dbl)
                    n1522 = local read "SIG LAB05-1"() -> (w2454:T2)
                    n1523 = local read "SIG LAB05-2"() -> (w2449:T2)
                    n1524 = Bundle By Name(cluster=w2454, "AMPS"=w2453, "VOLTS"=w2452, "PF"=w2451) -> (w2450:T2)
                    n1525 = Bundle By Name(cluster=w2449, "AMPS"=w2447, "VOLTS"=w2446, "PF"=w2445) -> (w2448:T2)
                    n1526 = local write "SIG LAB05-2"(w2448) -> ()
                    n1527 = local write "SIG LAB05-1"(w2450) -> ()
                  }
                }
              }
            }
          }
          frame #11 {
            # "save test data to file"
            n1528 = local read "on loops"() -> (w2483:dbl)
            n1529 = local read "jig cycle"() -> (w2480:dbl)
            n1530 = Add(x=w2483, y=2) -> (x+y=w2481:dbl)
            n1531 = Equal?(x=w2480, y=1) -> (x = y?=w2478:bool)
            n1532 = Equal?(x=w2480, y=w2481) -> (x = y?=w2479:bool)
            n1533 = Or(x=w2478, y=w2479) -> (x .or. y?=w2477:bool)
            n1534 = case shown="True" w2477 {
              tunnel: w2476 -> [_ w2494]
              tunnel: w2475 -> [_ w2493]
              tunnel: w2474 -> [_ w2492]
              tunnel: w2473 -> [_ w2491]
              tunnel: w2472 -> [_ w2490]
              tunnel: w2471 -> [_ w2489]
              tunnel: w2470 -> [_ w2488]
              tunnel: w2469 -> [_ w2487]
              tunnel: w2468 -> [_ w2486]
              tunnel: w2467 -> [_ w2485]
              frame False {
              }
              frame True {
                n1535 = stacked-sequence {
                  tunnel: w2494 -> [w2495 _ _ _ _ _ _ _ _ _]
                  tunnel: w2493 -> [_ w2540 _ _ _ _ _ _ _ _]
                  tunnel: w2492 -> [_ _ w2585 _ _ _ _ _ _ _]
                  tunnel: w2491 -> [_ _ _ w2630 _ _ _ _ _ _]
                  tunnel: w2490 -> [_ _ _ _ w2675 _ _ _ _ _]
                  tunnel: w2489 -> [_ _ _ _ _ w2720 _ _ _ _]
                  tunnel: w2488 -> [_ _ _ _ _ _ w2765 _ _ _]
                  tunnel: w2487 -> [_ _ _ _ _ _ _ w2810 _ _]
                  tunnel: w2486 -> [_ _ _ _ _ _ _ _ w2855 _]
                  tunnel: w2485 -> [_ _ _ _ _ _ _ _ _ w2900]
                  frame #0 {
                    # "LAB01-1"
                    n1536 = case shown="True" w2495 {
                      frame False {
                      }
                      frame True {
                        n1537 = local read "DISP LAB01-1"() -> (w2537:T4)
                        n1538 = local read "SIG LAB01-1"() -> (w2538:T2)
                        n1539 = local read "TDMS LAB01-1"() -> (w2539:refnum<k34>)
                        n1540 = Build Array("TEMP Neut") -> (w2503:string[])
                        n1541 = Build Array("CYCLE") -> (w2498:string[])
                        n1542 = Build Array("TEMP Live") -> (w2508:string[])
                        n1543 = Build Array("PF") -> (w2513:string[])
                        n1544 = Build Array("AMPS") -> (w2534:string[])
                        n1545 = Build Array("VOLTS") -> (w2525:string[])
                        n1546 = Unbundle(w2538) -> ("AMPS"=w2533:dbl, "VOLTS"=w2522:dbl, "PF"=w2521:dbl, "Tmp Live"=w2520:dbl, "Tmp Neut"=w2523:dbl)
                        n1547 = Unbundle(w2537) -> ("CYCLE"=w2518:dbl)  [unwired: 2 out]
                        n1548 = Build Array(w2522) -> (w2519:dbl[])
                        n1549 = Build Array(w2521) -> (w2512:dbl[])
                        n1550 = Build Array(w2520) -> (w2507:dbl[])
                        n1551 = Build Array(w2523) -> (w2502:dbl[])
                        n1552 = Build Array(w2533) -> (w2532:dbl[])
                        n1553 = Build Array(w2518) -> (w2497:dbl[])
                        n1554 = TDMS Write(0:w2539, 5:"LAB01-1 TEST VALUES", 7:w2534, 9:w2532) -> (4:w2527:refnum<k34>, 6:w2526:string, 15:w2514:errorcluster)  [unwired: 2 in, 1 out]
                        n1555 = TDMS Write(0:w2527, 5:w2526, 7:w2525, 9:w2519, 11:w2514) -> (4:w2517:refnum<k34>, 6:w2516:string, 15:w2515:errorcluster)  [unwired: 1 in, 1 out]
                        n1556 = TDMS Write(0:w2517, 5:w2516, 7:w2513, 9:w2512, 11:w2515) -> (4:w2511:refnum<k34>, 6:w2510:string, 15:w2509:errorcluster)  [unwired: 1 in, 1 out]
                        n1557 = TDMS Write(0:w2511, 5:w2510, 7:w2508, 9:w2507, 11:w2509) -> (4:w2506:refnum<k34>, 6:w2505:string, 15:w2504:errorcluster)  [unwired: 1 in, 1 out]
                        n1558 = TDMS Write(0:w2506, 5:w2505, 7:w2503, 9:w2502, 11:w2504) -> (4:w2501:refnum<k34>, 6:w2500:string, 15:w2499:errorcluster)  [unwired: 1 in, 1 out]
                        n1559 = TDMS Write(0:w2501, 5:w2500, 7:w2498, 9:w2497, 11:w2499) -> (15:w2496:errorcluster)  [unwired: 1 in, 3 out]
                        n1560 = local write "data file error"(w2496) -> ()
                      }
                    }
                  }
                  frame #1 {
                    # "LAB01-2"
                    n1561 = case shown="True" w2540 {
                      frame False {
                      }
                      frame True {
                        n1562 = local read "DISP LAB01-2"() -> (w2582:T4)
                        n1563 = local read "SIG LAB01-2"() -> (w2583:T2)
                        n1564 = local read "TDMS LAB01-2"() -> (w2584:refnum<k34>)
                        n1565 = Build Array("TEMP Neut") -> (w2548:string[])
                        n1566 = Build Array("CYCLE") -> (w2543:string[])
                        n1567 = Build Array("TEMP Live") -> (w2553:string[])
                        n1568 = Build Array("PF") -> (w2558:string[])
                        n1569 = Build Array("AMPS") -> (w2579:string[])
                        n1570 = Build Array("VOLTS") -> (w2570:string[])
                        n1571 = Unbundle(w2583) -> ("AMPS"=w2578:dbl, "VOLTS"=w2567:dbl, "PF"=w2566:dbl, "Tmp Live"=w2565:dbl, "Tmp Neut"=w2568:dbl)
                        n1572 = Unbundle(w2582) -> ("CYCLE"=w2563:dbl)  [unwired: 2 out]
                        n1573 = Build Array(w2567) -> (w2564:dbl[])
                        n1574 = Build Array(w2566) -> (w2557:dbl[])
                        n1575 = Build Array(w2565) -> (w2552:dbl[])
                        n1576 = Build Array(w2568) -> (w2547:dbl[])
                        n1577 = Build Array(w2578) -> (w2577:dbl[])
                        n1578 = Build Array(w2563) -> (w2542:dbl[])
                        n1579 = TDMS Write(0:w2584, 5:"LAB01-2 TEST VALUES", 7:w2579, 9:w2577) -> (4:w2572:refnum<k34>, 6:w2571:string, 15:w2559:errorcluster)  [unwired: 2 in, 1 out]
                        n1580 = TDMS Write(0:w2572, 5:w2571, 7:w2570, 9:w2564, 11:w2559) -> (4:w2562:refnum<k34>, 6:w2561:string, 15:w2560:errorcluster)  [unwired: 1 in, 1 out]
                        n1581 = TDMS Write(0:w2562, 5:w2561, 7:w2558, 9:w2557, 11:w2560) -> (4:w2556:refnum<k34>, 6:w2555:string, 15:w2554:errorcluster)  [unwired: 1 in, 1 out]
                        n1582 = TDMS Write(0:w2556, 5:w2555, 7:w2553, 9:w2552, 11:w2554) -> (4:w2551:refnum<k34>, 6:w2550:string, 15:w2549:errorcluster)  [unwired: 1 in, 1 out]
                        n1583 = TDMS Write(0:w2551, 5:w2550, 7:w2548, 9:w2547, 11:w2549) -> (4:w2546:refnum<k34>, 6:w2545:string, 15:w2544:errorcluster)  [unwired: 1 in, 1 out]
                        n1584 = TDMS Write(0:w2546, 5:w2545, 7:w2543, 9:w2542, 11:w2544) -> (15:w2541:errorcluster)  [unwired: 1 in, 3 out]
                        n1585 = local write "data file error"(w2541) -> ()
                      }
                    }
                  }
                  frame #2 {
                    # "LAB02-1"
                    n1586 = case shown="True" w2585 {
                      frame False {
                      }
                      frame True {
                        n1587 = local read "DISP LAB02-1"() -> (w2627:T4)
                        n1588 = local read "SIG LAB02-1"() -> (w2628:T2)
                        n1589 = local read "TDMS LAB02-1"() -> (w2629:refnum<k34>)
                        n1590 = Build Array("TEMP Neut") -> (w2593:string[])
                        n1591 = Build Array("CYCLE") -> (w2588:string[])
                        n1592 = Build Array("TEMP Live") -> (w2598:string[])
                        n1593 = Build Array("PF") -> (w2603:string[])
                        n1594 = Build Array("AMPS") -> (w2624:string[])
                        n1595 = Build Array("VOLTS") -> (w2615:string[])
                        n1596 = Unbundle(w2628) -> ("AMPS"=w2623:dbl, "VOLTS"=w2612:dbl, "PF"=w2611:dbl, "Tmp Live"=w2610:dbl, "Tmp Neut"=w2613:dbl)
                        n1597 = Unbundle(w2627) -> ("CYCLE"=w2608:dbl)  [unwired: 2 out]
                        n1598 = Build Array(w2612) -> (w2609:dbl[])
                        n1599 = Build Array(w2611) -> (w2602:dbl[])
                        n1600 = Build Array(w2610) -> (w2597:dbl[])
                        n1601 = Build Array(w2613) -> (w2592:dbl[])
                        n1602 = Build Array(w2623) -> (w2622:dbl[])
                        n1603 = Build Array(w2608) -> (w2587:dbl[])
                        n1604 = TDMS Write(0:w2629, 5:"LAB02-1 TEST VALUES", 7:w2624, 9:w2622) -> (4:w2617:refnum<k34>, 6:w2616:string, 15:w2604:errorcluster)  [unwired: 2 in, 1 out]
                        n1605 = TDMS Write(0:w2617, 5:w2616, 7:w2615, 9:w2609, 11:w2604) -> (4:w2607:refnum<k34>, 6:w2606:string, 15:w2605:errorcluster)  [unwired: 1 in, 1 out]
                        n1606 = TDMS Write(0:w2607, 5:w2606, 7:w2603, 9:w2602, 11:w2605) -> (4:w2601:refnum<k34>, 6:w2600:string, 15:w2599:errorcluster)  [unwired: 1 in, 1 out]
                        n1607 = TDMS Write(0:w2601, 5:w2600, 7:w2598, 9:w2597, 11:w2599) -> (4:w2596:refnum<k34>, 6:w2595:string, 15:w2594:errorcluster)  [unwired: 1 in, 1 out]
                        n1608 = TDMS Write(0:w2596, 5:w2595, 7:w2593, 9:w2592, 11:w2594) -> (4:w2591:refnum<k34>, 6:w2590:string, 15:w2589:errorcluster)  [unwired: 1 in, 1 out]
                        n1609 = TDMS Write(0:w2591, 5:w2590, 7:w2588, 9:w2587, 11:w2589) -> (15:w2586:errorcluster)  [unwired: 1 in, 3 out]
                        n1610 = local write "data file error"(w2586) -> ()
                      }
                    }
                  }
                  frame #3 {
                    # "LAB02-2"
                    n1611 = case shown="True" w2630 {
                      frame False {
                      }
                      frame True {
                        n1612 = local read "DISP LAB02-2"() -> (w2672:T4)
                        n1613 = local read "SIG LAB02-2"() -> (w2673:T2)
                        n1614 = local read "TDMS LAB02-2"() -> (w2674:refnum<k34>)
                        n1615 = Build Array("TEMP Neut") -> (w2638:string[])
                        n1616 = Build Array("CYCLE") -> (w2633:string[])
                        n1617 = Build Array("TEMP Live") -> (w2643:string[])
                        n1618 = Build Array("PF") -> (w2648:string[])
                        n1619 = Build Array("AMPS") -> (w2669:string[])
                        n1620 = Build Array("VOLTS") -> (w2660:string[])
                        n1621 = Unbundle(w2673) -> ("AMPS"=w2668:dbl, "VOLTS"=w2657:dbl, "PF"=w2656:dbl, "Tmp Live"=w2655:dbl, "Tmp Neut"=w2658:dbl)
                        n1622 = Unbundle(w2672) -> ("CYCLE"=w2653:dbl)  [unwired: 2 out]
                        n1623 = Build Array(w2657) -> (w2654:dbl[])
                        n1624 = Build Array(w2656) -> (w2647:dbl[])
                        n1625 = Build Array(w2655) -> (w2642:dbl[])
                        n1626 = Build Array(w2658) -> (w2637:dbl[])
                        n1627 = Build Array(w2668) -> (w2667:dbl[])
                        n1628 = Build Array(w2653) -> (w2632:dbl[])
                        n1629 = TDMS Write(0:w2674, 5:"LAB02-2 TEST VALUES", 7:w2669, 9:w2667) -> (4:w2662:refnum<k34>, 6:w2661:string, 15:w2649:errorcluster)  [unwired: 2 in, 1 out]
                        n1630 = TDMS Write(0:w2662, 5:w2661, 7:w2660, 9:w2654, 11:w2649) -> (4:w2652:refnum<k34>, 6:w2651:string, 15:w2650:errorcluster)  [unwired: 1 in, 1 out]
                        n1631 = TDMS Write(0:w2652, 5:w2651, 7:w2648, 9:w2647, 11:w2650) -> (4:w2646:refnum<k34>, 6:w2645:string, 15:w2644:errorcluster)  [unwired: 1 in, 1 out]
                        n1632 = TDMS Write(0:w2646, 5:w2645, 7:w2643, 9:w2642, 11:w2644) -> (4:w2641:refnum<k34>, 6:w2640:string, 15:w2639:errorcluster)  [unwired: 1 in, 1 out]
                        n1633 = TDMS Write(0:w2641, 5:w2640, 7:w2638, 9:w2637, 11:w2639) -> (4:w2636:refnum<k34>, 6:w2635:string, 15:w2634:errorcluster)  [unwired: 1 in, 1 out]
                        n1634 = TDMS Write(0:w2636, 5:w2635, 7:w2633, 9:w2632, 11:w2634) -> (15:w2631:errorcluster)  [unwired: 1 in, 3 out]
                        n1635 = local write "data file error"(w2631) -> ()
                      }
                    }
                  }
                  frame #4 {
                    # "LAB03-1"
                    n1636 = case shown="True" w2675 {
                      frame False {
                      }
                      frame True {
                        n1637 = local read "DISP LAB03-1"() -> (w2717:T4)
                        n1638 = local read "SIG LAB03-1"() -> (w2718:T2)
                        n1639 = local read "TDMS LAB03-1"() -> (w2719:refnum<k34>)
                        n1640 = Build Array("TEMP Neut") -> (w2683:string[])
                        n1641 = Build Array("CYCLE") -> (w2678:string[])
                        n1642 = Build Array("TEMP Live") -> (w2688:string[])
                        n1643 = Build Array("PF") -> (w2693:string[])
                        n1644 = Build Array("AMPS") -> (w2714:string[])
                        n1645 = Build Array("VOLTS") -> (w2705:string[])
                        n1646 = Unbundle(w2718) -> ("AMPS"=w2713:dbl, "VOLTS"=w2702:dbl, "PF"=w2701:dbl, "Tmp Live"=w2700:dbl, "Tmp Neut"=w2703:dbl)
                        n1647 = Unbundle(w2717) -> ("CYCLE"=w2698:dbl)  [unwired: 2 out]
                        n1648 = Build Array(w2702) -> (w2699:dbl[])
                        n1649 = Build Array(w2701) -> (w2692:dbl[])
                        n1650 = Build Array(w2700) -> (w2687:dbl[])
                        n1651 = Build Array(w2703) -> (w2682:dbl[])
                        n1652 = Build Array(w2713) -> (w2712:dbl[])
                        n1653 = Build Array(w2698) -> (w2677:dbl[])
                        n1654 = TDMS Write(0:w2719, 5:"LAB03-1 TEST VALUES", 7:w2714, 9:w2712) -> (4:w2707:refnum<k34>, 6:w2706:string, 15:w2694:errorcluster)  [unwired: 2 in, 1 out]
                        n1655 = TDMS Write(0:w2707, 5:w2706, 7:w2705, 9:w2699, 11:w2694) -> (4:w2697:refnum<k34>, 6:w2696:string, 15:w2695:errorcluster)  [unwired: 1 in, 1 out]
                        n1656 = TDMS Write(0:w2697, 5:w2696, 7:w2693, 9:w2692, 11:w2695) -> (4:w2691:refnum<k34>, 6:w2690:string, 15:w2689:errorcluster)  [unwired: 1 in, 1 out]
                        n1657 = TDMS Write(0:w2691, 5:w2690, 7:w2688, 9:w2687, 11:w2689) -> (4:w2686:refnum<k34>, 6:w2685:string, 15:w2684:errorcluster)  [unwired: 1 in, 1 out]
                        n1658 = TDMS Write(0:w2686, 5:w2685, 7:w2683, 9:w2682, 11:w2684) -> (4:w2681:refnum<k34>, 6:w2680:string, 15:w2679:errorcluster)  [unwired: 1 in, 1 out]
                        n1659 = TDMS Write(0:w2681, 5:w2680, 7:w2678, 9:w2677, 11:w2679) -> (15:w2676:errorcluster)  [unwired: 1 in, 3 out]
                        n1660 = local write "data file error"(w2676) -> ()
                      }
                    }
                  }
                  frame #5 {
                    # "LAB03-2"
                    n1661 = case shown="True" w2720 {
                      frame False {
                      }
                      frame True {
                        n1662 = local read "DISP LAB03-2"() -> (w2762:T4)
                        n1663 = local read "SIG LAB03-2"() -> (w2763:T2)
                        n1664 = local read "TDMS LAB03-2"() -> (w2764:refnum<k34>)
                        n1665 = Build Array("TEMP Neut") -> (w2728:string[])
                        n1666 = Build Array("CYCLE") -> (w2723:string[])
                        n1667 = Build Array("TEMP Live") -> (w2733:string[])
                        n1668 = Build Array("PF") -> (w2738:string[])
                        n1669 = Build Array("AMPS") -> (w2759:string[])
                        n1670 = Build Array("VOLTS") -> (w2750:string[])
                        n1671 = Unbundle(w2763) -> ("AMPS"=w2758:dbl, "VOLTS"=w2747:dbl, "PF"=w2746:dbl, "Tmp Live"=w2745:dbl, "Tmp Neut"=w2748:dbl)
                        n1672 = Unbundle(w2762) -> ("CYCLE"=w2743:dbl)  [unwired: 2 out]
                        n1673 = Build Array(w2747) -> (w2744:dbl[])
                        n1674 = Build Array(w2746) -> (w2737:dbl[])
                        n1675 = Build Array(w2745) -> (w2732:dbl[])
                        n1676 = Build Array(w2748) -> (w2727:dbl[])
                        n1677 = Build Array(w2758) -> (w2757:dbl[])
                        n1678 = Build Array(w2743) -> (w2722:dbl[])
                        n1679 = TDMS Write(0:w2764, 5:"LAB03-2 TEST VALUES", 7:w2759, 9:w2757) -> (4:w2752:refnum<k34>, 6:w2751:string, 15:w2739:errorcluster)  [unwired: 2 in, 1 out]
                        n1680 = TDMS Write(0:w2752, 5:w2751, 7:w2750, 9:w2744, 11:w2739) -> (4:w2742:refnum<k34>, 6:w2741:string, 15:w2740:errorcluster)  [unwired: 1 in, 1 out]
                        n1681 = TDMS Write(0:w2742, 5:w2741, 7:w2738, 9:w2737, 11:w2740) -> (4:w2736:refnum<k34>, 6:w2735:string, 15:w2734:errorcluster)  [unwired: 1 in, 1 out]
                        n1682 = TDMS Write(0:w2736, 5:w2735, 7:w2733, 9:w2732, 11:w2734) -> (4:w2731:refnum<k34>, 6:w2730:string, 15:w2729:errorcluster)  [unwired: 1 in, 1 out]
                        n1683 = TDMS Write(0:w2731, 5:w2730, 7:w2728, 9:w2727, 11:w2729) -> (4:w2726:refnum<k34>, 6:w2725:string, 15:w2724:errorcluster)  [unwired: 1 in, 1 out]
                        n1684 = TDMS Write(0:w2726, 5:w2725, 7:w2723, 9:w2722, 11:w2724) -> (15:w2721:errorcluster)  [unwired: 1 in, 3 out]
                        n1685 = local write "data file error"(w2721) -> ()
                      }
                    }
                  }
                  frame #6 {
                    # "LAB04-1"
                    n1686 = case shown="True" w2765 {
                      frame False {
                      }
                      frame True {
                        n1687 = local read "DISP LAB04-1"() -> (w2807:T4)
                        n1688 = local read "SIG LAB04-1"() -> (w2808:T2)
                        n1689 = local read "TDMS LAB04-1"() -> (w2809:refnum<k34>)
                        n1690 = Build Array("TEMP Neut") -> (w2773:string[])
                        n1691 = Build Array("CYCLE") -> (w2768:string[])
                        n1692 = Build Array("TEMP Live") -> (w2778:string[])
                        n1693 = Build Array("PF") -> (w2783:string[])
                        n1694 = Build Array("AMPS") -> (w2804:string[])
                        n1695 = Build Array("VOLTS") -> (w2795:string[])
                        n1696 = Unbundle(w2808) -> ("AMPS"=w2803:dbl, "VOLTS"=w2792:dbl, "PF"=w2791:dbl, "Tmp Live"=w2790:dbl, "Tmp Neut"=w2793:dbl)
                        n1697 = Unbundle(w2807) -> ("CYCLE"=w2788:dbl)  [unwired: 2 out]
                        n1698 = Build Array(w2792) -> (w2789:dbl[])
                        n1699 = Build Array(w2791) -> (w2782:dbl[])
                        n1700 = Build Array(w2790) -> (w2777:dbl[])
                        n1701 = Build Array(w2793) -> (w2772:dbl[])
                        n1702 = Build Array(w2803) -> (w2802:dbl[])
                        n1703 = Build Array(w2788) -> (w2767:dbl[])
                        n1704 = TDMS Write(0:w2809, 5:"LAB04-1 TEST VALUES", 7:w2804, 9:w2802) -> (4:w2797:refnum<k34>, 6:w2796:string, 15:w2784:errorcluster)  [unwired: 2 in, 1 out]
                        n1705 = TDMS Write(0:w2797, 5:w2796, 7:w2795, 9:w2789, 11:w2784) -> (4:w2787:refnum<k34>, 6:w2786:string, 15:w2785:errorcluster)  [unwired: 1 in, 1 out]
                        n1706 = TDMS Write(0:w2787, 5:w2786, 7:w2783, 9:w2782, 11:w2785) -> (4:w2781:refnum<k34>, 6:w2780:string, 15:w2779:errorcluster)  [unwired: 1 in, 1 out]
                        n1707 = TDMS Write(0:w2781, 5:w2780, 7:w2778, 9:w2777, 11:w2779) -> (4:w2776:refnum<k34>, 6:w2775:string, 15:w2774:errorcluster)  [unwired: 1 in, 1 out]
                        n1708 = TDMS Write(0:w2776, 5:w2775, 7:w2773, 9:w2772, 11:w2774) -> (4:w2771:refnum<k34>, 6:w2770:string, 15:w2769:errorcluster)  [unwired: 1 in, 1 out]
                        n1709 = TDMS Write(0:w2771, 5:w2770, 7:w2768, 9:w2767, 11:w2769) -> (15:w2766:errorcluster)  [unwired: 1 in, 3 out]
                        n1710 = local write "data file error"(w2766) -> ()
                      }
                    }
                  }
                  frame #7 {
                    # "LAB04-2"
                    n1711 = case shown="True" w2810 {
                      frame False {
                      }
                      frame True {
                        n1712 = local read "DISP LAB04-2"() -> (w2852:T4)
                        n1713 = local read "SIG LAB04-2"() -> (w2853:T2)
                        n1714 = local read "TDMS LAB04-2"() -> (w2854:refnum<k34>)
                        n1715 = Build Array("TEMP Neut") -> (w2818:string[])
                        n1716 = Build Array("CYCLE") -> (w2813:string[])
                        n1717 = Build Array("TEMP Live") -> (w2823:string[])
                        n1718 = Build Array("PF") -> (w2828:string[])
                        n1719 = Build Array("AMPS") -> (w2849:string[])
                        n1720 = Build Array("VOLTS") -> (w2840:string[])
                        n1721 = Unbundle(w2853) -> ("AMPS"=w2848:dbl, "VOLTS"=w2837:dbl, "PF"=w2836:dbl, "Tmp Live"=w2835:dbl, "Tmp Neut"=w2838:dbl)
                        n1722 = Unbundle(w2852) -> ("CYCLE"=w2833:dbl)  [unwired: 2 out]
                        n1723 = Build Array(w2837) -> (w2834:dbl[])
                        n1724 = Build Array(w2836) -> (w2827:dbl[])
                        n1725 = Build Array(w2835) -> (w2822:dbl[])
                        n1726 = Build Array(w2838) -> (w2817:dbl[])
                        n1727 = Build Array(w2848) -> (w2847:dbl[])
                        n1728 = Build Array(w2833) -> (w2812:dbl[])
                        n1729 = TDMS Write(0:w2854, 5:"LAB04-2 TEST VALUES", 7:w2849, 9:w2847) -> (4:w2842:refnum<k34>, 6:w2841:string, 15:w2829:errorcluster)  [unwired: 2 in, 1 out]
                        n1730 = TDMS Write(0:w2842, 5:w2841, 7:w2840, 9:w2834, 11:w2829) -> (4:w2832:refnum<k34>, 6:w2831:string, 15:w2830:errorcluster)  [unwired: 1 in, 1 out]
                        n1731 = TDMS Write(0:w2832, 5:w2831, 7:w2828, 9:w2827, 11:w2830) -> (4:w2826:refnum<k34>, 6:w2825:string, 15:w2824:errorcluster)  [unwired: 1 in, 1 out]
                        n1732 = TDMS Write(0:w2826, 5:w2825, 7:w2823, 9:w2822, 11:w2824) -> (4:w2821:refnum<k34>, 6:w2820:string, 15:w2819:errorcluster)  [unwired: 1 in, 1 out]
                        n1733 = TDMS Write(0:w2821, 5:w2820, 7:w2818, 9:w2817, 11:w2819) -> (4:w2816:refnum<k34>, 6:w2815:string, 15:w2814:errorcluster)  [unwired: 1 in, 1 out]
                        n1734 = TDMS Write(0:w2816, 5:w2815, 7:w2813, 9:w2812, 11:w2814) -> (15:w2811:errorcluster)  [unwired: 1 in, 3 out]
                        n1735 = local write "data file error"(w2811) -> ()
                      }
                    }
                  }
                  frame #8 {
                    # "LAB05-1"
                    n1736 = case shown="True" w2855 {
                      frame False {
                      }
                      frame True {
                        n1737 = local read "DISP LAB05-1"() -> (w2897:T4)
                        n1738 = local read "SIG LAB05-1"() -> (w2898:T2)
                        n1739 = local read "TDMS LAB05-1"() -> (w2899:refnum<k34>)
                        n1740 = Build Array("TEMP Neut") -> (w2863:string[])
                        n1741 = Build Array("CYCLE") -> (w2858:string[])
                        n1742 = Build Array("TEMP Live") -> (w2868:string[])
                        n1743 = Build Array("PF") -> (w2873:string[])
                        n1744 = Build Array("AMPS") -> (w2894:string[])
                        n1745 = Build Array("VOLTS") -> (w2885:string[])
                        n1746 = Unbundle(w2898) -> ("AMPS"=w2893:dbl, "VOLTS"=w2882:dbl, "PF"=w2881:dbl, "Tmp Live"=w2880:dbl, "Tmp Neut"=w2883:dbl)
                        n1747 = Unbundle(w2897) -> ("CYCLE"=w2878:dbl)  [unwired: 2 out]
                        n1748 = Build Array(w2882) -> (w2879:dbl[])
                        n1749 = Build Array(w2881) -> (w2872:dbl[])
                        n1750 = Build Array(w2880) -> (w2867:dbl[])
                        n1751 = Build Array(w2883) -> (w2862:dbl[])
                        n1752 = Build Array(w2893) -> (w2892:dbl[])
                        n1753 = Build Array(w2878) -> (w2857:dbl[])
                        n1754 = TDMS Write(0:w2899, 5:"LAB05-1 TEST VALUES", 7:w2894, 9:w2892) -> (4:w2887:refnum<k34>, 6:w2886:string, 15:w2874:errorcluster)  [unwired: 2 in, 1 out]
                        n1755 = TDMS Write(0:w2887, 5:w2886, 7:w2885, 9:w2879, 11:w2874) -> (4:w2877:refnum<k34>, 6:w2876:string, 15:w2875:errorcluster)  [unwired: 1 in, 1 out]
                        n1756 = TDMS Write(0:w2877, 5:w2876, 7:w2873, 9:w2872, 11:w2875) -> (4:w2871:refnum<k34>, 6:w2870:string, 15:w2869:errorcluster)  [unwired: 1 in, 1 out]
                        n1757 = TDMS Write(0:w2871, 5:w2870, 7:w2868, 9:w2867, 11:w2869) -> (4:w2866:refnum<k34>, 6:w2865:string, 15:w2864:errorcluster)  [unwired: 1 in, 1 out]
                        n1758 = TDMS Write(0:w2866, 5:w2865, 7:w2863, 9:w2862, 11:w2864) -> (4:w2861:refnum<k34>, 6:w2860:string, 15:w2859:errorcluster)  [unwired: 1 in, 1 out]
                        n1759 = TDMS Write(0:w2861, 5:w2860, 7:w2858, 9:w2857, 11:w2859) -> (15:w2856:errorcluster)  [unwired: 1 in, 3 out]
                        n1760 = local write "data file error"(w2856) -> ()
                      }
                    }
                  }
                  frame #9 {
                    # "LAB05-2"
                    n1761 = case shown="True" w2900 {
                      frame False {
                      }
                      frame True {
                        n1762 = local read "DISP LAB05-2"() -> (w2942:T4)
                        n1763 = local read "SIG LAB05-2"() -> (w2943:T2)
                        n1764 = local read "TDMS LAB05-2"() -> (w2944:refnum<k34>)
                        n1765 = Build Array("TEMP Neut") -> (w2908:string[])
                        n1766 = Build Array("CYCLE") -> (w2903:string[])
                        n1767 = Build Array("TEMP Live") -> (w2913:string[])
                        n1768 = Build Array("PF") -> (w2918:string[])
                        n1769 = Build Array("AMPS") -> (w2939:string[])
                        n1770 = Build Array("VOLTS") -> (w2930:string[])
                        n1771 = Unbundle(w2943) -> ("AMPS"=w2938:dbl, "VOLTS"=w2927:dbl, "PF"=w2926:dbl, "Tmp Live"=w2925:dbl, "Tmp Neut"=w2928:dbl)
                        n1772 = Unbundle(w2942) -> ("CYCLE"=w2923:dbl)  [unwired: 2 out]
                        n1773 = Build Array(w2927) -> (w2924:dbl[])
                        n1774 = Build Array(w2926) -> (w2917:dbl[])
                        n1775 = Build Array(w2925) -> (w2912:dbl[])
                        n1776 = Build Array(w2928) -> (w2907:dbl[])
                        n1777 = Build Array(w2938) -> (w2937:dbl[])
                        n1778 = Build Array(w2923) -> (w2902:dbl[])
                        n1779 = TDMS Write(0:w2944, 5:"LAB05-2 TEST VALUES", 7:w2939, 9:w2937) -> (4:w2932:refnum<k34>, 6:w2931:string, 15:w2919:errorcluster)  [unwired: 2 in, 1 out]
                        n1780 = TDMS Write(0:w2932, 5:w2931, 7:w2930, 9:w2924, 11:w2919) -> (4:w2922:refnum<k34>, 6:w2921:string, 15:w2920:errorcluster)  [unwired: 1 in, 1 out]
                        n1781 = TDMS Write(0:w2922, 5:w2921, 7:w2918, 9:w2917, 11:w2920) -> (4:w2916:refnum<k34>, 6:w2915:string, 15:w2914:errorcluster)  [unwired: 1 in, 1 out]
                        n1782 = TDMS Write(0:w2916, 5:w2915, 7:w2913, 9:w2912, 11:w2914) -> (4:w2911:refnum<k34>, 6:w2910:string, 15:w2909:errorcluster)  [unwired: 1 in, 1 out]
                        n1783 = TDMS Write(0:w2911, 5:w2910, 7:w2908, 9:w2907, 11:w2909) -> (4:w2906:refnum<k34>, 6:w2905:string, 15:w2904:errorcluster)  [unwired: 1 in, 1 out]
                        n1784 = TDMS Write(0:w2906, 5:w2905, 7:w2903, 9:w2902, 11:w2904) -> (15:w2901:errorcluster)  [unwired: 1 in, 3 out]
                        n1785 = local write "data file error"(w2901) -> ()
                      }
                    }
                  }
                }
              }
            }
          }
          frame #12 {
            # "check for amps fail"
            # "check for cycle test & temperature rise fail conditions"
            n1786 = local read "on loops"() -> (w2970:dbl)
            n1787 = local read "jig cycle"() -> (w2967:dbl)
            n1788 = local read "jig cycle"() -> (w2972:dbl)
            n1789 = Add(x=w2970, y=3.0) -> (x+y=w2968:dbl)
            n1790 = Equal?(x=w2967, y=w2968) -> (x = y?=w2963:bool)
            n1791 = Equal?(x=w2972, y=1.0) -> (x = y?=w2965:bool)
            n1792 = stacked-sequence {
              tunnel: w2966 -> [w2975 _ _ _ _ _ _ _ _ _]
              tunnel: w2965 -> [w2976 w2995 w3014 w3033 w3052 w3071 w3090 w3109 w3128 w3147]
              tunnel: w2964 -> [w2973 _ _ _ _ _ _ _ _ _]
              tunnel: w2963 -> [w2974 w2994 w3013 w3032 w3051 w3070 w3089 w3108 w3127 w3146]
              tunnel: w2962 -> [_ w2993 _ _ _ _ _ _ _ _]
              tunnel: w2961 -> [_ w2992 _ _ _ _ _ _ _ _]
              tunnel: w2960 -> [_ _ w3012 _ _ _ _ _ _ _]
              tunnel: w2959 -> [_ _ w3011 _ _ _ _ _ _ _]
              tunnel: w2958 -> [_ _ _ w3031 _ _ _ _ _ _]
              tunnel: w2957 -> [_ _ _ w3030 _ _ _ _ _ _]
              tunnel: w2956 -> [_ _ _ _ w3050 _ _ _ _ _]
              tunnel: w2955 -> [_ _ _ _ w3049 _ _ _ _ _]
              tunnel: w2954 -> [_ _ _ _ _ w3069 _ _ _ _]
              tunnel: w2953 -> [_ _ _ _ _ w3068 _ _ _ _]
              tunnel: w2952 -> [_ _ _ _ _ _ w3088 _ _ _]
              tunnel: w2951 -> [_ _ _ _ _ _ w3087 _ _ _]
              tunnel: w2950 -> [_ _ _ _ _ _ _ w3107 _ _]
              tunnel: w2949 -> [_ _ _ _ _ _ _ w3106 _ _]
              tunnel: w2948 -> [_ _ _ _ _ _ _ _ w3126 _]
              tunnel: w2947 -> [_ _ _ _ _ _ _ _ w3125 _]
              tunnel: w2946 -> [_ _ _ _ _ _ _ _ _ w3145]
              tunnel: w2945 -> [_ _ _ _ _ _ _ _ _ w3144]
              frame #0 {
                # "LAB01-1"
                n1793 = case shown="True" w2973 {
                  tunnel: w2976 -> [_ w2988]
                  tunnel: w2975 -> [_ w2985]
                  tunnel: w2974 -> [_ w2984]
                  frame False {
                  }
                  frame True {
                    n1794 = local read "TEMP START LAB01-1"() -> (w2990:cluster{"TL":dbl, "TN":dbl})
                    n1795 = local read "RESULT LAB01-1"() -> (w2977:bool)
                    n1796 = local read "FAIL LAB01-1"() -> (w2981:cluster{"LO":dbl, "HI":dbl})
                    n1797 = local read "TDMS LAB01-1"() -> (w2989:refnum<k34>)
                    n1798 = local read "SET LAB01-1"() -> (w2986:T5)
                    n1799 = local read "DISP LAB01-1"() -> (w2987:T4)
                    n1800 = local read "SIG LAB01-1"() -> (w2991:T2)
                    n1801 = Bundle("FAIL LAB01-1"=w2981, "SIG LAB01-1"=w2991, "TEMP START LAB01-1"=w2990, "DISP LAB01-1"=w2987, "SET LAB01-1"=w2986, "TDMS LAB01-1"=w2989) -> (w2979:T25)  [unwired: 1 in]
                    n1802 = call "sub vi - cycle&temp fail v5.vi"("Amps Lo?"=w2988, "Input Cluster"=w2979, "SELECT"=w2985, "Amps Hi?"=w2984, "Result In"=w2977) -> ("(FAIL) out"=w2980:cluster{"FAIL LO":dbl, "FAIL HI":dbl}, "(DISP) out"=w2983:T4, "Result Out"=w2978:bool, "file error"=w2982:errorcluster)  [unwired: 11 in]
                    n1803 = local write "FAIL LAB01-1"(w2980) -> ()
                    n1804 = local write "DISP LAB01-1"(w2983) -> ()
                    n1805 = local write "RESULT LAB01-1"(w2978) -> ()
                    n1806 = local write "data file error"(w2982) -> ()
                  }
                }
              }
              frame #1 {
                # "LAB01-2"
                n1807 = case shown="True" w2993 {
                  tunnel: w2995 -> [_ w3007]
                  tunnel: w2992 -> [_ w3004]
                  tunnel: w2994 -> [_ w3003]
                  frame False {
                  }
                  frame True {
                    n1808 = local read "TEMP START LAB01-2"() -> (w3009:cluster{"TL":dbl, "TN":dbl})
                    n1809 = local read "FAIL LAB01-2"() -> (w3000:cluster{"LO":dbl, "HI":dbl})
                    n1810 = local read "TDMS LAB01-2"() -> (w3008:refnum<k34>)
                    n1811 = local read "SET LAB01-2"() -> (w3005:T5)
                    n1812 = local read "DISP LAB01-2"() -> (w3006:T4)
                    n1813 = local read "RESULT LAB01-2"() -> (w2996:bool)
                    n1814 = local read "SIG LAB01-2"() -> (w3010:T2)
                    n1815 = Bundle("FAIL LAB01-2"=w3000, "SIG LAB01-2"=w3010, "TEMP START LAB01-2"=w3009, "DISP LAB01-2"=w3006, "SET LAB01-2"=w3005, "TDMS LAB01-2"=w3008) -> (w2998:T26)  [unwired: 1 in]
                    n1816 = call "sub vi - cycle&temp fail v5.vi"("Amps Lo?"=w3007, "Input Cluster"=w2998, "SELECT"=w3004, "Amps Hi?"=w3003, "Result In"=w2996) -> ("(FAIL) out"=w2999:cluster{"FAIL LO":dbl, "FAIL HI":dbl}, "(DISP) out"=w3002:T4, "Result Out"=w2997:bool, "file error"=w3001:errorcluster)  [unwired: 11 in]
                    n1817 = local write "FAIL LAB01-2"(w2999) -> ()
                    n1818 = local write "DISP LAB01-2"(w3002) -> ()
                    n1819 = local write "RESULT LAB01-2"(w2997) -> ()
                    n1820 = local write "data file error"(w3001) -> ()
                  }
                }
              }
              frame #2 {
                # "LAB02-1"
                n1821 = case shown="True" w3012 {
                  tunnel: w3014 -> [_ w3026]
                  tunnel: w3011 -> [_ w3023]
                  tunnel: w3013 -> [_ w3022]
                  frame False {
                  }
                  frame True {
                    n1822 = local read "TEMP START LAB02-1"() -> (w3028:cluster{"TL":dbl, "TN":dbl})
                    n1823 = local read "FAIL LAB02-1"() -> (w3019:cluster{"LO":dbl, "HI":dbl})
                    n1824 = local read "TDMS LAB02-1"() -> (w3027:refnum<k34>)
                    n1825 = local read "SET LAB02-1"() -> (w3024:T5)
                    n1826 = local read "DISP LAB02-1"() -> (w3025:T4)
                    n1827 = local read "SIG LAB02-1"() -> (w3029:T2)
                    n1828 = local read "RESULT LAB02-1"() -> (w3015:bool)
                    n1829 = Bundle("FAIL LAB02-1"=w3019, "SIG LAB02-1"=w3029, "TEMP START LAB02-1"=w3028, "DISP LAB02-1"=w3025, "SET LAB02-1"=w3024, "TDMS LAB02-1"=w3027) -> (w3017:T27)  [unwired: 1 in]
                    n1830 = call "sub vi - cycle&temp fail v5.vi"("Amps Lo?"=w3026, "Input Cluster"=w3017, "SELECT"=w3023, "Amps Hi?"=w3022, "Result In"=w3015) -> ("(FAIL) out"=w3018:cluster{"FAIL LO":dbl, "FAIL HI":dbl}, "(DISP) out"=w3021:T4, "Result Out"=w3016:bool, "file error"=w3020:errorcluster)  [unwired: 11 in]
                    n1831 = local write "FAIL LAB02-1"(w3018) -> ()
                    n1832 = local write "DISP LAB02-1"(w3021) -> ()
                    n1833 = local write "RESULT LAB02-1"(w3016) -> ()
                    n1834 = local write "data file error"(w3020) -> ()
                  }
                }
              }
              frame #3 {
                # "LAB02-2"
                n1835 = case shown="True" w3031 {
                  tunnel: w3033 -> [_ w3045]
                  tunnel: w3030 -> [_ w3042]
                  tunnel: w3032 -> [_ w3041]
                  frame False {
                  }
                  frame True {
                    n1836 = local read "TEMP START LAB02-2"() -> (w3047:cluster{"TL":dbl, "TN":dbl})
                    n1837 = local read "FAIL LAB02-2"() -> (w3038:cluster{"LO":dbl, "HI":dbl})
                    n1838 = local read "TDMS LAB02-2"() -> (w3046:refnum<k34>)
                    n1839 = local read "SET LAB02-2"() -> (w3043:T5)
                    n1840 = local read "DISP LAB02-2"() -> (w3044:T4)
                    n1841 = local read "SIG LAB02-2"() -> (w3048:T2)
                    n1842 = local read "RESULT LAB02-2"() -> (w3034:bool)
                    n1843 = Bundle("FAIL LAB02-2"=w3038, "SIG LAB02-2"=w3048, "TEMP START LAB02-2"=w3047, "DISP LAB02-2"=w3044, "SET LAB02-2"=w3043, "TDMS LAB02-2"=w3046) -> (w3036:T28)  [unwired: 1 in]
                    n1844 = call "sub vi - cycle&temp fail v5.vi"("Amps Lo?"=w3045, "Input Cluster"=w3036, "SELECT"=w3042, "Amps Hi?"=w3041, "Result In"=w3034) -> ("(FAIL) out"=w3037:cluster{"FAIL LO":dbl, "FAIL HI":dbl}, "(DISP) out"=w3040:T4, "Result Out"=w3035:bool, "file error"=w3039:errorcluster)  [unwired: 11 in]
                    n1845 = local write "FAIL LAB02-2"(w3037) -> ()
                    n1846 = local write "DISP LAB02-2"(w3040) -> ()
                    n1847 = local write "RESULT LAB02-2"(w3035) -> ()
                    n1848 = local write "data file error"(w3039) -> ()
                  }
                }
              }
              frame #4 {
                # "LAB03-1"
                n1849 = case shown="True" w3050 {
                  tunnel: w3052 -> [_ w3064]
                  tunnel: w3049 -> [_ w3061]
                  tunnel: w3051 -> [_ w3060]
                  frame False {
                  }
                  frame True {
                    n1850 = local read "TEMP START LAB03-1"() -> (w3066:cluster{"TL":dbl, "TN":dbl})
                    n1851 = local read "FAIL LAB03-1"() -> (w3057:cluster{"LO":dbl, "HI":dbl})
                    n1852 = local read "TDMS LAB03-1"() -> (w3065:refnum<k34>)
                    n1853 = local read "SET LAB03-1"() -> (w3062:T5)
                    n1854 = local read "DISP LAB03-1"() -> (w3063:T4)
                    n1855 = local read "SIG LAB03-1"() -> (w3067:T2)
                    n1856 = local read "RESULT LAB03-1"() -> (w3053:bool)
                    n1857 = Bundle("FAIL LAB03-1"=w3057, "SIG LAB03-1"=w3067, "TEMP START LAB03-1"=w3066, "DISP LAB03-1"=w3063, "SET LAB03-1"=w3062, "TDMS LAB03-1"=w3065) -> (w3055:T29)  [unwired: 1 in]
                    n1858 = call "sub vi - cycle&temp fail v5.vi"("Amps Lo?"=w3064, "Input Cluster"=w3055, "SELECT"=w3061, "Amps Hi?"=w3060, "Result In"=w3053) -> ("(FAIL) out"=w3056:cluster{"FAIL LO":dbl, "FAIL HI":dbl}, "(DISP) out"=w3059:T4, "Result Out"=w3054:bool, "file error"=w3058:errorcluster)  [unwired: 11 in]
                    n1859 = local write "FAIL LAB03-1"(w3056) -> ()
                    n1860 = local write "DISP LAB03-1"(w3059) -> ()
                    n1861 = local write "RESULT LAB03-1"(w3054) -> ()
                    n1862 = local write "data file error"(w3058) -> ()
                  }
                }
              }
              frame #5 {
                # "LAB03-2"
                n1863 = case shown="True" w3069 {
                  tunnel: w3071 -> [_ w3083]
                  tunnel: w3068 -> [_ w3080]
                  tunnel: w3070 -> [_ w3079]
                  frame False {
                  }
                  frame True {
                    n1864 = local read "TEMP START LAB03-2"() -> (w3085:cluster{"TL":dbl, "TN":dbl})
                    n1865 = local read "FAIL LAB03-2"() -> (w3076:cluster{"LO":dbl, "HI":dbl})
                    n1866 = local read "TDMS LAB03-2"() -> (w3084:refnum<k34>)
                    n1867 = local read "SET LAB03-2"() -> (w3081:T5)
                    n1868 = local read "DISP LAB03-2"() -> (w3082:T4)
                    n1869 = local read "RESULT LAB03-2"() -> (w3072:bool)
                    n1870 = local read "SIG LAB03-2"() -> (w3086:T2)
                    n1871 = Bundle("FAIL LAB03-2"=w3076, "SIG LAB03-2"=w3086, "TEMP START LAB03-2"=w3085, "DISP LAB03-2"=w3082, "SET LAB03-2"=w3081, "TDMS LAB03-2"=w3084) -> (w3074:T30)  [unwired: 1 in]
                    n1872 = call "sub vi - cycle&temp fail v5.vi"("Amps Lo?"=w3083, "Input Cluster"=w3074, "SELECT"=w3080, "Amps Hi?"=w3079, "Result In"=w3072) -> ("(FAIL) out"=w3075:cluster{"FAIL LO":dbl, "FAIL HI":dbl}, "(DISP) out"=w3078:T4, "Result Out"=w3073:bool, "file error"=w3077:errorcluster)  [unwired: 11 in]
                    n1873 = local write "FAIL LAB03-2"(w3075) -> ()
                    n1874 = local write "DISP LAB03-2"(w3078) -> ()
                    n1875 = local write "RESULT LAB03-2"(w3073) -> ()
                    n1876 = local write "data file error"(w3077) -> ()
                  }
                }
              }
              frame #6 {
                # "LAB04-1"
                n1877 = case shown="True" w3088 {
                  tunnel: w3090 -> [_ w3102]
                  tunnel: w3087 -> [_ w3099]
                  tunnel: w3089 -> [_ w3098]
                  frame False {
                  }
                  frame True {
                    n1878 = local read "TEMP START LAB04-1"() -> (w3104:cluster{"TL":dbl, "TN":dbl})
                    n1879 = local read "FAIL LAB04-1"() -> (w3095:cluster{"LO":dbl, "HI":dbl})
                    n1880 = local read "TDMS LAB04-1"() -> (w3103:refnum<k34>)
                    n1881 = local read "SET LAB04-1"() -> (w3100:T5)
                    n1882 = local read "DISP LAB04-1"() -> (w3101:T4)
                    n1883 = local read "SIG LAB04-1"() -> (w3105:T2)
                    n1884 = local read "RESULT LAB04-1"() -> (w3091:bool)
                    n1885 = Bundle("FAIL LAB04-1"=w3095, "SIG LAB04-1"=w3105, "TEMP START LAB04-1"=w3104, "DISP LAB04-1"=w3101, "SET LAB04-1"=w3100, "TDMS LAB04-1"=w3103) -> (w3093:T31)  [unwired: 1 in]
                    n1886 = call "sub vi - cycle&temp fail v5.vi"("Amps Lo?"=w3102, "Input Cluster"=w3093, "SELECT"=w3099, "Amps Hi?"=w3098, "Result In"=w3091) -> ("(FAIL) out"=w3094:cluster{"FAIL LO":dbl, "FAIL HI":dbl}, "(DISP) out"=w3097:T4, "Result Out"=w3092:bool, "file error"=w3096:errorcluster)  [unwired: 11 in]
                    n1887 = local write "FAIL LAB04-1"(w3094) -> ()
                    n1888 = local write "DISP LAB04-1"(w3097) -> ()
                    n1889 = local write "RESULT LAB04-1"(w3092) -> ()
                    n1890 = local write "data file error"(w3096) -> ()
                  }
                }
              }
              frame #7 {
                # "LAB04-2"
                n1891 = case shown="True" w3107 {
                  tunnel: w3109 -> [_ w3121]
                  tunnel: w3106 -> [_ w3118]
                  tunnel: w3108 -> [_ w3117]
                  frame False {
                  }
                  frame True {
                    n1892 = local read "TEMP START LAB04-2"() -> (w3123:cluster{"TL":dbl, "TN":dbl})
                    n1893 = local read "FAIL LAB04-2"() -> (w3114:cluster{"LO":dbl, "HI":dbl})
                    n1894 = local read "TDMS LAB04-2"() -> (w3122:refnum<k34>)
                    n1895 = local read "SET LAB04-2"() -> (w3119:T5)
                    n1896 = local read "DISP LAB04-2"() -> (w3120:T4)
                    n1897 = local read "SIG LAB04-2"() -> (w3124:T2)
                    n1898 = local read "RESULT LAB04-2"() -> (w3110:bool)
                    n1899 = Bundle("FAIL LAB04-2"=w3114, "SIG LAB04-2"=w3124, "TEMP START LAB04-2"=w3123, "DISP LAB04-2"=w3120, "SET LAB04-2"=w3119, "TDMS LAB04-2"=w3122) -> (w3112:T32)  [unwired: 1 in]
                    n1900 = call "sub vi - cycle&temp fail v5.vi"("Amps Lo?"=w3121, "Input Cluster"=w3112, "SELECT"=w3118, "Amps Hi?"=w3117, "Result In"=w3110) -> ("(FAIL) out"=w3113:cluster{"FAIL LO":dbl, "FAIL HI":dbl}, "(DISP) out"=w3116:T4, "Result Out"=w3111:bool, "file error"=w3115:errorcluster)  [unwired: 11 in]
                    n1901 = local write "FAIL LAB04-2"(w3113) -> ()
                    n1902 = local write "DISP LAB04-2"(w3116) -> ()
                    n1903 = local write "RESULT LAB04-2"(w3111) -> ()
                    n1904 = local write "data file error"(w3115) -> ()
                  }
                }
              }
              frame #8 {
                # "LAB05-1"
                n1905 = case shown="True" w3126 {
                  tunnel: w3128 -> [_ w3140]
                  tunnel: w3125 -> [_ w3137]
                  tunnel: w3127 -> [_ w3136]
                  frame False {
                  }
                  frame True {
                    n1906 = local read "TEMP START LAB05-1"() -> (w3142:cluster{"TL":dbl, "TN":dbl})
                    n1907 = local read "FAIL LAB05-1"() -> (w3133:cluster{"LO":dbl, "HI":dbl})
                    n1908 = local read "TDMS LAB05-1"() -> (w3141:refnum<k34>)
                    n1909 = local read "SET LAB05-1"() -> (w3138:T5)
                    n1910 = local read "DISP LAB05-1"() -> (w3139:T4)
                    n1911 = local read "SIG LAB05-1"() -> (w3143:T2)
                    n1912 = local read "RESULT LAB05-1"() -> (w3129:bool)
                    n1913 = Bundle("FAIL LAB05-1"=w3133, "SIG LAB05-1"=w3143, "TEMP START LAB05-1"=w3142, "DISP LAB05-1"=w3139, "SET LAB05-1"=w3138, "TDMS LAB05-1"=w3141) -> (w3131:T33)  [unwired: 1 in]
                    n1914 = call "sub vi - cycle&temp fail v5.vi"("Amps Lo?"=w3140, "Input Cluster"=w3131, "SELECT"=w3137, "Amps Hi?"=w3136, "Result In"=w3129) -> ("(FAIL) out"=w3132:cluster{"FAIL LO":dbl, "FAIL HI":dbl}, "(DISP) out"=w3135:T4, "Result Out"=w3130:bool, "file error"=w3134:errorcluster)  [unwired: 11 in]
                    n1915 = local write "FAIL LAB05-1"(w3132) -> ()
                    n1916 = local write "DISP LAB05-1"(w3135) -> ()
                    n1917 = local write "RESULT LAB05-1"(w3130) -> ()
                    n1918 = local write "data file error"(w3134) -> ()
                  }
                }
              }
              frame #9 {
                # "LAB05-2"
                n1919 = case shown="True" w3145 {
                  tunnel: w3147 -> [_ w3159]
                  tunnel: w3144 -> [_ w3156]
                  tunnel: w3146 -> [_ w3155]
                  frame False {
                  }
                  frame True {
                    n1920 = local read "TEMP START LAB05-2"() -> (w3161:cluster{"TL":dbl, "TN":dbl})
                    n1921 = local read "FAIL LAB05-2"() -> (w3152:cluster{"LO":dbl, "HI":dbl})
                    n1922 = local read "TDMS LAB05-2"() -> (w3160:refnum<k34>)
                    n1923 = local read "SET LAB05-2"() -> (w3157:T5)
                    n1924 = local read "DISP LAB05-2"() -> (w3158:T4)
                    n1925 = local read "SIG LAB05-2"() -> (w3162:T2)
                    n1926 = local read "RESULT LAB05-2"() -> (w3148:bool)
                    n1927 = Bundle("FAIL LAB05-2"=w3152, "SIG LAB05-2"=w3162, "TEMP START LAB05-2"=w3161, "DISP LAB05-2"=w3158, "SET LAB05-2"=w3157, "TDMS LAB05-2"=w3160) -> (w3150:T34)  [unwired: 1 in]
                    n1928 = call "sub vi - cycle&temp fail v5.vi"("Amps Lo?"=w3159, "Input Cluster"=w3150, "SELECT"=w3156, "Amps Hi?"=w3155, "Result In"=w3148) -> ("(FAIL) out"=w3151:cluster{"FAIL LO":dbl, "FAIL HI":dbl}, "(DISP) out"=w3154:T4, "Result Out"=w3149:bool, "file error"=w3153:errorcluster)  [unwired: 11 in]
                    n1929 = local write "FAIL LAB05-2"(w3151) -> ()
                    n1930 = local write "DISP LAB05-2"(w3154) -> ()
                    n1931 = local write "RESULT LAB05-2"(w3149) -> ()
                    n1932 = local write "data file error"(w3153) -> ()
                  }
                }
              }
            }
          }
          frame #13 {
            # "run calibration routine"
            n1933 = local read "CALIBRATE"() -> (w3163:bool)
            n1934 = case shown="True" w3163 {
              frame False {
              }
              frame True {
                n1935 = stacked-sequence {
                  seq-local: [w3164 _ _] -> [_ w3166 _]
                  frame #0 {
                    n1936 = call "CALIBRATION PASSWORD"() -> ("PASSWORD"=w3164:string)  [unwired: 17 in, 2 out]
                  }
                  frame #1 {
                    n1937 = Equal?(x=w3166, y="7777") -> (x = y?=w3165:bool)
                    n1938 = case shown="True" w3165 {
                      frame False {
                      }
                      frame True {
                        n1939 = stacked-sequence {
                          frame #0 {
                            n1940 = call "sub vi - calibration v1.vi"() -> ()  [unwired: 12 in]
                          }
                          frame #1 {
                            n1941 = call "sub vi - get calibration values v1.vi"() -> ("LAB01 (CAL)"=w3172:T6, "LAB02 (CAL)"=w3171:T7, "LAB03 (CAL)"=w3170:T6, "LAB04 (CAL)"=w3169:T6, "calibration file error out"=w3173:errorcluster, "LAB05 (CAL)"=w3168:T6)  [unwired: 10 in]
                            n1942 = local write "calibration file error out"(w3173) -> ()
                            n1943 = local write "CAL LAB04"(w3169) -> ()
                            n1944 = local write "CAL LAB05"(w3168) -> ()
                            n1945 = local write "CAL LAB01"(w3172) -> ()
                            n1946 = local write "CAL LAB02"(w3171) -> ()
                            n1947 = local write "CAL LAB03"(w3170) -> ()
                          }
                        }
                      }
                    }
                  }
                  frame #2 {
                    n1948 = local write "CALIBRATE"(FALSE) -> ()
                  }
                }
              }
            }
          }
          frame #14 {
            # "save certain settings to file"
            n1949 = String To Path(string="c:\\crabtree\\Set Up\\") -> (path=w3176:path)
            n1950 = Build Path(base path=w3176, name or relative path="settings.bin") -> (appended path=w3178:path)
            n1951 = Build Path(base path=w3176, name or relative path="mail.bin") -> (appended path=w3175:path)
            n1952 = Create Folder(path (use dialog)=w3176) -> (error out=w3181:errorcluster)  [unwired: 2 in, 2 out]
            n1953 = call <vilib>:"Clear Errors.vi"("error in (no error)"=w3181) -> ()  [unwired: 6 in, 1 out]
            n1954 = stacked-sequence {
              seq-local: [w3182 _] -> [_ w3195]
              tunnel: w3178 -> [_ w3196]
              tunnel: w3175 -> [_ w3194]
              frame #0 {
                n1955 = local read "Network Directory"() -> (w3187:path)
                n1956 = local read "SET LAB05-2"() -> (w3186:T5)
                n1957 = local read "SET LAB05-1"() -> (w3185:T5)
                n1958 = local read "SET LAB04-2"() -> (w3184:T5)
                n1959 = local read "SET LAB03-2"() -> (w3188:T5)
                n1960 = local read "SET LAB04-1"() -> (w3183:T5)
                n1961 = local read "SET LAB03-1"() -> (w3189:T5)
                n1962 = local read "SET LAB02-2"() -> (w3190:T5)
                n1963 = local read "SET LAB02-1"() -> (w3191:T5)
                n1964 = local read "SET LAB01-2"() -> (w3192:T5)
                n1965 = local read "SET LAB01-1"() -> (w3193:T5)
                n1966 = Bundle("SET LAB01-1"=w3193, "SET LAB01-2"=w3192, "SET LAB02-1"=w3191, "SET LAB02-2"=w3190, "SET LAB03-1"=w3189, "SET LAB03-2"=w3188, "SET LAB04-1"=w3183, "SET LAB04-2"=w3184, "SET LAB05-1"=w3185, "SET LAB05-2"=w3186, "Network Directory"=w3187) -> (w3182:T17)  [unwired: 1 in]
              }
              frame #1 {
                n1967 = event shown="[2] \"MAIL SETTINGS.OUT SERVER ADDRESS\", \"MAIL SETTINGS.FROM ACCOUNT\", \"MAIL SETTINGS.USER NAME\", \"MAIL SELECT\", \"MAIL SETTINGS.PASSWORD\": Value Change" {
                  selector: _ -> [_ _ _]
                  dyn-events: _ -> [_ _ _]
                  timeout: 10.0 -> [_ _ _]
                  tunnel: w3196 -> [_ w3198 _]
                  tunnel: w3195 -> [_ w3199 _]
                  tunnel: w3194 -> [_ _ w3209]
                  event Timeout {
                    n1968 = event-data() -> ()  [unwired: 1 in, 3 out]
                  }
                  event "SET LAB01-1", "SET LAB01-2", "SET LAB02-1", "SET LAB02-2", "SET LAB03-1", "SET LAB03-2", "SET LAB04-1", "SET LAB04-2", "SET LAB05-1", "SET LAB05-2", "Network Directory": Value Change {
                    n1969 = event-data() -> ()  [unwired: 1 in, 6 out]
                    n1970 = Open/Create/Replace File(file path (use dialog)=w3198, operation (0:open)=T16."replace or create") -> (refnum out=w3204:refnum<file>, error out=w3203:errorcluster)  [unwired: 4 in, 1 out]
                    n1971 = Write to Binary File(file (use dialog)=w3204, data=w3199, error in=w3203) -> (refnum out=w3202:refnum<file>, error out=w3201:errorcluster)  [unwired: 3 in, 1 out]
                    n1972 = Close File(refnum=w3202, error in=w3201) -> (error out=w3200:errorcluster)  [unwired: 1 out]
                    n1973 = local write "data file error"(w3200) -> ()
                  }
                  event "MAIL SETTINGS.OUT SERVER ADDRESS", "MAIL SETTINGS.FROM ACCOUNT", "MAIL SETTINGS.USER NAME", "MAIL SELECT", "MAIL SETTINGS.PASSWORD": Value Change {
                    n1974 = event-data() -> ()  [unwired: 1 in, 6 out]
                    n1975 = local read "MAIL SETTINGS"() -> (w3208:T8)
                    n1976 = local read "MAIL SELECT"() -> (w3206:cluster{"Mail Notification":bool, "TO:":string})
                    n1977 = Open/Create/Replace File(file path (use dialog)=w3209, operation (0:open)=T16."replace or create") -> (refnum out=w3214:refnum<file>, error out=w3213:errorcluster)  [unwired: 4 in, 1 out]
                    n1978 = Bundle("MAIL SETTINGS"=w3208, "MAIL SELECT"=w3206) -> (w3207:T18)  [unwired: 1 in]
                    n1979 = Write to Binary File(file (use dialog)=w3214, data=w3207, error in=w3213) -> (refnum out=w3212:refnum<file>, error out=w3211:errorcluster)  [unwired: 3 in, 1 out]
                    n1980 = Close File(refnum=w3212, error in=w3211) -> (error out=w3210:errorcluster)  [unwired: 1 out]
                    n1981 = local write "data file error"(w3210) -> ()
                  }
                }
              }
            }
          }
          frame #15 {
            # "mail control"
            n1982 = local read "MAIL SETTINGS"() -> (w3231:T8)
            n1983 = local read "MAIL SELECT"() -> (w3232:cluster{"Mail Notification":bool, "TO:":string})
            n1984 = Unbundle(w3231) -> ("OUT SERVER ADDRESS"=w3230:string, "FROM ACCOUNT"=w3229:string, "TEST MAIL"=w3228:bool)  [unwired: 4 out]
            n1985 = Unbundle(w3232) -> ("Mail Notification"=w3226:bool, "TO:"=w3227:string)
            n1986 = stacked-sequence {
              tunnel: w3227 -> [w3237 w3271]
              tunnel: w3231 -> [w3236 w3270]
              tunnel: w3230 -> [w3235 w3269]
              tunnel: w3229 -> [w3234 w3268]
              tunnel: w3228 -> [w3233 _]
              tunnel: w3226 -> [_ w3267]
              tunnel: w3225 -> [_ w3266]
              tunnel: w3224 -> [_ w3265]
              tunnel: w3223 -> [_ w3264]
              tunnel: w3222 -> [_ w3263]
              tunnel: w3221 -> [_ w3262]
              tunnel: w3220 -> [_ w3261]
              tunnel: w3219 -> [_ w3260]
              tunnel: w3218 -> [_ w3259]
              tunnel: w3217 -> [_ w3258]
              tunnel: w3216 -> [_ w3257]
              frame #0 {
                # "mail test"
                n1987 = case shown="True" w3233 {
                  tunnel: w3236 -> [_ w3241]
                  tunnel: w3237 -> [_ w3240]
                  tunnel: w3235 -> [_ w3239]
                  tunnel: w3234 -> [_ w3238]
                  frame False {
                  }
                  frame True {
                    n1988 = stacked-sequence {
                      seq-local: [_ _ w3247 _] -> [_ _ _ w3252]
                      tunnel: w3241 -> [w3244 _ _ w3256]
                      tunnel: w3240 -> [_ _ w3251 _]
                      tunnel: w3239 -> [_ _ w3250 _]
                      tunnel: w3238 -> [_ _ w3249 _]
                      frame #0 {
                        n1989 = Bundle(cluster=w3244, "TEST MAIL STATUS"="TEST START") -> (w3242:T8)  [unwired: 6 in]
                        n1990 = local write "MAIL SETTINGS"(w3242) -> ()
                      }
                      frame #1 {
                        n1991 = Wait (ms)(milliseconds to wait=500) -> ()  [unwired: 1 out]
                      }
                      frame #2 {
                        n1992 = call "sub vi - send mail v3.vi"("TO:"=w3251, "message"="", "subject"="MAIL TEST FROM LAB PANEL", "out going server"=w3250, "from"=w3249) -> ("error out"=w3247:errorcluster)  [unwired: 10 in]
                      }
                      frame #3 {
                        n1993 = Bundle(cluster=w3256, "TEST MAIL"=FALSE, "TEST MAIL STATUS"="TEST END", "mail error"=w3252) -> (w3254:T8)  [unwired: 4 in]
                        n1994 = local write "MAIL SETTINGS"(w3254) -> ()
                      }
                    }
                  }
                }
              }
              frame #1 {
                # "mail report"
                n1995 = stacked-sequence {
                  seq-local: [w3276 _ _] -> [_ _ w3456]
                  seq-local: [_ w3373 _] -> [_ _ w3445]
                  tunnel: w3271 -> [_ _ w3457]
                  tunnel: w3270 -> [_ _ _]
                  tunnel: w3269 -> [_ _ w3454]
                  tunnel: w3268 -> [_ _ w3453]
                  tunnel: w3267 -> [_ _ w3447]
                  tunnel: w3266 -> [_ w3403 _]
                  tunnel: w3265 -> [_ w3400 _]
                  tunnel: w3264 -> [_ w3399 _]
                  tunnel: w3263 -> [_ w3398 _]
                  tunnel: w3262 -> [_ w3397 _]
                  tunnel: w3261 -> [_ w3396 _]
                  tunnel: w3260 -> [_ w3395 _]
                  tunnel: w3259 -> [_ w3394 _]
                  tunnel: w3258 -> [_ w3393 _]
                  tunnel: w3257 -> [_ w3392 _]
                  frame #0 {
                    w3272 = "/"
                    w3274 = "/"
                    w3275 = 2.0
                    w3282 = "\r"
                    n1996 = local read "DISP LAB01-2"() -> (w3371:T4)
                    n1997 = local read "DISP LAB01-1"() -> (w3372:T4)
                    n1998 = local read "DISP LAB02-1"() -> (w3370:T4)
                    n1999 = local read "DISP LAB03-2"() -> (w3367:T4)
                    n2000 = local read "DISP LAB02-2"() -> (w3369:T4)
                    n2001 = local read "DISP LAB03-1"() -> (w3368:T4)
                    n2002 = local read "DISP LAB04-2"() -> (w3365:T4)
                    n2003 = local read "DISP LAB04-1"() -> (w3366:T4)
                    n2004 = local read "DISP LAB05-1"() -> (w3364:T4)
                    n2005 = local read "DISP LAB05-2"() -> (w3363:T4)
                    n2006 = Unbundle(w3371) -> ("CYCLE"=w3355:dbl, "MINS"=w3354:dbl, "STATUS"=w3351:string)
                    n2007 = Unbundle(w3372) -> ("CYCLE"=w3360:dbl, "MINS"=w3359:dbl, "STATUS"=w3356:string)
                    n2008 = Unbundle(w3370) -> ("CYCLE"=w3348:dbl, "MINS"=w3347:dbl, "STATUS"=w3346:string)
                    n2009 = Unbundle(w3367) -> ("CYCLE"=w3335:dbl, "MINS"=w3334:dbl, "STATUS"=w3331:string)
                    n2010 = Unbundle(w3368) -> ("CYCLE"=w3340:dbl, "MINS"=w3339:dbl, "STATUS"=w3336:string)
                    n2011 = Unbundle(w3369) -> ("CYCLE"=w3345:dbl, "MINS"=w3344:dbl, "STATUS"=w3341:string)
                    n2012 = Unbundle(w3366) -> ("CYCLE"=w3330:dbl, "MINS"=w3329:dbl, "STATUS"=w3326:string)
                    n2013 = Unbundle(w3365) -> ("CYCLE"=w3325:dbl, "MINS"=w3324:dbl, "STATUS"=w3321:string)
                    n2014 = Unbundle(w3364) -> ("CYCLE"=w3320:dbl, "MINS"=w3319:dbl, "STATUS"=w3316:string)
                    n2015 = Unbundle(w3363) -> ("CYCLE"=w3362:dbl, "MINS"=w3361:dbl, "STATUS"=w3313:string)
                    n2016 = Number To Decimal String(number=w3348) -> (decimal integer string=w3350:string)  [unwired: 1 in]
                    n2017 = Number To Decimal String(number=w3345) -> (decimal integer string=w3343:string)  [unwired: 1 in]
                    n2018 = Number To Decimal String(number=w3340) -> (decimal integer string=w3338:string)  [unwired: 1 in]
                    n2019 = Number To Decimal String(number=w3355) -> (decimal integer string=w3353:string)  [unwired: 1 in]
                    n2020 = Number To Decimal String(number=w3335) -> (decimal integer string=w3333:string)  [unwired: 1 in]
                    n2021 = Number To Decimal String(number=w3360) -> (decimal integer string=w3358:string)  [unwired: 1 in]
                    n2022 = Number To Decimal String(number=w3362) -> (decimal integer string=w3315:string)  [unwired: 1 in]
                    n2023 = Number To Decimal String(number=w3330) -> (decimal integer string=w3328:string)  [unwired: 1 in]
                    n2024 = Number To Decimal String(number=w3325) -> (decimal integer string=w3323:string)  [unwired: 1 in]
                    n2025 = Number To Decimal String(number=w3320) -> (decimal integer string=w3318:string)  [unwired: 1 in]
                    n2026 = Number To Fractional String(number=w3347, precision (6)=w3275) -> (F-format string=w3349:string)  [unwired: 2 in]
                    n2027 = Number To Fractional String(number=w3334, precision (6)=w3275) -> (F-format string=w3332:string)  [unwired: 2 in]
                    n2028 = Number To Fractional String(number=w3344, precision (6)=w3275) -> (F-format string=w3342:string)  [unwired: 2 in]
                    n2029 = Number To Fractional String(number=w3339, precision (6)=w3275) -> (F-format string=w3337:string)  [unwired: 2 in]
                    n2030 = Number To Fractional String(number=w3324, precision (6)=w3275) -> (F-format string=w3322:string)  [unwired: 2 in]
                    n2031 = Number To Fractional String(number=w3329, precision (6)=w3275) -> (F-format string=w3327:string)  [unwired: 2 in]
                    n2032 = Number To Fractional String(number=w3354, precision (6)=w3275) -> (F-format string=w3352:string)  [unwired: 2 in]
                    n2033 = Number To Fractional String(number=w3319, precision (6)=w3275) -> (F-format string=w3317:string)  [unwired: 2 in]
                    n2034 = Number To Fractional String(number=w3359, precision (6)=w3275) -> (F-format string=w3357:string)  [unwired: 2 in]
                    n2035 = Number To Fractional String(number=w3361, precision (6)=w3275) -> (F-format string=w3314:string)  [unwired: 2 in]
                    n2036 = Concatenate Strings(w3274, w3333, w3274, w3332, w3274, w3331) -> (w3297:string)
                    n2037 = Concatenate Strings(w3274, w3328, w3274, w3327, w3274, w3326) -> (w3296:string)
                    n2038 = Concatenate Strings(w3274, w3323, w3274, w3322, w3274, w3321) -> (w3295:string)
                    n2039 = Concatenate Strings(w3274, w3318, w3274, w3317, w3274, w3316) -> (w3294:string)
                    n2040 = Concatenate Strings(w3274, w3315, w3274, w3314, w3274, w3313) -> (w3293:string)
                    n2041 = Concatenate Strings(w3274, w3358, w3274, w3357, w3274, w3356) -> (w3302:string)
                    n2042 = Concatenate Strings(w3274, w3338, w3274, w3337, w3274, w3336) -> (w3298:string)
                    n2043 = Concatenate Strings(w3274, w3353, w3274, w3352, w3274, w3351) -> (w3301:string)
                    n2044 = Concatenate Strings(w3274, w3350, w3274, w3349, w3274, w3346) -> (w3300:string)
                    n2045 = Concatenate Strings(w3274, w3343, w3274, w3342, w3274, w3341) -> (w3299:string)
                    n2046 = Concatenate Strings("LAB03-1", w3298, w3282) -> (w3288:string)
                    n2047 = Concatenate Strings("LAB02-1", w3300, w3282) -> (w3290:string)
                    n2048 = Concatenate Strings("LAB02-2", w3299, w3282) -> (w3289:string)
                    n2049 = Concatenate Strings("LAB04-2", w3295, w3282) -> (w3285:string)
                    n2050 = Concatenate Strings("LAB05-1", w3294, w3282) -> (w3286:string)
                    n2051 = Concatenate Strings("LAB04-1", w3296, w3282) -> (w3284:string)
                    n2052 = Concatenate Strings("LAB03-2", w3297, w3282) -> (w3283:string)
                    n2053 = Concatenate Strings("LAB05-2", w3293, w3282) -> (w3287:string)
                    n2054 = Concatenate Strings("LAB01-2", w3301, w3282) -> (w3291:string)
                    n2055 = Concatenate Strings("LAB01-1", w3302, w3282) -> (w3292:string)
                    n2056 = Concatenate Strings(w3292, w3291, w3290, w3289, w3288, w3283, w3284, w3285, w3286, w3287) -> (w3277:string)
                    n2057 = Concatenate Strings("PANEL", w3272, "CYCLES", w3272, "MINS", w3272, "STATUS", "\r", w3277) -> (w3276:string)
                    "MAIL REPORT" <- w3276
                  }
                  frame #1 {
                    w3401 = "END"
                    n2058 = local read "mail control"() -> (w3402:string)
                    n2059 = case shown="False" w3397 {
                      tunnel: w3402 -> [w3426 _]
                      tunnel: w3401 -> [w3425 _]
                      tunnel: [w3424 FALSE] -> w3387
                      frame False {
                        n2060 = Equal?(x=w3426, y=w3425) -> (x = y?=w3424:bool)
                      }
                      frame True {
                      }
                    }
                    n2061 = case shown="False" w3403 {
                      tunnel: w3402 -> [w3442 _]
                      tunnel: w3401 -> [w3441 _]
                      tunnel: [w3440 FALSE] -> w3391
                      frame False {
                        n2062 = Equal?(x=w3442, y=w3441) -> (x = y?=w3440:bool)
                      }
                      frame True {
                      }
                    }
                    n2063 = case shown="False" w3400 {
                      tunnel: w3402 -> [w3438 _]
                      tunnel: w3401 -> [w3437 _]
                      tunnel: [w3436 FALSE] -> w3390
                      frame False {
                        n2064 = Equal?(x=w3438, y=w3437) -> (x = y?=w3436:bool)
                      }
                      frame True {
                      }
                    }
                    n2065 = case shown="False" w3398 {
                      tunnel: w3402 -> [w3430 _]
                      tunnel: w3401 -> [w3429 _]
                      tunnel: [w3428 FALSE] -> w3388
                      frame False {
                        n2066 = Equal?(x=w3430, y=w3429) -> (x = y?=w3428:bool)
                      }
                      frame True {
                      }
                    }
                    n2067 = case shown="False" w3399 {
                      tunnel: w3402 -> [w3434 _]
                      tunnel: w3401 -> [w3433 _]
                      tunnel: [w3432 FALSE] -> w3389
                      frame False {
                        n2068 = Equal?(x=w3434, y=w3433) -> (x = y?=w3432:bool)
                      }
                      frame True {
                      }
                    }
                    n2069 = Or(x=w3389, y=w3388) -> (x .or. y?=w3380:bool)
                    n2070 = Or(x=w3391, y=w3390) -> (x .or. y?=w3381:bool)
                    n2071 = Or(x=w3381, y=w3380) -> (x .or. y?=w3376:bool)
                    n2072 = case shown="False" w3393 {
                      tunnel: w3402 -> [w3410 _]
                      tunnel: w3401 -> [w3409 _]
                      tunnel: [w3408 FALSE] -> w3382
                      frame False {
                        n2073 = Equal?(x=w3410, y=w3409) -> (x = y?=w3408:bool)
                      }
                      frame True {
                      }
                    }
                    n2074 = case shown="False" w3392 {
                      tunnel: w3402 -> [w3406 _]
                      tunnel: w3401 -> [w3405 _]
                      tunnel: [w3404 FALSE] -> w3386
                      frame False {
                        n2075 = Equal?(x=w3406, y=w3405) -> (x = y?=w3404:bool)
                      }
                      frame True {
                      }
                    }
                    n2076 = case shown="False" w3394 {
                      tunnel: w3402 -> [w3414 _]
                      tunnel: w3401 -> [w3413 _]
                      tunnel: [w3412 FALSE] -> w3383
                      frame False {
                        n2077 = Equal?(x=w3414, y=w3413) -> (x = y?=w3412:bool)
                      }
                      frame True {
                      }
                    }
                    n2078 = case shown="False" w3396 {
                      tunnel: w3402 -> [w3422 _]
                      tunnel: w3401 -> [w3421 _]
                      tunnel: [w3420 FALSE] -> w3385
                      frame False {
                        n2079 = Equal?(x=w3422, y=w3421) -> (x = y?=w3420:bool)
                      }
                      frame True {
                      }
                    }
                    n2080 = case shown="False" w3395 {
                      tunnel: w3402 -> [w3418 _]
                      tunnel: w3401 -> [w3417 _]
                      tunnel: [w3416 FALSE] -> w3384
                      frame False {
                        n2081 = Equal?(x=w3418, y=w3417) -> (x = y?=w3416:bool)
                      }
                      frame True {
                      }
                    }
                    n2082 = Or(x=w3385, y=w3384) -> (x .or. y?=w3379:bool)
                    n2083 = Or(x=w3383, y=w3382) -> (x .or. y?=w3378:bool)
                    n2084 = Or(x=w3386, y=w3387) -> (x .or. y?=w3374:bool)
                    n2085 = Or(x=w3379, y=w3378) -> (x .or. y?=w3377:bool)
                    n2086 = Or(x=w3376, y=w3377) -> (x .or. y?=w3375:bool)
                    n2087 = Or(x=w3375, y=w3374) -> (x .or. y?=w3373:bool)
                  }
                  frame #2 {
                    n2088 = local read "on loops"() -> (w3452:dbl)
                    n2089 = local read "jig cycle"() -> (w3449:dbl)
                    n2090 = Add(x=w3452, y=3.0) -> (x+y=w3450:dbl)
                    n2091 = Equal?(x=w3449, y=w3450) -> (x = y?=w3448:bool)
                    n2092 = And(x=w3447, y=w3448) -> (x .and. y?=w3446:bool)
                    n2093 = And(x=w3446, y=w3445) -> (x .and. y?=w3444:bool)
                    n2094 = case shown="True" w3444 {
                      tunnel: w3457 -> [_ w3462]
                      tunnel: w3456 -> [_ w3461]
                      tunnel: "Lab Panel Test Status" -> [_ w3460]
                      tunnel: w3454 -> [_ w3459]
                      tunnel: w3453 -> [_ w3458]
                      frame False {
                      }
                      frame True {
                        n2095 = stacked-sequence {
                          tunnel: w3462 -> [w3469 _]
                          tunnel: w3461 -> [w3468 _]
                          tunnel: w3460 -> [w3467 _]
                          tunnel: w3459 -> [w3466 _]
                          tunnel: w3458 -> [w3465 _]
                          frame #0 {
                            n2096 = disable-structure shown="Disabled" {
                              disable-tunnel: w3469 -> [w3475 _]
                              disable-tunnel: w3468 -> [w3474 _]
                              disable-tunnel: w3467 -> [w3473 _]
                              disable-tunnel: w3466 -> [w3472 _]
                              disable-tunnel: w3465 -> [w3471 _]
                              disable-tunnel: [w3470 _] -> w3464
                              frame Disabled {
                                n2097 = call "sub vi - send mail v3.vi"("TO:"=w3475, "message"=w3474, "subject"=w3473, "out going server"=w3472, "from"=w3471) -> ("error out"=w3470:errorcluster)  [unwired: 10 in]
                              }
                              frame Enabled {
                              }
                            }
                            n2098 = One Button Dialog(message="mail ") -> ()  [unwired: 1 in, 1 out]
                            n2099 = local write "Mail Report Error"(w3464) -> ()
                          }
                          frame #1 {
                            n2100 = local write "mail control"("") -> ()
                          }
                        }
                      }
                    }
                  }
                }
              }
            }
          }
          frame #16 {
            # "end test & close test files"
            n2101 = stacked-sequence {
              tunnel: w3486 -> [w3492 _ _ _ _ _ _ _ _ _]
              tunnel: w3487 -> [_ w3521 _ _ _ _ _ _ _ _]
              tunnel: w3485 -> [_ _ w3541 _ _ _ _ _ _ _]
              tunnel: w3484 -> [_ _ _ w3561 _ _ _ _ _ _]
              tunnel: w3483 -> [_ _ _ _ w3581 _ _ _ _ _]
              tunnel: w3482 -> [_ _ _ _ _ w3601 _ _ _ _]
              tunnel: w3481 -> [_ _ _ _ _ _ w3621 _ _ _]
              tunnel: w3480 -> [_ _ _ _ _ _ _ w3641 _ _]
              tunnel: w3479 -> [_ _ _ _ _ _ _ _ w3661 _]
              tunnel: w3478 -> [_ _ _ _ _ _ _ _ _ w3681]
              frame #0 {
                # "LAB01-1"
                n2102 = local read "DISP LAB01-1"() -> (w3490:T4)
                n2103 = local read "TDMS LAB01-1"() -> (w3488:refnum<k34>)
                n2104 = Unbundle(w3490) -> ("CYCLE"=w3491:dbl, "STATUS"=w3489:string)  [unwired: 1 out]
                n2105 = case shown="True" w3492 {
                  tunnel: w3491 -> [_ w3505]
                  tunnel: w3490 -> [w3495 w3504]
                  tunnel: w3489 -> [w3496 w3503]
                  tunnel: w3488 -> [w3493 w3502]
                  frame False {
                    n2106 = Equal?(x=w3496, y="RUN") -> (x = y?=w3494:bool)
                    n2107 = case shown="True" w3494 {
                      tunnel: w3495 -> [_ w3501]
                      tunnel: w3493 -> [_ w3498]
                      frame False {
                      }
                      frame True {
                        n2108 = TDMS Close(11:w3498) -> ()  [unwired: 1 in, 2 out]
                        n2109 = Bundle(cluster=w3501, "STATUS"="STOP") -> (w3500:T4)  [unwired: 2 in]
                        n2110 = local write "DISP LAB01-1"(w3500) -> ()
                      }
                    }
                  }
                  frame True {
                    n2111 = Not Equal?(x=w3503, y="RUN") -> (x != y?=w3506:bool)
                    n2112 = Greater?(x=w3505, y=2.0) -> (0:w3508:bool)
                    n2113 = And(x=w3508, y=w3506) -> (x .and. y?=w3507:bool)
                    n2114 = case shown="True" w3507 {
                      tunnel: w3504 -> [_ w3512]
                      tunnel: w3502 -> [_ w3511]
                      frame False {
                      }
                      frame True {
                        n2115 = stacked-sequence {
                          tunnel: w3512 -> [w3515 _ _]
                          tunnel: w3511 -> [_ w3516 _]
                          frame #0 {
                            n2116 = local write "mail control"("END") -> ()
                            n2117 = Bundle(cluster=w3515) -> (w3514:T4)  [unwired: 3 in]
                            n2118 = local write "DISP LAB01-1"(w3514) -> ()
                          }
                          frame #1 {
                            n2119 = TDMS Close(11:w3516) -> (0:w3517:errorcluster)  [unwired: 1 in, 1 out]
                            n2120 = local write "data file error"(w3517) -> ()
                          }
                          frame #2 {
                            n2121 = local write "RUN LAB01-1"(FALSE) -> ()
                            n2122 = call "Save data file to network drive v1.vi"("panel id"="LAB01-1") -> ("network file save error"=w3518:errorcluster)  [unwired: 9 in, 1 out]
                            n2123 = local write "data file error"(w3518) -> ()
                          }
                        }
                      }
                    }
                  }
                }
              }
              frame #1 {
                # "LAB01-2"
                n2124 = case shown="True" w3521 {
                  frame False {
                  }
                  frame True {
                    n2125 = local read "DISP LAB01-2"() -> (w3528:T4)
                    n2126 = local read "TDMS LAB01-2"() -> (w3527:refnum<k34>)
                    n2127 = Unbundle(w3528) -> ("CYCLE"=w3524:dbl, "STATUS"=w3529:string)  [unwired: 1 out]
                    n2128 = Not Equal?(x=w3529, y="RUN") -> (x != y?=w3523:bool)
                    n2129 = Greater?(x=w3524, y=2.0) -> (0:w3525:bool)
                    n2130 = And(x=w3525, y=w3523) -> (x .and. y?=w3522:bool)
                    n2131 = case shown="True" w3522 {
                      tunnel: w3528 -> [_ w3532]
                      tunnel: w3527 -> [_ w3531]
                      frame False {
                      }
                      frame True {
                        n2132 = stacked-sequence {
                          tunnel: w3532 -> [w3535 _ _]
                          tunnel: w3531 -> [_ w3537 _]
                          frame #0 {
                            n2133 = local write "mail control"("END") -> ()
                            n2134 = Bundle(cluster=w3535) -> (w3536:T4)  [unwired: 3 in]
                            n2135 = local write "RUN LAB01-2"(FALSE) -> ()
                            n2136 = local write "DISP LAB01-2"(w3536) -> ()
                          }
                          frame #1 {
                            n2137 = TDMS Close(11:w3537) -> (0:w3538:errorcluster)  [unwired: 1 in, 1 out]
                            n2138 = local write "data file error"(w3538) -> ()
                          }
                          frame #2 {
                            n2139 = call "Save data file to network drive v1.vi"("panel id"="LAB01-2") -> ("network file save error"=w3539:errorcluster)  [unwired: 9 in, 1 out]
                            n2140 = local write "data file error"(w3539) -> ()
                          }
                        }
                      }
                    }
                  }
                }
              }
              frame #2 {
                # "LAB02-1"
                n2141 = case shown="True" w3541 {
                  frame False {
                  }
                  frame True {
                    n2142 = local read "DISP LAB02-1"() -> (w3548:T4)
                    n2143 = Unbundle(w3548) -> ("CYCLE"=w3544:dbl, "STATUS"=w3549:string)  [unwired: 1 out]
                    n2144 = local read "TDMS LAB02-1"() -> (w3547:refnum<k34>)
                    n2145 = Not Equal?(x=w3549, y="RUN") -> (x != y?=w3543:bool)
                    n2146 = Greater?(x=w3544, y=2.0) -> (0:w3545:bool)
                    n2147 = And(x=w3545, y=w3543) -> (x .and. y?=w3542:bool)
                    n2148 = case shown="True" w3542 {
                      tunnel: w3548 -> [_ w3552]
                      tunnel: w3547 -> [_ w3551]
                      frame False {
                      }
                      frame True {
                        n2149 = stacked-sequence {
                          tunnel: w3552 -> [w3555 _ _]
                          tunnel: w3551 -> [_ w3557 _]
                          frame #0 {
                            n2150 = local write "mail control"("END") -> ()
                            n2151 = Bundle(cluster=w3555) -> (w3556:T4)  [unwired: 3 in]
                            n2152 = local write "RUN LAB02-1"(FALSE) -> ()
                            n2153 = local write "DISP LAB02-1"(w3556) -> ()
                          }
                          frame #1 {
                            n2154 = TDMS Close(11:w3557) -> (0:w3558:errorcluster)  [unwired: 1 in, 1 out]
                            n2155 = local write "data file error"(w3558) -> ()
                          }
                          frame #2 {
                            n2156 = call "Save data file to network drive v1.vi"("panel id"="LAB02-1") -> ("network file save error"=w3559:errorcluster)  [unwired: 9 in, 1 out]
                            n2157 = local write "data file error"(w3559) -> ()
                          }
                        }
                      }
                    }
                  }
                }
              }
              frame #3 {
                # "LAB02-2"
                n2158 = case shown="True" w3561 {
                  frame False {
                  }
                  frame True {
                    n2159 = local read "DISP LAB02-2"() -> (w3568:T4)
                    n2160 = local read "TDMS LAB02-2"() -> (w3567:refnum<k34>)
                    n2161 = Unbundle(w3568) -> ("CYCLE"=w3564:dbl, "STATUS"=w3569:string)  [unwired: 1 out]
                    n2162 = Not Equal?(x=w3569, y="RUN") -> (x != y?=w3563:bool)
                    n2163 = Greater?(x=w3564, y=2.0) -> (0:w3565:bool)
                    n2164 = And(x=w3565, y=w3563) -> (x .and. y?=w3562:bool)
                    n2165 = case shown="True" w3562 {
                      tunnel: w3568 -> [_ w3572]
                      tunnel: w3567 -> [_ w3571]
                      frame False {
                      }
                      frame True {
                        n2166 = stacked-sequence {
                          tunnel: w3572 -> [w3575 _ _]
                          tunnel: w3571 -> [_ w3577 _]
                          frame #0 {
                            n2167 = local write "mail control"("END") -> ()
                            n2168 = Bundle(cluster=w3575) -> (w3576:T4)  [unwired: 3 in]
                            n2169 = local write "RUN LAB02-2"(FALSE) -> ()
                            n2170 = local write "DISP LAB02-2"(w3576) -> ()
                          }
                          frame #1 {
                            n2171 = TDMS Close(11:w3577) -> (0:w3578:errorcluster)  [unwired: 1 in, 1 out]
                            n2172 = local write "data file error"(w3578) -> ()
                          }
                          frame #2 {
                            n2173 = call "Save data file to network drive v1.vi"("panel id"="LAB02-2") -> ("network file save error"=w3579:errorcluster)  [unwired: 9 in, 1 out]
                            n2174 = local write "data file error"(w3579) -> ()
                          }
                        }
                      }
                    }
                  }
                }
              }
              frame #4 {
                # "LAB03-1"
                n2175 = case shown="True" w3581 {
                  frame False {
                  }
                  frame True {
                    n2176 = local read "DISP LAB03-1"() -> (w3588:T4)
                    n2177 = local read "TDMS LAB03-1"() -> (w3587:refnum<k34>)
                    n2178 = Unbundle(w3588) -> ("CYCLE"=w3584:dbl, "STATUS"=w3589:string)  [unwired: 1 out]
                    n2179 = Not Equal?(x=w3589, y="RUN") -> (x != y?=w3583:bool)
                    n2180 = Greater?(x=w3584, y=2.0) -> (0:w3585:bool)
                    n2181 = And(x=w3585, y=w3583) -> (x .and. y?=w3582:bool)
                    n2182 = case shown="True" w3582 {
                      tunnel: w3588 -> [_ w3592]
                      tunnel: w3587 -> [_ w3591]
                      frame False {
                      }
                      frame True {
                        n2183 = stacked-sequence {
                          tunnel: w3592 -> [w3595 _ _]
                          tunnel: w3591 -> [_ w3597 _]
                          frame #0 {
                            n2184 = local write "mail control"("END") -> ()
                            n2185 = Bundle(cluster=w3595) -> (w3596:T4)  [unwired: 3 in]
                            n2186 = local write "RUN LAB03-1"(FALSE) -> ()
                            n2187 = local write "DISP LAB03-1"(w3596) -> ()
                          }
                          frame #1 {
                            n2188 = TDMS Close(11:w3597) -> (0:w3598:errorcluster)  [unwired: 1 in, 1 out]
                            n2189 = local write "data file error"(w3598) -> ()
                          }
                          frame #2 {
                            n2190 = call "Save data file to network drive v1.vi"("panel id"="LAB03-1") -> ("network file save error"=w3599:errorcluster)  [unwired: 9 in, 1 out]
                            n2191 = local write "data file error"(w3599) -> ()
                          }
                        }
                      }
                    }
                  }
                }
              }
              frame #5 {
                # "LAB03-2"
                n2192 = case shown="True" w3601 {
                  frame False {
                  }
                  frame True {
                    n2193 = local read "DISP LAB03-2"() -> (w3608:T4)
                    n2194 = Unbundle(w3608) -> ("CYCLE"=w3604:dbl, "STATUS"=w3609:string)  [unwired: 1 out]
                    n2195 = local read "TDMS LAB03-2"() -> (w3607:refnum<k34>)
                    n2196 = Not Equal?(x=w3609, y="RUN") -> (x != y?=w3603:bool)
                    n2197 = Greater?(x=w3604, y=2.0) -> (0:w3605:bool)
                    n2198 = And(x=w3605, y=w3603) -> (x .and. y?=w3602:bool)
                    n2199 = case shown="True" w3602 {
                      tunnel: w3608 -> [_ w3612]
                      tunnel: w3607 -> [_ w3611]
                      frame False {
                      }
                      frame True {
                        n2200 = stacked-sequence {
                          tunnel: w3612 -> [w3615 _ _]
                          tunnel: w3611 -> [_ w3617 _]
                          frame #0 {
                            n2201 = local write "mail control"("END") -> ()
                            n2202 = Bundle(cluster=w3615) -> (w3616:T4)  [unwired: 3 in]
                            n2203 = local write "RUN LAB03-2"(FALSE) -> ()
                            n2204 = local write "DISP LAB03-2"(w3616) -> ()
                          }
                          frame #1 {
                            n2205 = TDMS Close(11:w3617) -> (0:w3618:errorcluster)  [unwired: 1 in, 1 out]
                            n2206 = local write "data file error"(w3618) -> ()
                          }
                          frame #2 {
                            n2207 = call "Save data file to network drive v1.vi"("panel id"="LAB03-2") -> ("network file save error"=w3619:errorcluster)  [unwired: 9 in, 1 out]
                            n2208 = local write "data file error"(w3619) -> ()
                          }
                        }
                      }
                    }
                  }
                }
              }
              frame #6 {
                # "LAB04-1"
                n2209 = case shown="True" w3621 {
                  frame False {
                  }
                  frame True {
                    n2210 = local read "DISP LAB04-1"() -> (w3628:T4)
                    n2211 = Unbundle(w3628) -> ("CYCLE"=w3624:dbl, "STATUS"=w3629:string)  [unwired: 1 out]
                    n2212 = local read "TDMS LAB04-1"() -> (w3627:refnum<k34>)
                    n2213 = Not Equal?(x=w3629, y="RUN") -> (x != y?=w3623:bool)
                    n2214 = Greater?(x=w3624, y=2.0) -> (0:w3625:bool)
                    n2215 = And(x=w3625, y=w3623) -> (x .and. y?=w3622:bool)
                    n2216 = case shown="True" w3622 {
                      tunnel: w3628 -> [_ w3632]
                      tunnel: w3627 -> [_ w3631]
                      frame False {
                      }
                      frame True {
                        n2217 = stacked-sequence {
                          tunnel: w3632 -> [w3635 _ _]
                          tunnel: w3631 -> [_ w3637 _]
                          frame #0 {
                            n2218 = local write "mail control"("END") -> ()
                            n2219 = Bundle(cluster=w3635) -> (w3636:T4)  [unwired: 3 in]
                            n2220 = local write "RUN LAB04-1"(FALSE) -> ()
                            n2221 = local write "DISP LAB04-1"(w3636) -> ()
                          }
                          frame #1 {
                            n2222 = TDMS Close(11:w3637) -> (0:w3638:errorcluster)  [unwired: 1 in, 1 out]
                            n2223 = local write "data file error"(w3638) -> ()
                          }
                          frame #2 {
                            n2224 = call "Save data file to network drive v1.vi"("panel id"="LAB04-1") -> ("network file save error"=w3639:errorcluster)  [unwired: 9 in, 1 out]
                            n2225 = local write "data file error"(w3639) -> ()
                          }
                        }
                      }
                    }
                  }
                }
              }
              frame #7 {
                # "LAB04-2"
                n2226 = case shown="True" w3641 {
                  frame False {
                  }
                  frame True {
                    n2227 = local read "DISP LAB04-2"() -> (w3648:T4)
                    n2228 = Unbundle(w3648) -> ("CYCLE"=w3644:dbl, "STATUS"=w3649:string)  [unwired: 1 out]
                    n2229 = Not Equal?(x=w3649, y="RUN") -> (x != y?=w3643:bool)
                    n2230 = local read "TDMS LAB04-2"() -> (w3647:refnum<k34>)
                    n2231 = Greater?(x=w3644, y=2.0) -> (0:w3645:bool)
                    n2232 = And(x=w3645, y=w3643) -> (x .and. y?=w3642:bool)
                    n2233 = case shown="True" w3642 {
                      tunnel: w3648 -> [_ w3652]
                      tunnel: w3647 -> [_ w3651]
                      frame False {
                      }
                      frame True {
                        n2234 = stacked-sequence {
                          tunnel: w3652 -> [w3655 _ _]
                          tunnel: w3651 -> [_ w3657 _]
                          frame #0 {
                            n2235 = local write "mail control"("END") -> ()
                            n2236 = Bundle(cluster=w3655) -> (w3656:T4)  [unwired: 3 in]
                            n2237 = local write "RUN LAB04-2"(FALSE) -> ()
                            n2238 = local write "DISP LAB04-2"(w3656) -> ()
                          }
                          frame #1 {
                            n2239 = TDMS Close(11:w3657) -> (0:w3658:errorcluster)  [unwired: 1 in, 1 out]
                            n2240 = local write "data file error"(w3658) -> ()
                          }
                          frame #2 {
                            n2241 = call "Save data file to network drive v1.vi"("panel id"="LAB04-2") -> ("network file save error"=w3659:errorcluster)  [unwired: 9 in, 1 out]
                            n2242 = local write "data file error"(w3659) -> ()
                          }
                        }
                      }
                    }
                  }
                }
              }
              frame #8 {
                # "LAB05-1"
                n2243 = case shown="True" w3661 {
                  frame False {
                  }
                  frame True {
                    n2244 = local read "DISP LAB05-1"() -> (w3668:T4)
                    n2245 = Unbundle(w3668) -> ("CYCLE"=w3664:dbl, "STATUS"=w3669:string)  [unwired: 1 out]
                    n2246 = Not Equal?(x=w3669, y="RUN") -> (x != y?=w3663:bool)
                    n2247 = local read "TDMS LAB05-1"() -> (w3667:refnum<k34>)
                    n2248 = Greater?(x=w3664, y=2.0) -> (0:w3665:bool)
                    n2249 = And(x=w3665, y=w3663) -> (x .and. y?=w3662:bool)
                    n2250 = case shown="True" w3662 {
                      tunnel: w3668 -> [_ w3672]
                      tunnel: w3667 -> [_ w3671]
                      frame False {
                      }
                      frame True {
                        n2251 = stacked-sequence {
                          tunnel: w3672 -> [w3675 _ _]
                          tunnel: w3671 -> [_ w3677 _]
                          frame #0 {
                            n2252 = local write "mail control"("END") -> ()
                            n2253 = Bundle(cluster=w3675) -> (w3676:T4)  [unwired: 3 in]
                            n2254 = local write "RUN LAB05-1"(FALSE) -> ()
                            n2255 = local write "DISP LAB05-1"(w3676) -> ()
                          }
                          frame #1 {
                            n2256 = TDMS Close(11:w3677) -> (0:w3678:errorcluster)  [unwired: 1 in, 1 out]
                            n2257 = local write "data file error"(w3678) -> ()
                          }
                          frame #2 {
                            n2258 = call "Save data file to network drive v1.vi"("panel id"="LAB05-1") -> ("network file save error"=w3679:errorcluster)  [unwired: 9 in, 1 out]
                            n2259 = local write "data file error"(w3679) -> ()
                          }
                        }
                      }
                    }
                  }
                }
              }
              frame #9 {
                # "LAB05-2"
                n2260 = case shown="True" w3681 {
                  frame False {
                  }
                  frame True {
                    n2261 = local read "DISP LAB05-2"() -> (w3688:T4)
                    n2262 = Unbundle(w3688) -> ("CYCLE"=w3684:dbl, "STATUS"=w3689:string)  [unwired: 1 out]
                    n2263 = Not Equal?(x=w3689, y="RUN") -> (x != y?=w3683:bool)
                    n2264 = local read "TDMS LAB05-2"() -> (w3687:refnum<k34>)
                    n2265 = Greater?(x=w3684, y=2.0) -> (0:w3685:bool)
                    n2266 = And(x=w3685, y=w3683) -> (x .and. y?=w3682:bool)
                    n2267 = case shown="True" w3682 {
                      tunnel: w3688 -> [_ w3692]
                      tunnel: w3687 -> [_ w3691]
                      frame False {
                      }
                      frame True {
                        n2268 = stacked-sequence {
                          tunnel: w3692 -> [w3695 _ _]
                          tunnel: w3691 -> [_ w3697 _]
                          frame #0 {
                            n2269 = local write "mail control"("END") -> ()
                            n2270 = Bundle(cluster=w3695) -> (w3696:T4)  [unwired: 3 in]
                            n2271 = local write "RUN LAB05-2"(FALSE) -> ()
                            n2272 = local write "DISP LAB05-2"(w3696) -> ()
                          }
                          frame #1 {
                            n2273 = TDMS Close(11:w3697) -> (0:w3698:errorcluster)  [unwired: 1 in, 1 out]
                            n2274 = local write "data file error"(w3698) -> ()
                          }
                          frame #2 {
                            n2275 = call "Save data file to network drive v1.vi"("panel id"="LAB05-2") -> ("network file save error"=w3699:errorcluster)  [unwired: 9 in, 1 out]
                            n2276 = local write "data file error"(w3699) -> ()
                          }
                        }
                      }
                    }
                  }
                }
              }
            }
            n2277 = local read "Network Directory"() -> (w3477:path)
            n2278 = global write "Global 1.vi" "Network Drive"(w3477) -> ()
          }
        }
        n2279 = node-c288() -> ()  [unwired: 1 in, 1 out]
        "loops" <- w157
        "stop2" <- "stop"
      }
      n2280 = node-c288(w134) -> ()  [unwired: 1 out]
    }
  }
